vi "myRIO_BRig_RT_v0,60.vi"() -> ()   [LabVIEW 2014]
uses:
  myRIO_BRig_RT__Case_Exp_stateList.ctl
  myRIO_BRig_RT__Case_NonExp_stateList.ctl
  <vilib>/Platform/TimedLoop/XDataNode/timing_clust.ctl
  <vilib>/Platform/TimedLoop/XDataNode/nitl_modes.ctl
  <vilib>/Platform/TimedLoop/XDataNode/wakeup.ctl
  <vilib>/WebDAVClient/Advanced/SessionHandle.ctl
  <vilib>/myRIO/Common/Instrument Driver Framework/myRIO v1.0/UART/vis/myRIO v1.0 Close UART.vi
  <vilib>/FPGAPlugInAG/myRIO-1900/niLvFpga_Open_myRIO-1900.vi
  <vilib>/rvi/interface/common/dynamic/niFpgaDynamicAddResources.vi
  <vilib>/Utility/error.llb/Error Cluster From Error Code.vi
  <vilib>/rvi/errors/niLvFpgaAdjustHostInterfaceError.vi
  <vilib>/FPGAPlugInAG/Dynamic/niLvFpga_Close_Dynamic.vi
  <vilib>/myRIO/Common/Instrument Driver Framework/Utilities/vis/FPGA Ref Manager.vi
  <vilib>/myRIO/Common/Instrument Driver Framework/myRIO v1.0/myRIO v1.0 Reset FPGA.vi
  <vilib>/myRIO/Common/Instrument Driver Framework/myRIO v1.0/IRQ/vis/myRIO v1.0 IRQ Info FGV.vi
  <vilib>/myRIO/Common/Instrument Driver Framework/myRIO v1.0/IRQ/vis/myRIO v1.0 Timer IRQ Info FGV.vi
  <vilib>/myRIO/Common/Instrument Driver Framework/myRIO v1.0/IRQ/vis/myRIO v1.0 ISR Agent.vi
  <vilib>/rvi/interface/nirviOpenFPGA/nirviOpenFPGA.xnode
  myRIO_BRig_FPGA_v3,51__build.lvbitx
  myRIO_BRig_FPGA_v3,51.vi
  <vilib>/rvi/interface/nirviReadWriteControl/nirviReadWriteControl.xnode
  <vilib>/Platform/TimedLoop/XDataNode/XDataNode.xnode
  <vilib>/rvi/interface/nirviCloseFPGA/nirviCloseFPGA.xnode
  <vilib>/Platform/TimedLoop/XDataNode/XDNodeRunTimeDep.lvlib
  <vilib>/rvi/interface/Simulation/niFpgaSimulationCallBeginRW.vi
  <vilib>/myRIO/Instrument Drivers/Utilities/Utilities.lvlib
  <vilib>/WebDAVClient/NI_WebDAV.lvlib
  NiFpgaLv.dll
panel:
  out "SolenoidReward":bool
  in  "SolenoidProbability_L":u16=50 caption="Reward Time [ms]" min=1 max=1000 step=1
  in  "SolenoidProbability_R":u16=50 caption="Reward Time [ms]" min=1 max=1000 step=1
  out "output_PortA":dbl
  out "error out 4":errorcluster
  in  "laser_power_step":dbl
  in  "laser_power_max":dbl
  in  "Recording_p2":bool
  in  "Recording":bool
  out "error out 3":errorcluster
  out "error out 2":errorcluster
  in  "laser_power_min":dbl
  in  "f_millisec2count":dbl=159.0
  in  "laser_Tshutter":dbl=2.0
  in  "laser_Freq":dbl=10.0
  in  "laser_Tpeak":dbl=2.0
  in  "laser_duration":u16
  out "error out":errorcluster
  in  "LC_Cue1_All_Count":u16
  in  "LC_Cue1_First_Count":u16
  in  "LC_Cue1_All_delayOpt":bool
  in  "LC_ENL1_All_delayOpt":bool
  in  "LC_ENL1_All_Count":u16
  in  "LC_ENL1_First_Count":u16
  in  "LC_Cue1_First_delayOpt":bool
  in  "LC_ENL1_First_delayOpt":bool
  in  "Tcycle_Cue_max":u16=1000 caption="Max [ms]" min=5 max=5000 step=5
  in  "Tcycle_Cue_min":u16=1000 caption="Min [ms]" min=5 max=5000 step=5
  in  "SendData":bool
  out "cSpout":enum16{"Left", "Right"}(ring) caption="Left or Right Spout"
  out "A4":u32 caption="LickCounter_Right"
  out "A2":u32 caption="LickCounter_Left"
  in  "laserResponse_wrong_LED":bool
  out "error_initTrial":errorcluster
  out "error_Selection_pre":errorcluster
  out "error_Selection":errorcluster
  out "SelectWrong":bool
  out "SelectReward":bool
  in  "Left(F)_or_Right(T)":bool
  in  "ignoreWrong":bool
  in  "SelectionState":bool
  in  "laserResponse_wrong":bool
  in  "laserResponse_reward":bool
  in  "laserResponse_reward_LED":bool
  out "nRewards_Right":u16 caption="# Rewards Total (Right)"
  out "nRewards_Left":u16 caption="# Rewards Total (Left)"
  out "nRewards_cur":u16 caption="# Rewards in Current Block"
  out "TpB_target":u16 caption="Target Trials Per Block"
  out "cState_NonExp":T1 caption="NonExperimental State"
  out "iBlock":u16 caption="Current Block"
  out "cState":T2 caption="Experimental State"
  out "iTrial":u16 caption="Current Trial"
  in  "warmupType":u8(slide) max=2 step=1 scale=0.0..2.0
  in  "TestConnection":bool
  in  "warmup":bool caption="WarmUp"
  in  "Host Filename Prefix":string="Exp1_TM2"
  out "Connected To Host?":bool
  in  "Host Password":string="sabalab"
  in  "Host UserName":string="Test2"
  in  "sp_RightSpout":u16(slide)=2 max=2 step=1 scale=0.0..2.0
  in  "sp_LeftSpout":u16(slide)=2 max=2 step=1 scale=0.0..2.0
  in  "BUR_max":u16 caption="Count Reward Structure  (0 = off)"
  in  "LC_Wrong_Probability":u16
  in  "LC_Wrong_Trial":u16(slide) max=2 step=1 scale=0.0..2.0
  in  "LC_Wrong_Block":u16(slide) max=2 step=1 scale=0.0..2.0
  in  "LC_Wrong_OnOff":bool
  in  "LC_Reward_Probability":u16
  in  "LC_Reward_Trial":u16(slide) max=2 step=1 scale=0.0..2.0
  in  "LC_Reward_Block":u16(slide) max=2 step=1 scale=0.0..2.0
  in  "LC_Reward_OnOff":bool
  in  "LC_Cue1_All_Probability":u16
  in  "LC_Cue1_All_Block":u16(slide) max=2 step=1 scale=0.0..2.0
  in  "LC_Cue1_All_OnOff":bool
  in  "LC_Cue1_First_Probability":u16
  in  "LC_Cue1_First_Block":u16(slide) max=2 step=1 scale=0.0..2.0
  in  "LC_Cue1_First_OnOff":bool
  in  "LC_ENL1_All_Probability":u16 max=100 step=1
  in  "LC_ENL1_All_Block":u16(slide) max=2 step=1 scale=0.0..2.0
  in  "LC_ENL1_All_OnOff":bool
  in  "LC_ENL1_First_Probability":u16 max=100 step=1
  in  "LC_ENL1_First_Block":u16(slide) max=2 step=1 scale=0.0..2.0
  in  "Tcycle_Timeout":u16=1000 caption="Timeout Time [ms]" min=10 max=10000 step=1
  in  "Tcycle_Wrong":u16=1000 caption="Wrong Time [ms]" min=10 max=10000 step=1
  in  "Tcycle_Selection":u16=1000 caption="Answer Time [ms]" min=1 max=10000 step=1
  in  "Tcycle_RewardPost":u16=1000 caption="Consumption Time [ms]" min=250 max=10000 step=250
  in  "Tcycle_Reward_L":u16=500 caption="Reward Time [ms]" min=1 max=1000 step=1
  in  "Tcycle_Reward_R":u16=500 caption="Reward Time [ms]" min=1 max=1000 step=1
  in  "TpB_Max_R":u16=4 caption="Max TrialsPerBlock" min=1 max=12 step=1
  in  "TpB_Min_R":u16=4 caption="Min TrialsPerBlock" min=1 max=12 step=1
  in  "TpB_Max_L":u16=4 caption="Max TrialsPerBlock" min=1 max=12 step=1
  in  "TpB_Min_L":u16=4 caption="Min TrialsPerBlock" min=1 max=12 step=1
  in  "BUR_min":u16 caption="Count Reward Structure  (0 = off)"
  in  "TrialUntilReward":bool caption="Ignore Wrong \nSelection"
  in  "CueCycles":u16=1 caption="Cue Structure" min=1 max=1 step=1
  in  "MTrig_Laser_Tcycle":u16=10 caption="Time [ms]"
  in  "MTrig_Laser_trig":bool
  in  "MTrig_Audio_trig__R":bool caption="Trigger Audio"
  in  "MTrig_Audio_trig__L":bool caption="Trigger Audio"
  in  "RewCalib_Trig_R":bool caption="Calibrate_R"
  in  "RewCalib_Trig_L":bool caption="Calibrate_L"
  in  "MTrig_Solenoid_Tcycle__R":u16=300 caption="Time [ms]"
  in  "MTrig_Solenoid_Tcycle__L":u16=300 caption="Time [ms]"
  in  "MTrig_Solenoid_trig__R":bool caption="Solenoid"
  in  "MTrig_Solenoid_trig__L":bool caption="Solenoid"
  in  "STOP_abort":bool caption="Stop LabView\n(Stops myRio and FPGA)"
  in  "STOP_endBlock":bool caption="Stop Experiment\n@ End of Block"
  in  "STOP_endTrial":bool caption="Stop Experiment\n@ End of Trial"
  in  "START":bool caption="Start Experiment"
  in  "Tcycle_CuePenalty":u16=1000 caption="Penalty [ms]" min=1 max=10000 step=1
  in  "Audio_Amp__R":u16=100 caption="Amp"
  in  "Audio_Freq__R":u8=5 caption="Freq [kHz]" max=14 step=1
  in  "Audio_Amp__L":u16=100 caption="Amp"
  in  "Audio_Freq__L":u8=5 caption="Freq [kHz]" max=14 step=1
  in  "LC_Wrong_Tdelay":u16
  in  "LC_Cue1_All_Tdelay":u16
  in  "LC_ENL1_All_Tdelay":u16
  in  "LC_Reward_Tdelay":u16
  in  "LC_Cue1_First_Tdelay":u16
  in  "LC_ENL1_First_Tdelay":u16
  in  "LC_ENL1_First_OnOff":bool
  in  "Tcycle_ENLPenalty":u16=100 caption="Penalty [ms]" min=10 max=10000 step=10
  in  "Tcycle_ENL_max":u16=1000 caption="Max [ms]" min=250 max=10000 step=250
  in  "Tcycle_ENL_min":u16=1000 caption="Min [ms]" min=250 max=10000 step=250
  # "Manual Control"
  # "Task Structure"
  # "Task Timing"
  # "Laser Control\n\n                                                    On/Off      Block        Probability [%]   Delay [ms]                              Count"
  # "Manual Solenoid Trigger\nLeft              Right"
  # "Master Structure"
  # "Enforced NonLick"
  # "Enforced NonLick 1"
  # "from end"
  # "Time = Cue Min"
  # "Min\n \n  \nMax"
  # "Switch Trial"
  # "from start"
  # "(1) = Switching\n(2) = Two Choice"
  # "from end"
  # "NonSwitch Trials"
  # "Cue"
  # "from start"
  # "Cue 1"
  # "from end"
  # "Switch Trial"
  # "from start"
  # "Min"
  # "Max"
  # "from end"
  # "NonSwitch Trials"
  # "Trial Per Block Structure\n       Left                    Right"
  # "from start"
  # "Spout Selection Control"
  # "Manual Speaker Trigger\nLeft              Right"
  # "Selection Reward"
  # "Answer Time\n         [ms]\n\n  \nWrong Choice Penalty\n         [ms]\n \n \nChoice Timeout Penalty\n         [ms]"
  # "Selection Wrong"
  # "Cue Control"
  # "Left              Right"
  # "State"
  # "Manual Laser Trigger"
  # "Freq [kHz]\n \n \nAmp\n \n\n \n\nSpeaker\nSetting"
  # "Reward Control\n                 Left              Right"
  # "Min = 1\nMax = 32k"
  # "Reward Time\n         [ms]\n\nWater Prob"
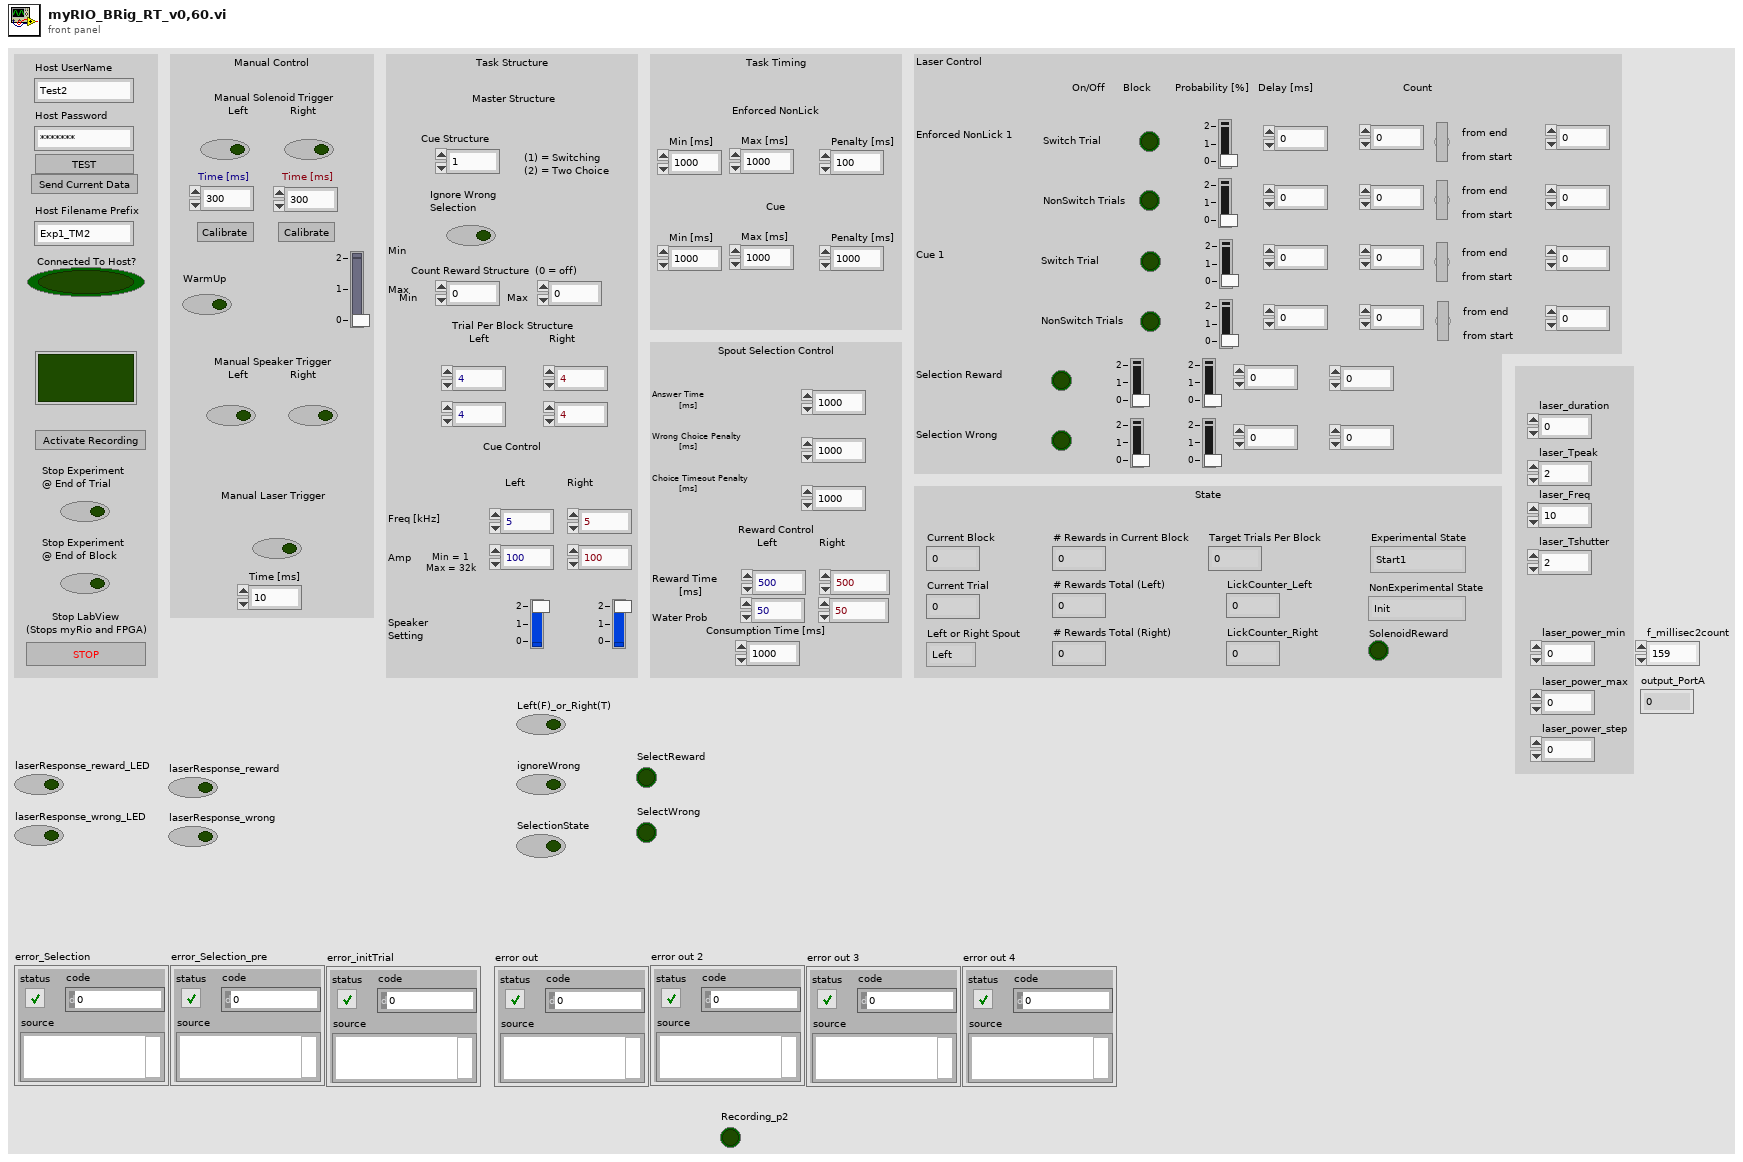
[diagram p1: front panel]
types:
  T1 = typedef "myRIO_BRig_RT__Case_NonExp_stateList.ctl" = enum16{"Init", "UploadSettings_pre", "UploadSettings_Read_dataExp", "UploadSettings_dataExp_1", "UploadSettings_Read_dataLC", "UploadSettings_dataLC_1", "UploadSettings_dataLC_2", "UploadSettings_Read_dataMTrig", "UploadSettings_dataMTrig_1", "UploadSettings_post", "Idle_pre", "IdleEmpty", "IdleEmpty2", "IdleEmpty3", "IdleEmpty4", "Idle", "Idle_2", "Idle_3", "Idle_4", "Idle_post", "Cue_pre__pre", "Cue_pre", "Cue", "Cue_post", "RewardCalibration_pre", "DispenseWater_pre__pre", "DispenseWater_pre", "DispenseWater", "DispenseWater_post", "TestConnection", "SendData", "End"}
  T2 = typedef "myRIO_BRig_RT__Case_Exp_stateList.ctl" = enum16{"Start1", "Start2", "Start3", "saveSettings1", "saveSettings2", "saveSettings3", "saveSettings4_LC_ENL", "saveSettings5_LC_Cue", "saveSettings6_LC_Other", "setSettings_Audio", "setSettings_Laser", "initBlock_pre", "initBlock", "initBlock2", "initBlock_post", "initTrial_pre", "initTrial", "initTrial2", "initTrial3", "initTrial4", "initTrial_LC_ENL1", "initTrial_LC_Cue1", "initTrial_post", "ENL1_pre", "ENL1", "ENL1_post", "ENL1Penalty_pre", "ENL1Penalty", "ENL2_pre", "ENL2", "ENL2Penalty_pre", "ENL2Penalty", "Cue1_pre", "Cue1", "Cue1_post", "Cue1Penalty_pre", "Cue1Penalty", "Cue2_pre", "Cue2", "Cue2Penalty_pre", "Cue2Penalty", "Selection_pre", "Selection", "Select_post", "SelectReward_pre", "SelectReward", "SelectRewardPost_pre", "SelectRewardPost", "SelectWrong_pre", "SelectWrong", "SelectWrong_post", "SelectTimeout_pre", "SelectTimeout", "SelectTimeout_post", "endTrial_pre", "endTrial1", "endTrial2", "endTrial3", "endTrial_post", "endBlock_pre", "endBlock", "endBlock_post", "endExp", "commConnect", "commUpload_pre", "commUpload_dataBlock", "commUpload_dataCurrent", "commUpload_dataExp", "commUpload_dataLC", "commUpload_dataTrial", "commUpload_post", "saveData_pre", "saveData_dataBlock", "saveData_dataCurrent", "saveData_dataExp", "saveData_dataLC", "saveData_dataTrial", "saveData_post", "empty_endBlock1", "empty_endBlock2", "empty_endTrial1", "empty_endTrial2", "empty_endTrial3", "empty_endTrial4", "empty_endTrial5"}
  T3 = typedef "XDNodeRunTimeDep.lvlib/timing_clust.ctl" = cluster{"Expected End [f-1]":u64, "Actual End [f-1]":u64, "Finished Late? [f-1]":bool, "Expected End [i-1]":u64, "Actual End [i-1]":u64, "Finished Late? [i-1]":bool, "Expected Start [i]":u64, "Actual Start [i]":u64, "Expected Start [f]":u64, "Actual Start [f]":u64, "Source Name":string, "Structure Name":string, "Period":i64, "Deadline":i64, "Offset":i64, "Start":i64, "Priority":i32, "Timeout":i32, "Mode":T4, "Wakeup Reason":T5, "Error":errorcluster, "Source Type":string, "Secondary Source Type":string, "Global End Time":u64, "Global Start Time":u64, "Frame Duration":u64, "Iteration Duration":u64, "Assigned CPU":i32, "I/O Scan Engine Mode":u32}
  T4 = typedef "XDNodeRunTimeDep.lvlib/nitl_modes.ctl" = enum32{"No Change", "Process missed periods, maintain original phase", "Discard missed periods, maintain original phase", "Process missed periods, ignore original phase", "Discard missed periods, ignore original phase"}
  T5 = typedef "XDNodeRunTimeDep.lvlib/wakeup.ctl" = enum32{"Normal", "Aborted", "Asynchronous wakeup", "Timing source error", "Timed loop error", "Timeout"}
  T6 = typedef "NI_WebDAV.lvlib/SessionHandle.ctl" = refnum<k1>
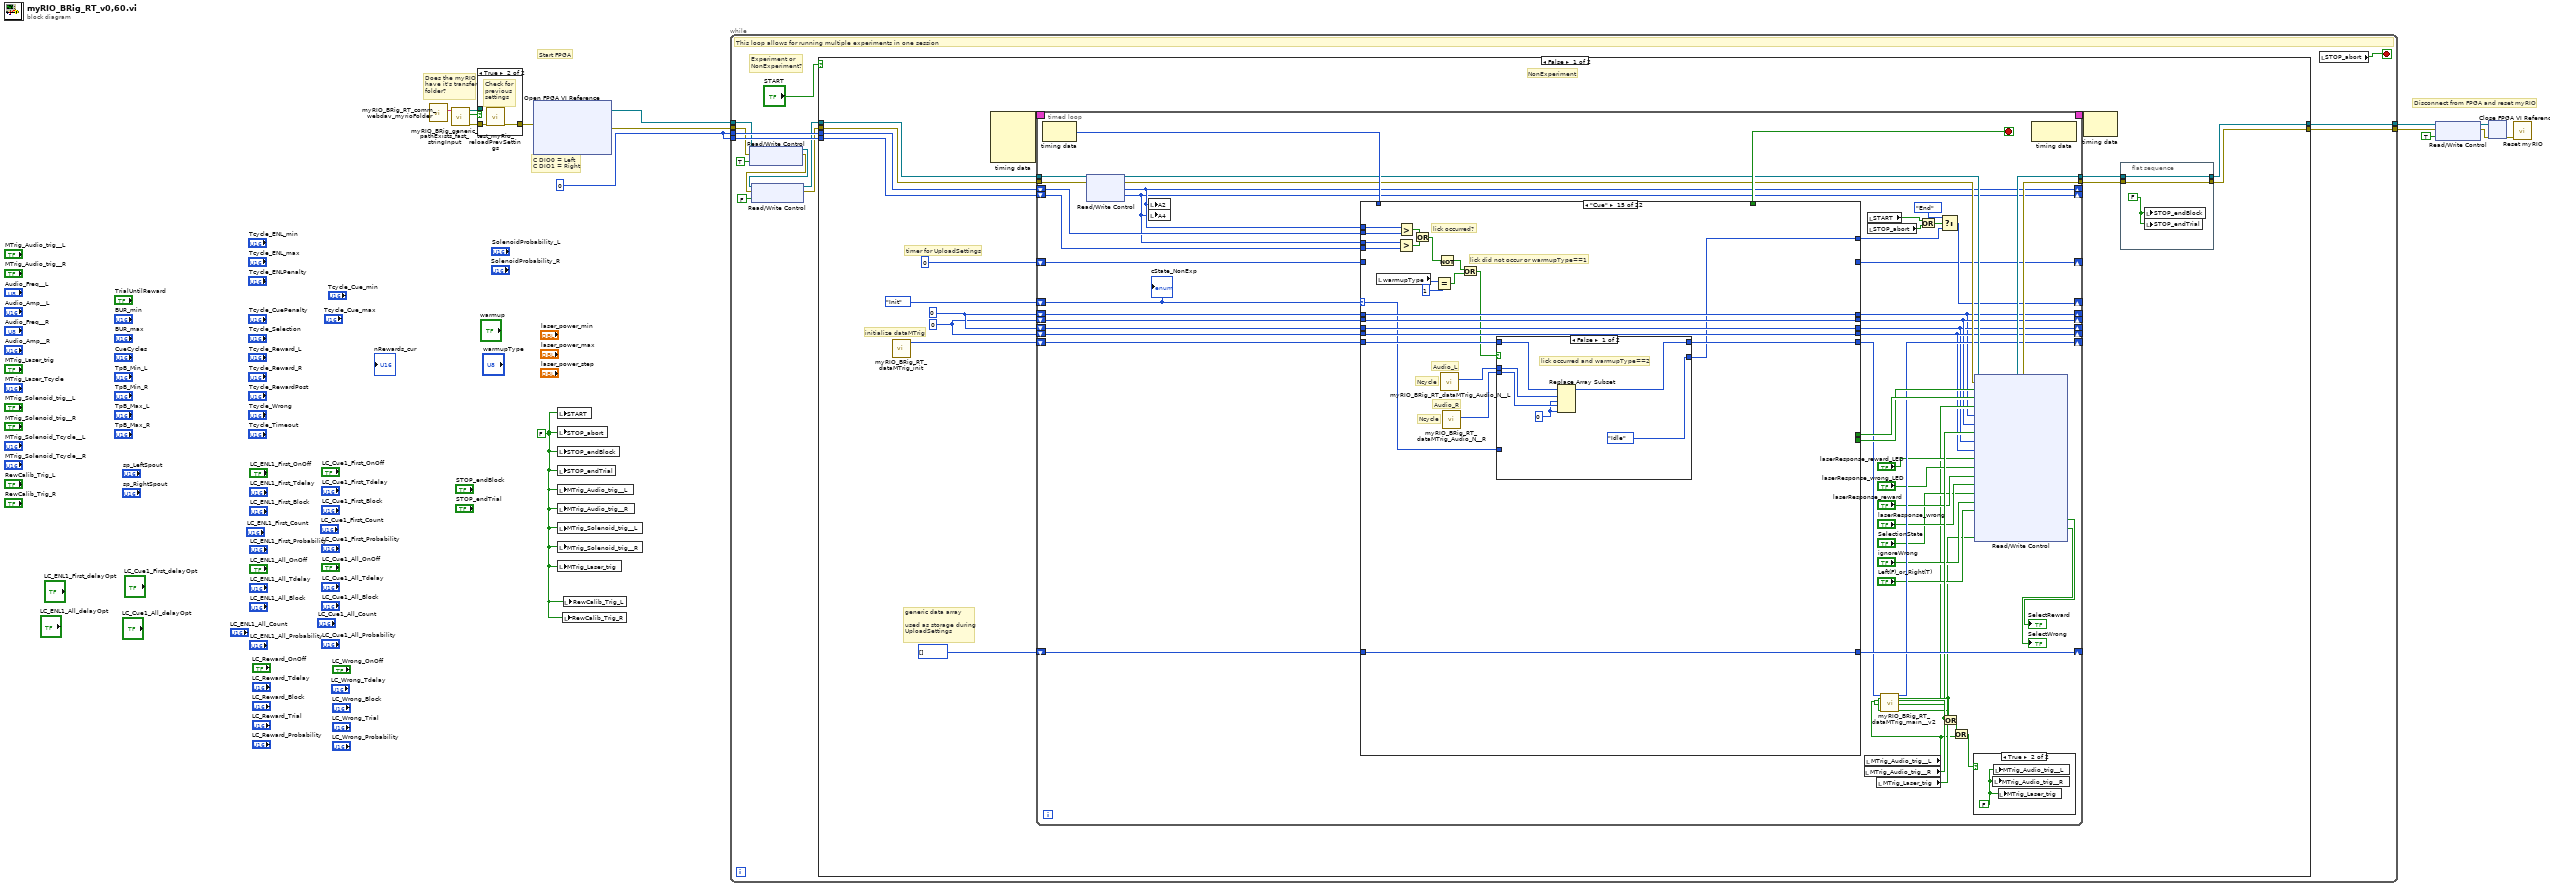
[diagram p0: block diagram]
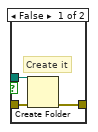
[diagram p2: hidden frame]
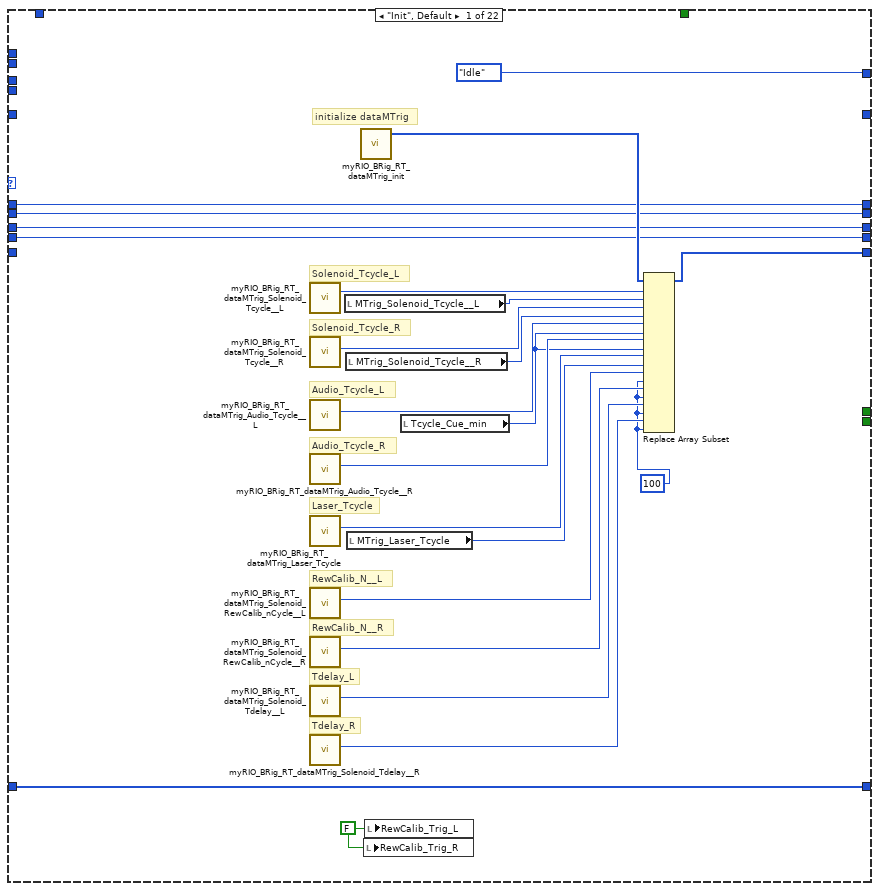
[diagram p4: hidden frame]
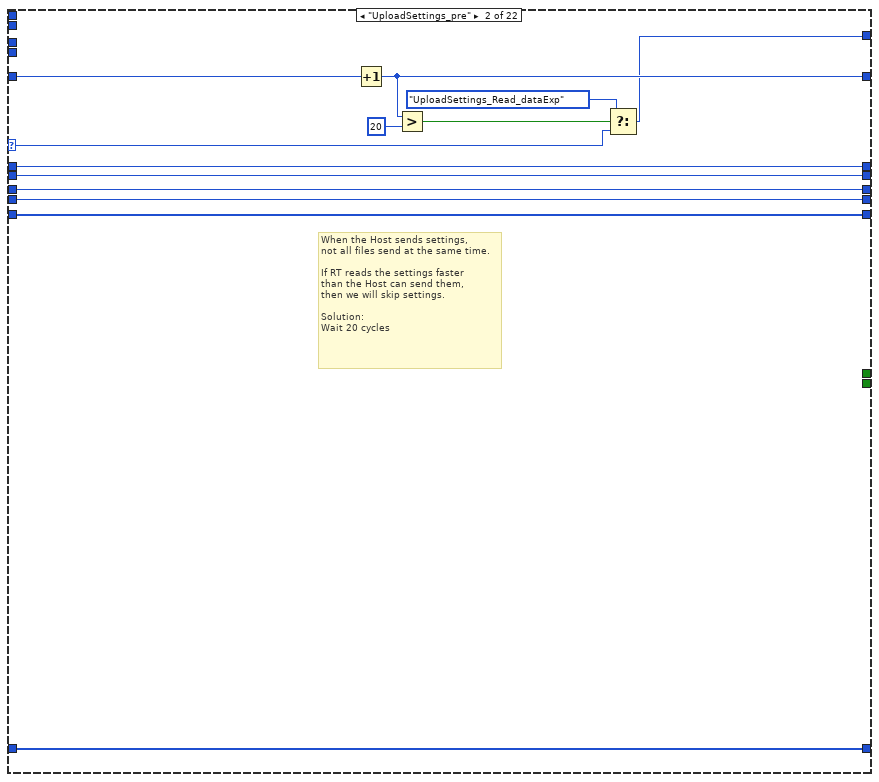
[diagram p5: hidden frame]
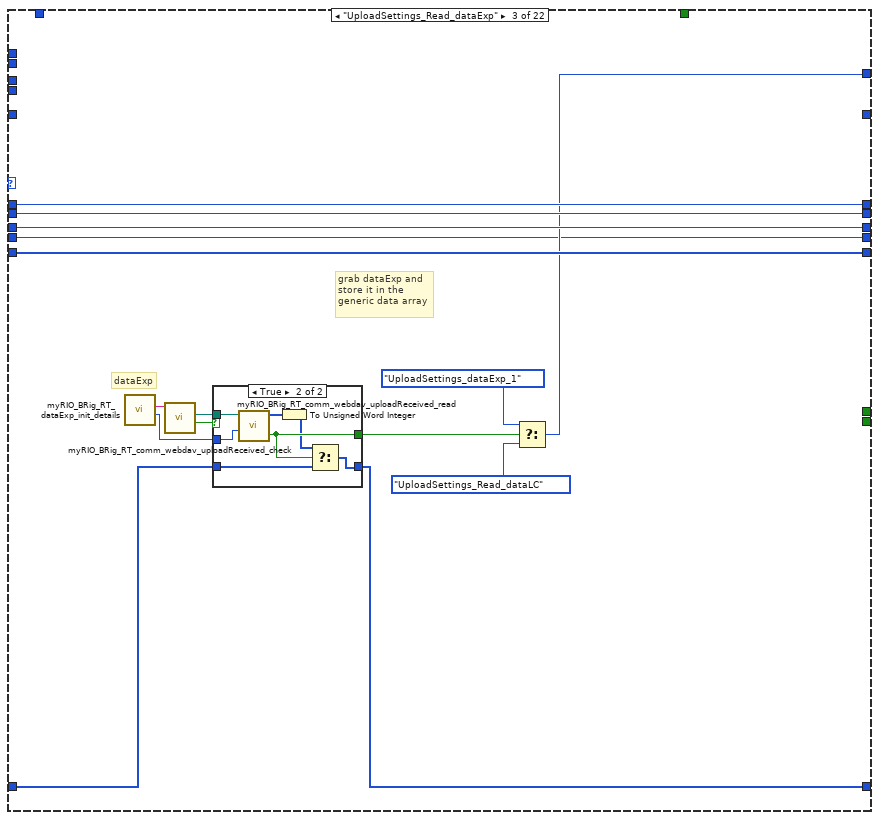
[diagram p6: hidden frame]
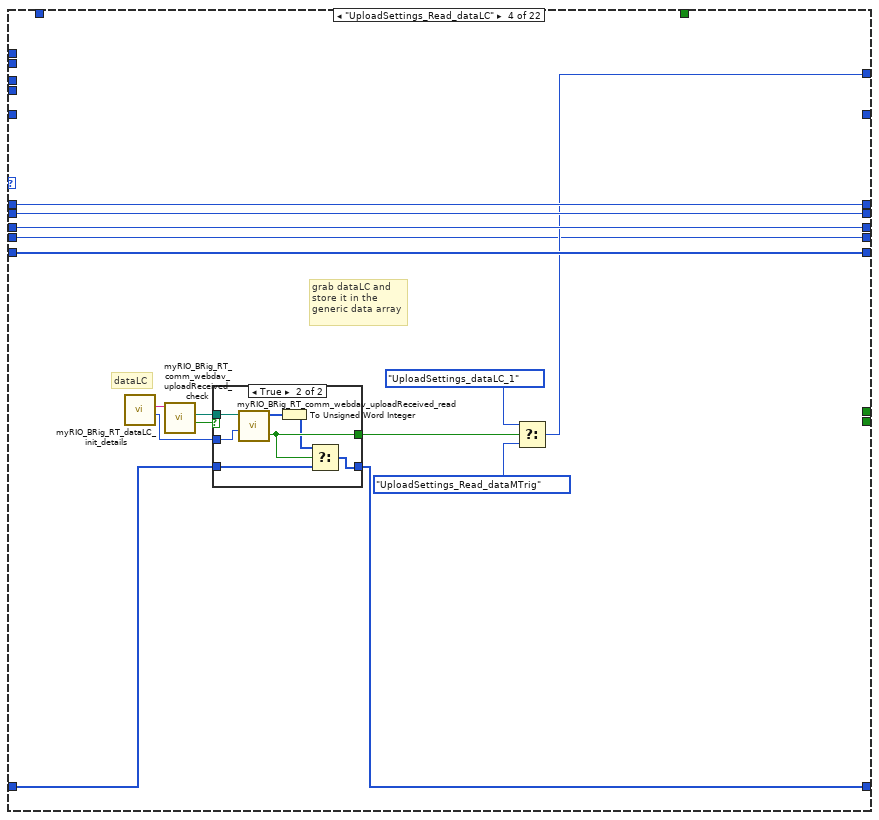
[diagram p8: hidden frame]
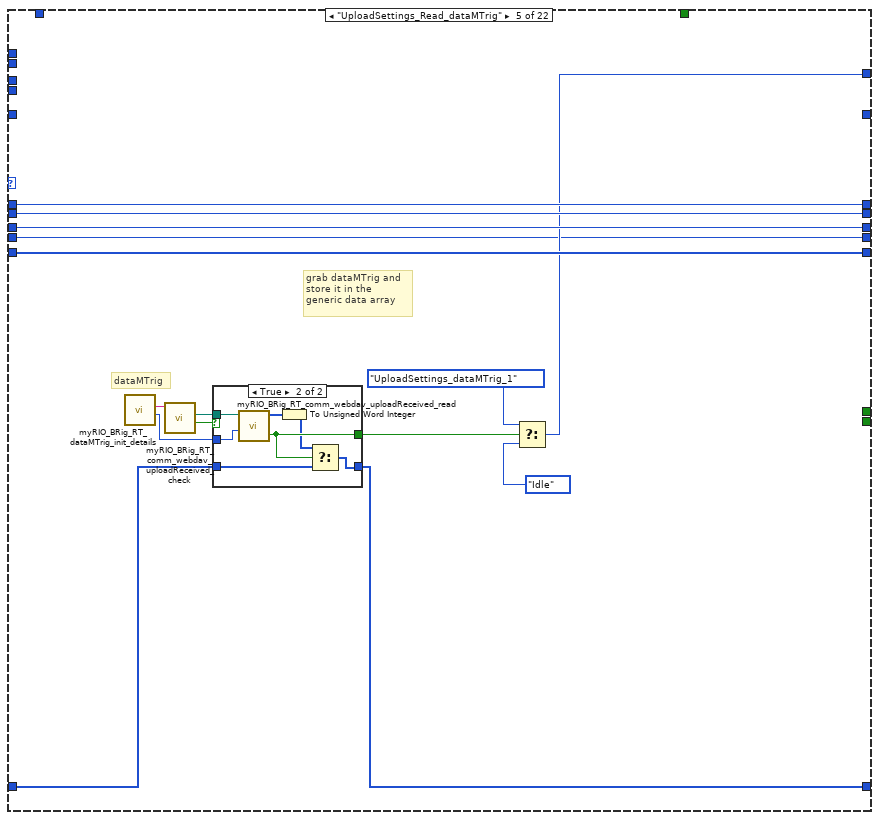
[diagram p10: hidden frame]
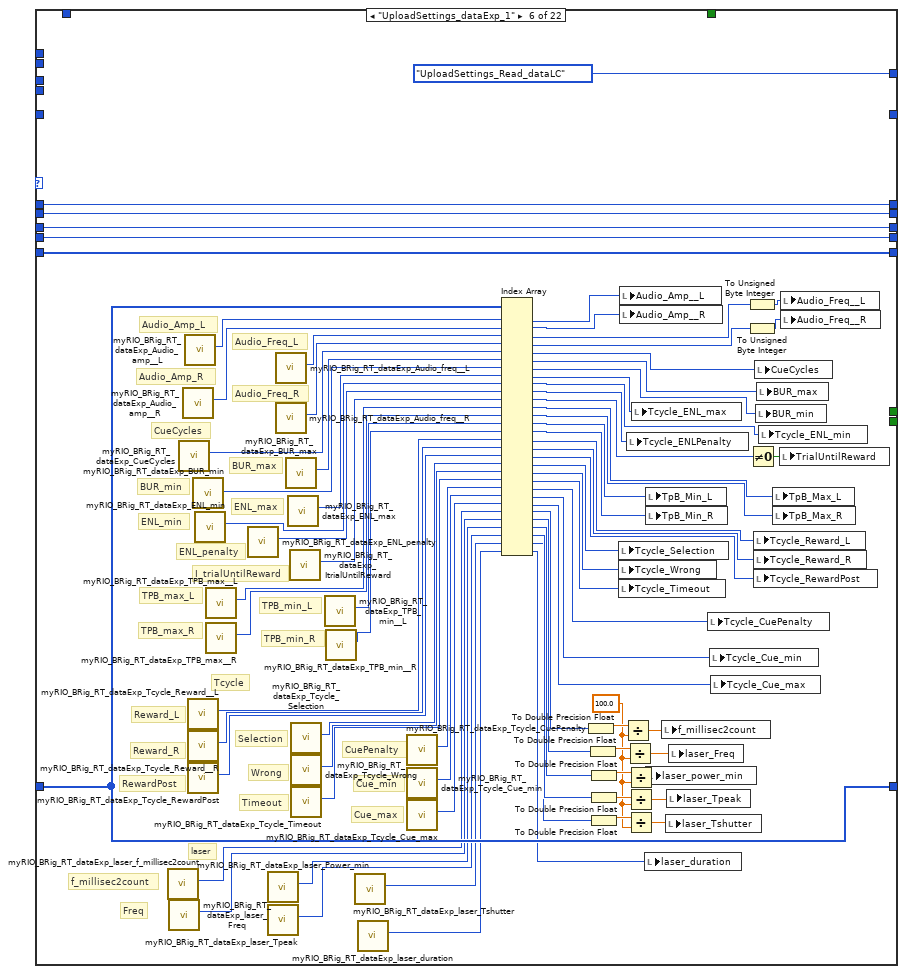
[diagram p12: hidden frame]
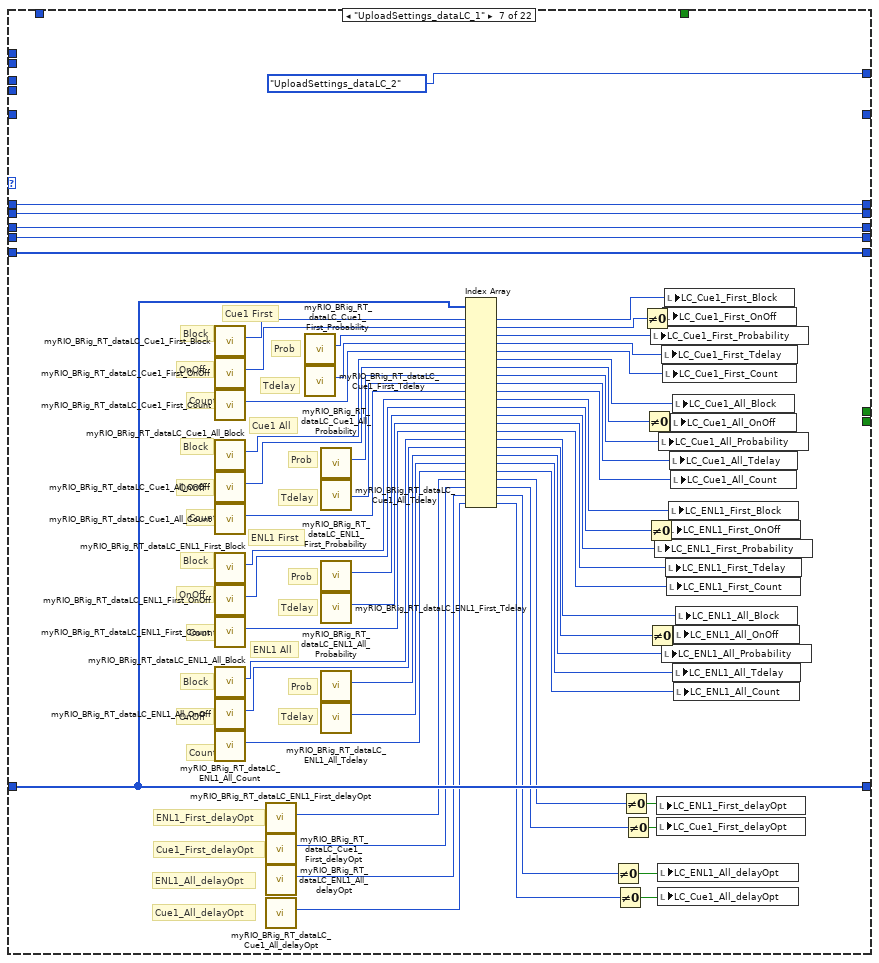
[diagram p13: hidden frame]
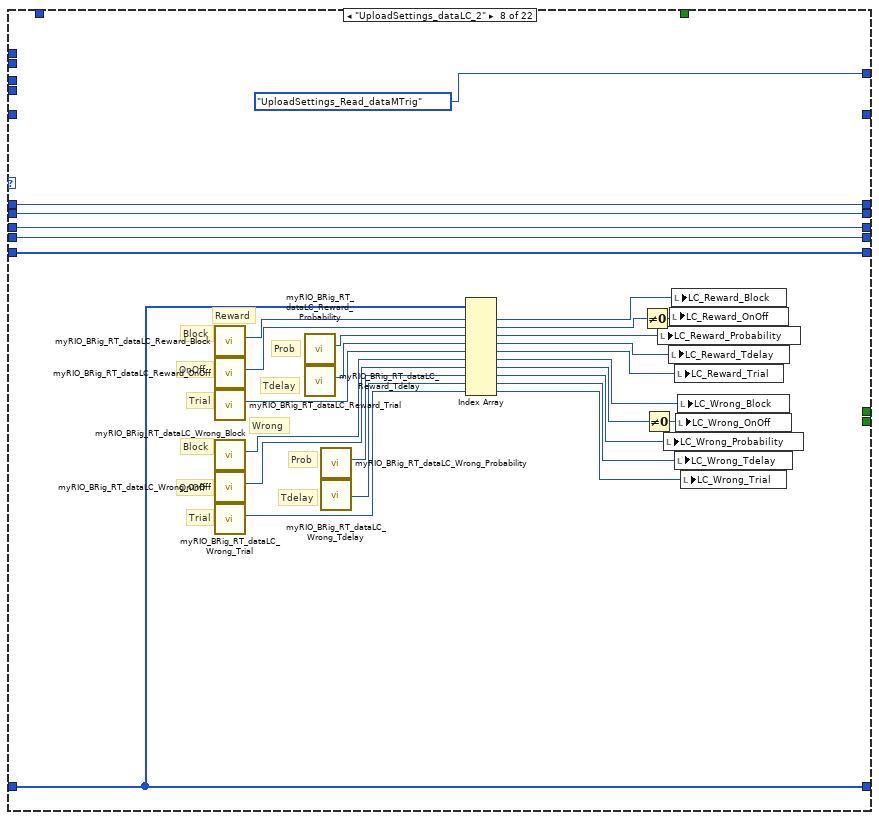
[diagram p14: hidden frame]
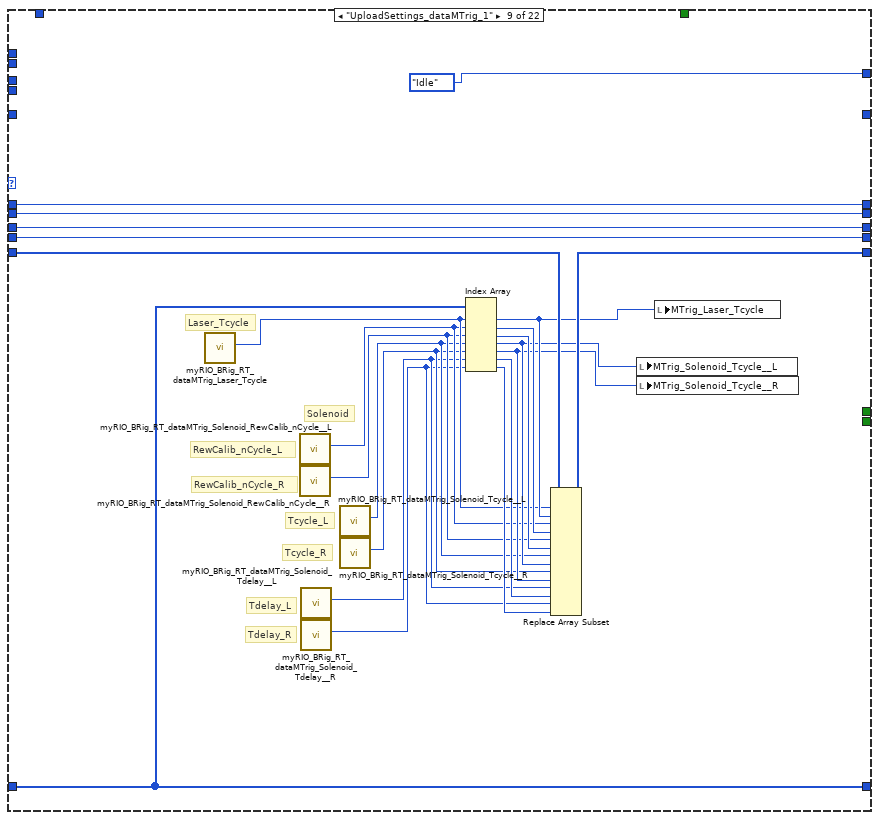
[diagram p15: hidden frame]
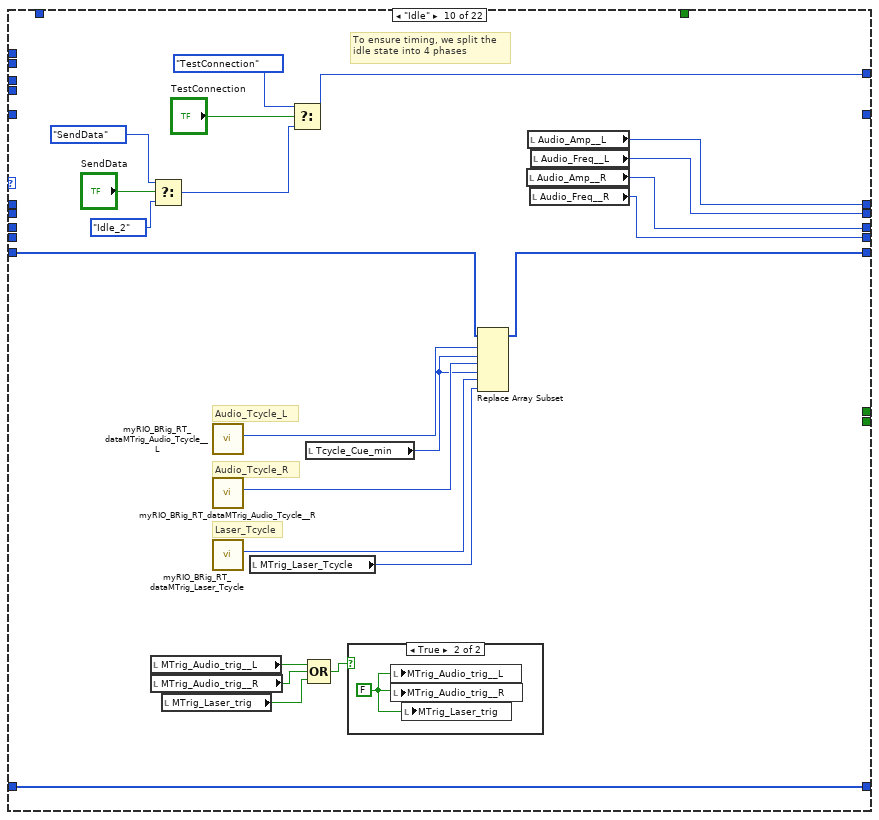
[diagram p16: hidden frame]
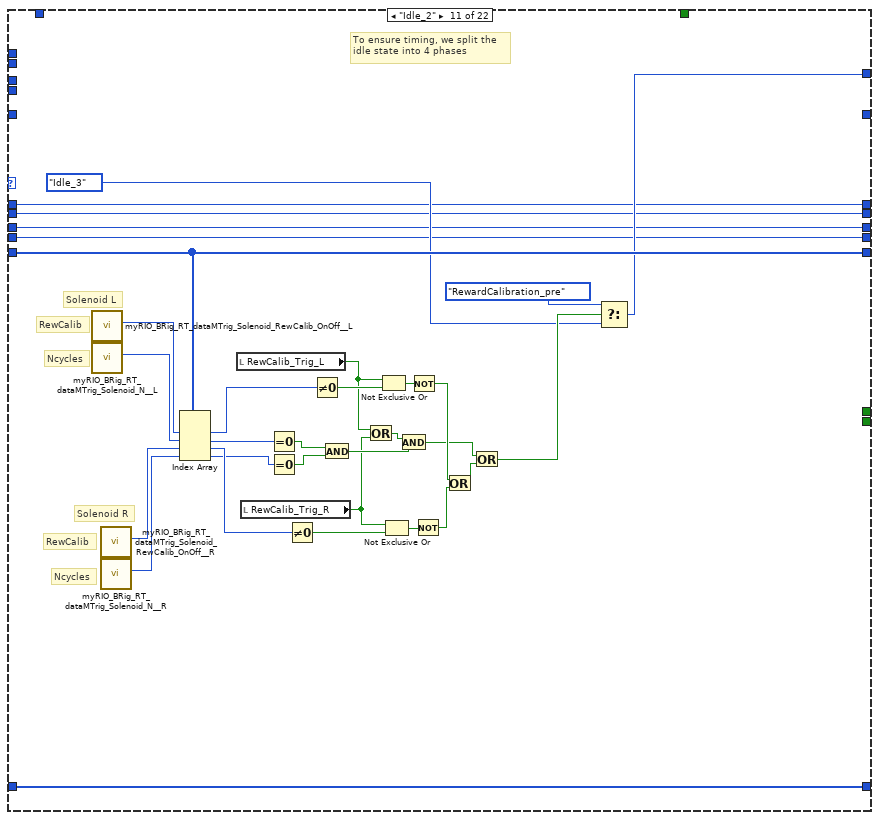
[diagram p18: hidden frame]
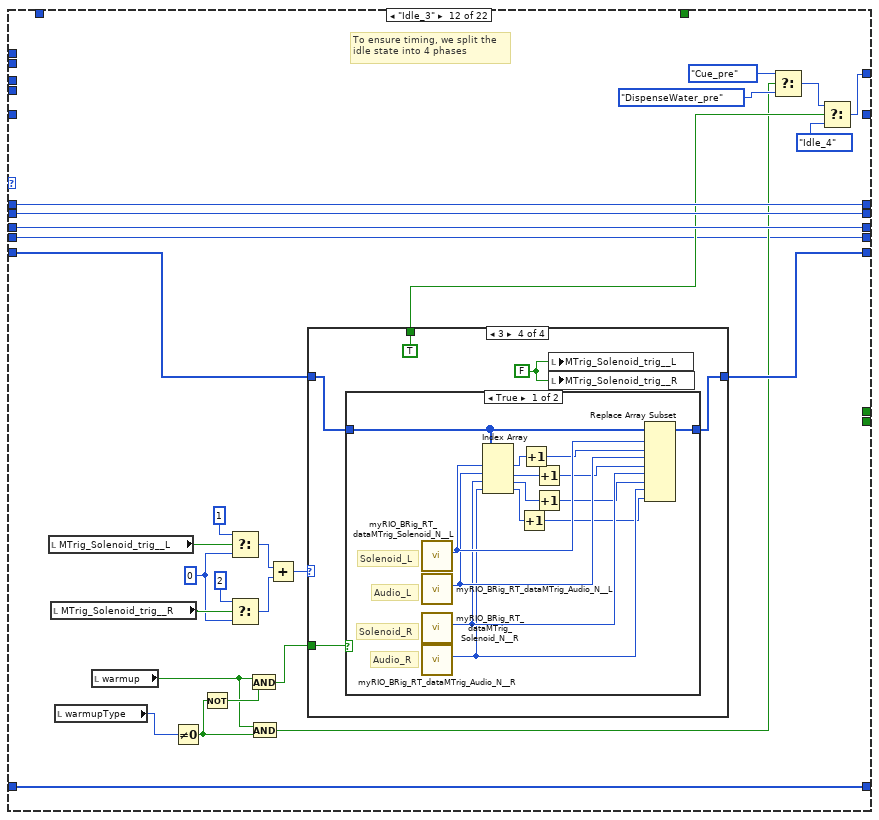
[diagram p19: hidden frame]
diagram:
  w9 = u32 0
  w6 = FALSE
  # "Does the myRIO\nhave it's transfer\nfolder?"
  # "C DIO0 = Left\nC DIO1 = Right"
  # "Start FPGA"
  # "Disconnect from FPGA and reset myRIO"
  n1 = call "myRIO_BRig_RT_comm_webdav_myrioFolder.vi"() -> ("output_myrioFolder"=w4:string)  [unwired: 11 in]
  n2 = call "myRIO_BRig_generic_pathExists_fast_stringInput.vi"("input_filePath"=w4) -> ("output_error"=w3:errorcluster, "output_Iexist"=w2:bool, "output_filePath"=w1:path)  [unwired: 8 in]
  n3 = case shown="True" w2 {
    tunnel: w1 -> [w18 _]
    tunnel: w3 -> [w17 w20]
    tunnel: [w16 w19] -> w5
    frame False {
      # "Create it"
      n4 = Create Folder(path (use dialog)=w18, error in=w17) -> (error out=w16:errorcluster)  [unwired: 1 in, 2 out]
    }
    frame True {
      # "Check for\nprevious\nsettings"
      n5 = call "test_myRio_reloadPrevSettings.vi"("input_error"=w20) -> ("output_error"=w19:errorcluster)  [unwired: 10 in]
    }
  }
  n6 = xnode "Open FPGA VI Reference"("error in"=w5) -> ("FPGA VI Reference Out"=w11:refnum<k20>, "error out"=w10:errorcluster)  [unwired: 1 in]
  n7 = local write "START"(w6) -> ()
  n8 = local write "STOP_abort"(w6) -> ()
  n9 = local write "STOP_endBlock"(w6) -> ()
  n10 = local write "STOP_endTrial"(w6) -> ()
  n11 = local write "MTrig_Audio_trig__L"(w6) -> ()
  n12 = local write "MTrig_Audio_trig__R"(w6) -> ()
  n13 = local write "MTrig_Solenoid_trig__L"(w6) -> ()
  n14 = local write "MTrig_Solenoid_trig__R"(w6) -> ()
  n15 = local write "MTrig_Laser_trig"(w6) -> ()
  n16 = local write "RewCalib_Trig_R"(w6) -> ()
  n17 = local write "RewCalib_Trig_L"(w6) -> ()
  n18 = while {
    tunnel: w11 -> [w24]
    tunnel: w10 -> [w29]
    tunnel: w9 -> [w32]
    tunnel: w9 -> [w31]
    tunnel: [w22] -> w8
    tunnel: [w21] -> w7
    stop <- w30 stop-if-true
    # "Experiment or\nNonExperiment?"
    # "This loop allows for running multiple experiments in one session"
    n19 = xnode "Read/Write Control"("FPGA VI Reference In"=w24, "error in"=w29, "Counts_Reset"=TRUE) -> ("FPGA VI Reference Out"=w26:refnum<k20>, "error out"=w27:errorcluster)
    n20 = xnode "Read/Write Control"("FPGA VI Reference In"=w26, "error in"=w27, "Counts_Reset"=FALSE) -> ("FPGA VI Reference Out"=w23:refnum<k20>, "error out"=w25:errorcluster)
    n21 = case shown="False" "START" {
      tunnel: w32 -> [w46 w958]
      tunnel: w31 -> [w45 w957]
      tunnel: w25 -> [w43 w908]
      tunnel: w23 -> [w44 w907]
      tunnel: [w41 w954] -> w22
      tunnel: [w39 w949] -> w21
      frame False {
        w35 = u8 0 ("Audio_Amp__L")
        w38 = u16 0 ("Audio_Amp__L")
        # "generic data array\n\nused as storage during\nUploadSettings"
        # "timer for UploadSettings"
        # "initialize dataMTrig"
        # "NonExperiment"
        n22 = call "myRIO_BRig_RT_dataMTrig_init.vi"() -> ("output_dataMTrig"=w47:u16[])  [unwired: 5 in]
        n23 = node-c288() -> (w50:T3)  [unwired: 4 in]
        n24 = timed-loop {
          timing: w50 -> [_]
          timing-out: [_] -> w49
          shift-right: [w88] -> _
          shift-left: w47 -> [w105]
          shift-right: [w77] -> _
          shift-left: myRIO_BRig_RT__Case_NonExp_stateList."Init" ("Enum") -> [w97]
          shift-right: [w56] -> _
          shift-left: w46 -> [w57]
          shift-right: [w54] -> _
          shift-left: w45 -> [w55]
          tunnel: [w100] -> w42
          tunnel: [w98] -> w40
          tunnel: w43 -> [w103]
          tunnel: w44 -> [w102]
          shift-right: [w96] -> _
          shift-left: u16[] [] ("output_data") -> [w95]
          shift-right: [w58] -> _
          shift-left: w38 -> [w94]
          shift-right: [w60] -> _
          shift-left: w35 -> [w93]
          shift-right: [w59] -> _
          shift-left: w38 -> [w92]
          shift-right: [w61] -> _
          shift-left: w35 -> [w62]
          shift-right: [w63] -> _
          shift-left: u16 0 ("Audio_Amp__L") -> [w64]
          stop <- w106 stop-if-true
          n25 = node-c288() -> (w104:i64)  [unwired: 1 in]
          n26 = xnode "Read/Write Control"("FPGA VI Reference In"=w102, "error in"=w103) -> ("FPGA VI Reference Out"=w101:refnum<k20>, "error out"=w99:errorcluster, "A2_LickL"=w56:u32, "A4_LickR"=w54:u32)
          n27 = local write "A2"(w56) -> ()
          n28 = local write "A4"(w54) -> ()
          n29 = case shown="\"Cue\"" w97 {
            selector: w97 -> [_ w139 _ _ _ _ _ _ _ _ _ _ _ _ w596 _ _ w802 _ _ _ w898]
            tunnel: [myRIO_BRig_RT__Case_NonExp_stateList."Idle" ("Enum") w137 w145 w168 w191 myRIO_BRig_RT__Case_NonExp_stateList."UploadSettings_Read_dataLC" ("Enum") myRIO_BRig_RT__Case_NonExp_stateList."UploadSettings_dataLC_2" ("Enum") myRIO_BRig_RT__Case_NonExp_stateList."UploadSettings_Read_dataMTrig" ("f") myRIO_BRig_RT__Case_NonExp_stateList."Idle" ("Enum") w421 w437 w473 w562 myRIO_BRig_RT__Case_NonExp_stateList."Cue" ("t") w589 myRIO_BRig_RT__Case_NonExp_stateList."DispenseWater_pre" ("Enum") w743 w800 w827 myRIO_BRig_RT__Case_NonExp_stateList."Idle" ("Enum") myRIO_BRig_RT__Case_NonExp_stateList."Idle" ("Enum") w898] -> w78
            tunnel: [w122 w133 w155 w178 w201 w293 w356 w385 w405 w427 w452 w482 w560 w579 w597 w652 w780 w807 w838 w880 w890 w896] -> w89
            tunnel: [_ _ _ _ _ _ _ _ _ _ _ _ _ _ _ _ _ _ _ _ _ TRUE] -> w106
            tunnel: w105 -> [_ w133 w155 w178 w201 w293 w356 w385 w406 w426 w452 w483 w560 w580 w598 w638 w776 w808 w839 w880 w890 w896]
            tunnel: w104 -> [_ _ _ _ _ _ _ _ _ _ _ _ _ _ _ _ _ w812 _ _ _ _]
            tunnel: [w112 w132 w146 w169 w192 w239 w309 w358 w387 w416 w433 w467 w556 w567 w606 w630 w728 w785 w820 w869 w885 w892] -> w96
            tunnel: w95 -> [w112 w132 w147 w170 w193 w239 w309 w358 w387 w416 w433 w467 w556 w567 w606 w630 w728 w785 w820 w869 w885 w892]
            tunnel: [w115 w135 w157 w180 w203 w290 w354 w360 w403 w409 w435 w477 w558 w586 w610 w632 w782 w817 w844 w871 w887 w894] -> w60
            tunnel: [w116 w136 w158 w181 w204 w291 w355 w361 w404 w423 w436 w476 w557 w588 w609 w633 w783 w818 w845 w872 w888 w895] -> w58
            tunnel: [w114 w134 w156 w179 w202 w289 w353 w359 w402 w422 w434 w478 w559 w585 w611 w631 w781 w816 w843 w870 w886 w893] -> w59
            tunnel: w94 -> [w116 w136 w158 w181 w204 w291 w355 w361 w404 _ w436 w476 w557 w588 w609 w633 w783 w818 w845 w872 w888 w895]
            tunnel: w93 -> [w115 w135 w157 w180 w203 w290 w354 w360 w403 _ w435 w477 w558 w586 w610 w632 w782 w817 w844 w871 w887 w894]
            tunnel: w92 -> [w114 w134 w156 w179 w202 w289 w353 w359 w402 _ w434 w478 w559 w585 w611 w631 w781 w816 w843 w870 w886 w893]
            tunnel: [_ _ _ _ _ _ _ _ _ _ _ _ _ _ _ _ _ w809 _ _ _ _] -> w91
            tunnel: [_ _ _ _ _ _ _ _ _ _ _ _ _ _ _ _ _ w791 _ _ _ _] -> w90
            tunnel: w64 -> [_ w143 _ _ _ _ _ _ _ _ _ _ _ _ _ _ _ _ _ _ _ _]
            tunnel: [_ w142 _ _ _ _ _ _ _ _ _ _ _ _ _ _ _ _ _ _ _ _] -> w63
            tunnel: w62 -> [w108 w131 w144 w167 w190 w213 w294 w357 w386 _ w432 w466 w555 w566 w605 w629 w727 w784 w819 w868 w881 w891]
            tunnel: [w108 w131 w144 w167 w190 w213 w294 w357 w386 w408 w432 w466 w555 w566 w605 w629 w727 w784 w819 w868 w881 w891] -> w61
            tunnel: w57 -> [_ _ _ _ _ _ _ _ _ _ _ _ _ _ w602 _ _ _ _ _ _ _]
            tunnel: w56 -> [_ _ _ _ _ _ _ _ _ _ _ _ _ _ w603 _ _ _ _ _ _ _]
            tunnel: w55 -> [_ _ _ _ _ _ _ _ _ _ _ _ _ _ w600 _ _ _ _ _ _ _]
            tunnel: w54 -> [_ _ _ _ _ _ _ _ _ _ _ _ _ _ w601 _ _ _ _ _ _ _]
            frame "Init", Default {
              w113 = FALSE ("RewCalib_Trig_L")
              w109 = u16 100 ("new element/subarray")
              # "Tdelay_R"
              # "Tdelay_L"
              # "RewCalib_N__R"
              # "RewCalib_N__L"
              # "Solenoid_Tcycle_R"
              # "Solenoid_Tcycle_L"
              # "Laser_Tcycle"
              # "Audio_Tcycle_R"
              # "Audio_Tcycle_L"
              # "initialize dataMTrig"
              n30 = call "myRIO_BRig_RT_dataMTrig_Solenoid_Tcycle__L.vi"() -> ("output_Solenoid_Tcycle__L"=w124:i32)  [unwired: 11 in]
              n31 = call "myRIO_BRig_RT_dataMTrig_Solenoid_Tcycle__R.vi"() -> ("output_Solenoid_Tcycle__R"=w125:i32)  [unwired: 11 in]
              n32 = call "myRIO_BRig_RT_dataMTrig_Audio_Tcycle__L.vi"() -> ("output_Audio_Tcycle__L"=w126:i32)  [unwired: 11 in]
              n33 = call "myRIO_BRig_RT_dataMTrig_Audio_Tcycle__R.vi"() -> ("output_Audio_Tcycle__R"=w127:i32)  [unwired: 11 in]
              n34 = call "myRIO_BRig_RT_dataMTrig_Laser_Tcycle.vi"() -> ("output_Laser_Tcycle"=w128:i32)  [unwired: 11 in]
              n35 = call "myRIO_BRig_RT_dataMTrig_Solenoid_RewCalib_nCycle__L.vi"() -> ("output_Solenoid_RewCalib_nCycle__L"=w120:i32)  [unwired: 11 in]
              n36 = call "myRIO_BRig_RT_dataMTrig_Solenoid_RewCalib_nCycle__R.vi"() -> ("output_Solenoid_RewCalib_nCycle__R"=w119:i32)  [unwired: 11 in]
              n37 = call "myRIO_BRig_RT_dataMTrig_Solenoid_Tdelay__L.vi"() -> ("output_Solenoid_Tdelay__L"=w118:i32)  [unwired: 11 in]
              n38 = call "myRIO_BRig_RT_dataMTrig_Solenoid_Tdelay__R.vi"() -> ("output_Solenoid_Tdelay__R"=w117:i32)  [unwired: 11 in]
              n39 = local read "MTrig_Solenoid_Tcycle__L"() -> (w129:u16)
              n40 = local read "MTrig_Solenoid_Tcycle__R"() -> (w130:u16)
              n41 = local read "MTrig_Laser_Tcycle"() -> (w110:u16)
              n42 = call "myRIO_BRig_RT_dataMTrig_init.vi"() -> ("output_dataMTrig"=w123:u16[])  [unwired: 5 in]
              n43 = local write "RewCalib_Trig_R"(w113) -> ()
              n44 = local write "RewCalib_Trig_L"(w113) -> ()
              n45 = local read "Tcycle_Cue_min"() -> (w111:u16)
              n46 = Replace Array Subset(array=w123, new element #1=w129, index #1=w124, new element #2=w130, index #2=w125, new element #3=w111, index #3=w126, new element #4=w111, index #4=w127, new element #5=w110, index #5=w128, new element #6=w109, index #6=w120, new element #7=w109, index #7=w119, new element #8=w109, index #8=w118, new element #9=w109, index #9=w117) -> (w122:u16[])
            }
            frame "UploadSettings_pre" {
              # "When the Host sends settings,\nnot all files send at the same time.\n\nIf RT reads the settings faster\nthan the Host can send them,\nthen we will skip settings.\n\nSolution:\nWait 20 cycles"
              n47 = Increment(x=w143) -> (x+1=w142:u16)
              n48 = Greater?(x=w142, y=u16 20) -> (0:w140:bool)
              n49 = Select(t=myRIO_BRig_RT__Case_NonExp_stateList."UploadSettings_Read_dataExp", s=w140, f=w139) -> (s? t:f=w137:T1)
            }
            frame "UploadSettings_Read_dataExp" {
              # "grab dataExp and\nstore it in the\ngeneric data array"
              # "dataExp"
              n50 = call "myRIO_BRig_RT_dataExp_init_details.vi"() -> ("output_dataSize"=w151:i32, "output_dataName"=w154:string)  [unwired: 10 in]
              n51 = call "myRIO_BRig_RT_comm_webdav_uploadReceived_check.vi"("input_dataName"=w154) -> ("output_Iexist"=w153:bool, "output_dataPath"=w152:path)  [unwired: 9 in]
              n52 = case shown="True" w153 {
                tunnel: w152 -> [_ w166]
                tunnel: w151 -> [_ w165]
                tunnel: [_ w164] -> w150
                tunnel: w147 -> [w159 w163]
                tunnel: [w159 w160] -> w146
                frame False {
                }
                frame True {
                  n53 = call "myRIO_BRig_RT_comm_webdav_uploadReceived_read.vi"("input_dataSize"=w165, "input_filePath"=w166) -> ("output_Ivalid"=w164:bool, "output_data"=w162:i64[])  [unwired: 8 in]
                  n54 = To Unsigned Word Integer(number=w162) -> (unsigned 16bit integer=w161:u16[])
                  n55 = Select(t=w161, s=w164, f=w163) -> (s? t:f=w160:u16[])
                }
              }
              n56 = Select(t=myRIO_BRig_RT__Case_NonExp_stateList."UploadSettings_dataExp_1", s=w150, f=myRIO_BRig_RT__Case_NonExp_stateList."UploadSettings_Read_dataLC" ("t")) -> (s? t:f=w145:T1)
            }
            frame "UploadSettings_Read_dataLC" {
              # "grab dataLC and\nstore it in the\ngeneric data array"
              # "dataLC"
              n57 = call "myRIO_BRig_RT_dataLC_init_details.vi"() -> ("output_dataSize"=w174:i32, "output_dataName"=w177:string)  [unwired: 10 in]
              n58 = call "myRIO_BRig_RT_comm_webdav_uploadReceived_check.vi"("input_dataName"=w177) -> ("output_Iexist"=w176:bool, "output_dataPath"=w175:path)  [unwired: 9 in]
              n59 = case shown="True" w176 {
                tunnel: w175 -> [_ w189]
                tunnel: w174 -> [_ w188]
                tunnel: [_ w187] -> w173
                tunnel: w170 -> [w182 w186]
                tunnel: [w182 w183] -> w169
                frame False {
                }
                frame True {
                  n60 = call "myRIO_BRig_RT_comm_webdav_uploadReceived_read.vi"("input_dataSize"=w188, "input_filePath"=w189) -> ("output_Ivalid"=w187:bool, "output_data"=w185:i64[])  [unwired: 8 in]
                  n61 = To Unsigned Word Integer(number=w185) -> (unsigned 16bit integer=w184:u16[])
                  n62 = Select(t=w184, s=w187, f=w186) -> (s? t:f=w183:u16[])
                }
              }
              n63 = Select(t=myRIO_BRig_RT__Case_NonExp_stateList."UploadSettings_dataLC_1", s=w173, f=myRIO_BRig_RT__Case_NonExp_stateList."UploadSettings_Read_dataMTrig" ("t")) -> (s? t:f=w168:T1)
            }
            frame "UploadSettings_Read_dataMTrig" {
              # "grab dataMTrig and\nstore it in the\ngeneric data array"
              # "dataMTrig"
              n64 = call "myRIO_BRig_RT_dataMTrig_init_details.vi"() -> ("output_dataSize"=w197:i32, "output_dataName"=w200:string)  [unwired: 10 in]
              n65 = call "myRIO_BRig_RT_comm_webdav_uploadReceived_check.vi"("input_dataName"=w200) -> ("output_Iexist"=w199:bool, "output_dataPath"=w198:path)  [unwired: 9 in]
              n66 = case shown="True" w199 {
                tunnel: w198 -> [_ w212]
                tunnel: w197 -> [_ w211]
                tunnel: [_ w210] -> w196
                tunnel: w193 -> [w205 w209]
                tunnel: [w205 w206] -> w192
                frame False {
                }
                frame True {
                  n67 = call "myRIO_BRig_RT_comm_webdav_uploadReceived_read.vi"("input_dataSize"=w211, "input_filePath"=w212) -> ("output_Ivalid"=w210:bool, "output_data"=w208:i64[])  [unwired: 8 in]
                  n68 = To Unsigned Word Integer(number=w208) -> (unsigned 16bit integer=w207:u16[])
                  n69 = Select(t=w207, s=w210, f=w209) -> (s? t:f=w206:u16[])
                }
              }
              n70 = Select(t=myRIO_BRig_RT__Case_NonExp_stateList."UploadSettings_dataMTrig_1", s=w196, f=myRIO_BRig_RT__Case_NonExp_stateList."Idle" ("t")) -> (s? t:f=w191:T1)
            }
            frame "UploadSettings_dataExp_1" {
              w222 = 100.0 ("y")
              # "Freq"
              # "f_millisec2count"
              # "laser"
              # "Cue_max"
              # "Cue_min"
              # "CuePenalty"
              # "Timeout"
              # "Wrong"
              # "Selection"
              # "RewardPost"
              # "Reward_R"
              # "Reward_L"
              # "Tcycle"
              # "TPB_min_R"
              # "TPB_min_L"
              # "TPB_max_R"
              # "TPB_max_L"
              # "I_trialUntilReward"
              # "ENL_penalty"
              # "ENL_min"
              # "ENL_max"
              # "BUR_max"
              # "BUR_min"
              # "CueCycles"
              # "Audio_Freq_R"
              # "Audio_Freq_L"
              # "Audio_Amp_R"
              # "Audio_Amp_L"
              n71 = call "myRIO_BRig_RT_dataExp_laser_f_millisec2count.vi"() -> ("output_laser_f_millisec2count"=w236:i32)  [unwired: 11 in]
              n72 = call "myRIO_BRig_RT_dataExp_laser_Freq.vi"() -> ("output_laser_Freq"=w235:i32)  [unwired: 11 in]
              n73 = call "myRIO_BRig_RT_dataExp_CueCycles.vi"() -> ("output_CueCycles"=w282:i32)  [unwired: 11 in]
              n74 = call "myRIO_BRig_RT_dataExp_Audio_amp__R.vi"() -> ("output_Audio_amp__R"=w286:i32)  [unwired: 11 in]
              n75 = call "myRIO_BRig_RT_dataExp_Audio_amp__L.vi"() -> ("output_Audio_amp__L"=w288:i32)  [unwired: 11 in]
              n76 = call "myRIO_BRig_RT_dataExp_Tcycle_Reward__L.vi"() -> ("output_Tcycle_Reward__L"=w259:i32)  [unwired: 11 in]
              n77 = call "myRIO_BRig_RT_dataExp_Tcycle_Reward__R.vi"() -> ("output_Tcycle_Reward__R"=w258:i32)  [unwired: 11 in]
              n78 = call "myRIO_BRig_RT_dataExp_Tcycle_RewardPost.vi"() -> ("output_Tcycle_RewardPost"=w257:i32)  [unwired: 11 in]
              n79 = call "myRIO_BRig_RT_dataExp_BUR_min.vi"() -> ("output_BUR_min"=w279:i32)  [unwired: 11 in]
              n80 = call "myRIO_BRig_RT_dataExp_ENL_min.vi"() -> ("output_ENL_min"=w275:i32)  [unwired: 11 in]
              n81 = call "myRIO_BRig_RT_dataExp_TPB_max__L.vi"() -> ("output_TPB_max__L"=w267:i32)  [unwired: 11 in]
              n82 = call "myRIO_BRig_RT_dataExp_TPB_max__R.vi"() -> ("output_TPB_max__R"=w266:i32)  [unwired: 11 in]
              n83 = call "myRIO_BRig_RT_dataExp_ENL_penalty.vi"() -> ("output_ENL_penalty"=w274:i32)  [unwired: 11 in]
              n84 = call "myRIO_BRig_RT_dataExp_laser_Power_min.vi"() -> ("output_laser_Power_min"=w234:i32)  [unwired: 11 in]
              n85 = call "myRIO_BRig_RT_dataExp_laser_Tpeak.vi"() -> ("output_laser_Tpeak"=w233:i32)  [unwired: 11 in]
              n86 = call "myRIO_BRig_RT_dataExp_Audio_freq__L.vi"() -> ("output_Audio_freq__L"=w284:i32)  [unwired: 11 in]
              n87 = call "myRIO_BRig_RT_dataExp_Audio_freq__R.vi"() -> ("output_Audio_freq__R"=w283:i32)  [unwired: 11 in]
              n88 = call "myRIO_BRig_RT_dataExp_BUR_max.vi"() -> ("output_BUR_max"=w280:i32)  [unwired: 11 in]
              n89 = call "myRIO_BRig_RT_dataExp_ENL_max.vi"() -> ("output_ENL_max"=w276:i32)  [unwired: 11 in]
              n90 = call "myRIO_BRig_RT_dataExp_ItrialUntilReward.vi"() -> ("output_I_trialUntilReward"=w270:i32)  [unwired: 11 in]
              n91 = call "myRIO_BRig_RT_dataExp_Tcycle_Selection.vi"() -> ("output_Tcycle_Selection"=w256:i32)  [unwired: 11 in]
              n92 = call "myRIO_BRig_RT_dataExp_Tcycle_Wrong.vi"() -> ("output_Tcycle_Wrong"=w255:i32)  [unwired: 11 in]
              n93 = call "myRIO_BRig_RT_dataExp_Tcycle_Timeout.vi"() -> ("output_Tcycle_Timeout"=w254:i32)  [unwired: 11 in]
              n94 = call "myRIO_BRig_RT_dataExp_TPB_min__L.vi"() -> ("output_TPB_min__L"=w265:i32)  [unwired: 11 in]
              n95 = call "myRIO_BRig_RT_dataExp_TPB_min__R.vi"() -> ("output_TPB_min__R"=w264:i32)  [unwired: 11 in]
              n96 = call "myRIO_BRig_RT_dataExp_laser_Tshutter.vi"() -> ("output_laser_Tshutter"=w232:i32)  [unwired: 11 in]
              n97 = call "myRIO_BRig_RT_dataExp_laser_duration.vi"() -> ("output_laser_duration"=w231:i32)  [unwired: 11 in]
              n98 = call "myRIO_BRig_RT_dataExp_Tcycle_CuePenalty.vi"() -> ("output_Tcycle_CuePenalty"=w247:i32)  [unwired: 11 in]
              n99 = call "myRIO_BRig_RT_dataExp_Tcycle_Cue_min.vi"() -> ("output_Tcycle_Cue_min"=w246:i32)  [unwired: 11 in]
              n100 = call "myRIO_BRig_RT_dataExp_Tcycle_Cue_max.vi"() -> ("output_Tcycle_Cue_max"=w245:i32)  [unwired: 11 in]
              n101 = Index Array(array=w239, index #1=w288, index #2=w286, index #3=w284, index #4=w283, index #5=w282, index #6=w280, index #7=w279, index #8=w276, index #9=w275, index #10=w274, index #11=w270, index #12=w267, index #13=w266, index #14=w265, index #15=w264, index #16=w259, index #17=w258, index #18=w257, index #19=w256, index #20=w255, index #21=w254, index #22=w247, index #23=w246, index #24=w245, index #25=w236, index #26=w235, index #27=w234, index #28=w233, index #29=w232, index #30=w231) -> (element #1=w287:u16, element #2=w285:u16, element #3=w242:u16, element #4=w241:u16, element #5=w281:u16, element #6=w278:u16, element #7=w277:u16, element #8=w273:u16, element #9=w272:u16, element #10=w271:u16, element #11=w268:u16, element #12=w263:u16, element #13=w262:u16, element #14=w261:u16, element #15=w260:u16, element #16=w253:u16, element #17=w252:u16, element #18=w251:u16, element #19=w250:u16, element #20=w249:u16, element #21=w248:u16, element #22=w244:u16, element #23=w238:u16, element #24=w237:u16, element #25=w230:u16, element #26=w221:u16, element #27=w220:u16, element #28=w219:u16, element #29=w218:u16, element #30=w214:u16)
              n102 = To Double Precision Float(number=w230) -> (double precision float=w229:dbl)
              n103 = To Double Precision Float(number=w221) -> (double precision float=w227:dbl)
              n104 = To Double Precision Float(number=w220) -> (double precision float=w225:dbl)
              n105 = To Double Precision Float(number=w219) -> (double precision float=w224:dbl)
              n106 = To Double Precision Float(number=w218) -> (double precision float=w223:dbl)
              n107 = local write "Tcycle_Selection"(w250) -> ()
              n108 = local write "Tcycle_Wrong"(w249) -> ()
              n109 = local write "Tcycle_Timeout"(w248) -> ()
              n110 = local write "Audio_Amp__L"(w287) -> ()
              n111 = local write "Audio_Amp__R"(w285) -> ()
              n112 = Divide(x=w229, y=w222) -> (x/y=w228:dbl)
              n113 = Divide(x=w227, y=w222) -> (x/y=w226:dbl)
              n114 = Divide(x=w225, y=w222) -> (x/y=w217:dbl)
              n115 = Divide(x=w224, y=w222) -> (x/y=w216:dbl)
              n116 = Divide(x=w223, y=w222) -> (x/y=w215:dbl)
              n117 = local write "Tcycle_ENLPenalty"(w271) -> ()
              n118 = local write "Tcycle_ENL_max"(w273) -> ()
              n119 = local write "laser_duration"(w214) -> ()
              n120 = local write "TpB_Min_L"(w261) -> ()
              n121 = local write "TpB_Min_R"(w260) -> ()
              n122 = local write "laser_power_min"(w217) -> ()
              n123 = local write "f_millisec2count"(w228) -> ()
              n124 = local write "laser_Tshutter"(w215) -> ()
              n125 = local write "laser_Tpeak"(w216) -> ()
              n126 = local write "laser_Freq"(w226) -> ()
              n127 = local write "Tcycle_CuePenalty"(w244) -> ()
              n128 = local write "Tcycle_Cue_min"(w238) -> ()
              n129 = local write "Tcycle_Cue_max"(w237) -> ()
              n130 = To Unsigned Byte Integer(number=w242) -> (unsigned 8bit integer=w243:u8)
              n131 = To Unsigned Byte Integer(number=w241) -> (unsigned 8bit integer=w240:u8)
              n132 = Not Equal To 0?(x=w268) -> (x != 0?=w269:bool)
              n133 = local write "Tcycle_Reward_L"(w253) -> ()
              n134 = local write "Tcycle_Reward_R"(w252) -> ()
              n135 = local write "Tcycle_RewardPost"(w251) -> ()
              n136 = local write "CueCycles"(w281) -> ()
              n137 = local write "BUR_min"(w277) -> ()
              n138 = local write "BUR_max"(w278) -> ()
              n139 = local write "Tcycle_ENL_min"(w272) -> ()
              n140 = local write "TpB_Max_L"(w263) -> ()
              n141 = local write "TpB_Max_R"(w262) -> ()
              n142 = local write "TrialUntilReward"(w269) -> ()
              n143 = local write "Audio_Freq__L"(w243) -> ()
              n144 = local write "Audio_Freq__R"(w240) -> ()
            }
            frame "UploadSettings_dataLC_1" {
              # "Cue1_All_delayOpt"
              # "ENL1_All_delayOpt"
              # "Cue1_First_delayOpt"
              # "ENL1_First_delayOpt"
              # "ENL1 First"
              # "Cue1 All"
              # "Cue1 First"
              # "Count"
              # "Tdelay"
              # "Prob"
              # "OnOff"
              # "Block"
              # "ENL1 All"
              # "Count"
              # "Tdelay"
              # "Prob"
              # "OnOff"
              # "Block"
              # "Count"
              # "Tdelay"
              # "Prob"
              # "Block"
              # "OnOff"
              # "Count"
              # "Tdelay"
              # "Prob"
              # "OnOff"
              # "Block"
              n145 = call "myRIO_BRig_RT_dataLC_Cue1_First_Block.vi"() -> ("output_Cue1_First_Block"=w351:i32)  [unwired: 11 in]
              n146 = call "myRIO_BRig_RT_dataLC_Cue1_First_OnOff.vi"() -> ("output_Cue1_First_OnOff"=w349:i32)  [unwired: 11 in]
              n147 = call "myRIO_BRig_RT_dataLC_Cue1_First_Count.vi"() -> ("output_Cue1_First_Count"=w346:i32)  [unwired: 11 in]
              n148 = call "myRIO_BRig_RT_dataLC_Cue1_All_Block.vi"() -> ("output_Cue1_All_Block"=w333:i32)  [unwired: 11 in]
              n149 = call "myRIO_BRig_RT_dataLC_Cue1_All_OnOff.vi"() -> ("output_Cue1_All_OnOff"=w332:i32)  [unwired: 11 in]
              n150 = call "myRIO_BRig_RT_dataLC_Cue1_All_Count.vi"() -> ("output_Cue1_All_Count"=w343:i32)  [unwired: 11 in]
              n151 = call "myRIO_BRig_RT_dataLC_ENL1_First_Block.vi"() -> ("output_ENL1_First_Block"=w331:i32)  [unwired: 11 in]
              n152 = call "myRIO_BRig_RT_dataLC_ENL1_First_OnOff.vi"() -> ("output_ENL1_First_OnOff"=w342:i32)  [unwired: 11 in]
              n153 = call "myRIO_BRig_RT_dataLC_ENL1_First_Count.vi"() -> ("output_ENL1_First_Count"=w339:i32)  [unwired: 11 in]
              n154 = call "myRIO_BRig_RT_dataLC_ENL1_All_Block.vi"() -> ("output_ENL1_All_Block"=w338:i32)  [unwired: 11 in]
              n155 = call "myRIO_BRig_RT_dataLC_ENL1_All_OnOff.vi"() -> ("output_ENL1_All_OnOff"=w337:i32)  [unwired: 11 in]
              n156 = call "myRIO_BRig_RT_dataLC_ENL1_All_Count.vi"() -> ("output_ENL1_All_Count"=w334:i32)  [unwired: 11 in]
              n157 = call "myRIO_BRig_RT_dataLC_ENL1_First_delayOpt.vi"() -> ("output_ENL1_First_delayOpt"=w308:i32)  [unwired: 11 in]
              n158 = call "myRIO_BRig_RT_dataLC_Cue1_First_delayOpt.vi"() -> ("output_Cue1_First_delayOpt"=w307:i32)  [unwired: 11 in]
              n159 = call "myRIO_BRig_RT_dataLC_ENL1_All_delayOpt.vi"() -> ("output_ENL1_All_delayOpt"=w300:i32)  [unwired: 11 in]
              n160 = call "myRIO_BRig_RT_dataLC_Cue1_All_delayOpt.vi"() -> ("output_Cue1_All_delayOpt"=w299:i32)  [unwired: 11 in]
              n161 = call "myRIO_BRig_RT_dataLC_Cue1_First_Probability.vi"() -> ("output_Cue1_First_Probability"=w348:i32)  [unwired: 11 in]
              n162 = call "myRIO_BRig_RT_dataLC_Cue1_First_Tdelay.vi"() -> ("output_Cue1_First_Tdelay"=w347:i32)  [unwired: 11 in]
              n163 = call "myRIO_BRig_RT_dataLC_Cue1_All_Probability.vi"() -> ("output_Cue1_All_Probability"=w345:i32)  [unwired: 11 in]
              n164 = call "myRIO_BRig_RT_dataLC_Cue1_All_Tdelay.vi"() -> ("output_Cue1_All_Tdelay"=w344:i32)  [unwired: 11 in]
              n165 = call "myRIO_BRig_RT_dataLC_ENL1_First_Probability.vi"() -> ("output_ENL1_First_Probability"=w341:i32)  [unwired: 11 in]
              n166 = call "myRIO_BRig_RT_dataLC_ENL1_First_Tdelay.vi"() -> ("output_ENL1_First_Tdelay"=w340:i32)  [unwired: 11 in]
              n167 = call "myRIO_BRig_RT_dataLC_ENL1_All_Probability.vi"() -> ("output_ENL1_All_Probability"=w336:i32)  [unwired: 11 in]
              n168 = call "myRIO_BRig_RT_dataLC_ENL1_All_Tdelay.vi"() -> ("output_ENL1_All_Tdelay"=w335:i32)  [unwired: 11 in]
              n169 = Index Array(array=w309, index #1=w351, index #2=w349, index #3=w348, index #4=w347, index #5=w346, index #6=w333, index #7=w332, index #8=w345, index #9=w344, index #10=w343, index #11=w331, index #12=w342, index #13=w341, index #14=w340, index #15=w339, index #16=w338, index #17=w337, index #18=w336, index #19=w335, index #20=w334, index #21=w308, index #22=w307, index #23=w300, index #24=w299) -> (element #1=w350:u16, element #2=w329:u16, element #3=w328:u16, element #4=w327:u16, element #5=w326:u16, element #6=w322:u16, element #7=w321:u16, element #8=w320:u16, element #9=w319:u16, element #10=w318:u16, element #11=w317:u16, element #12=w316:u16, element #13=w315:u16, element #14=w314:u16, element #15=w301:u16, element #16=w313:u16, element #17=w312:u16, element #18=w311:u16, element #19=w310:u16, element #20=w302:u16, element #21=w305:u16, element #22=w303:u16, element #23=w296:u16, element #24=w295:u16)
              n170 = Not Equal To 0?(x=w296) -> (x != 0?=w298:bool)
              n171 = Not Equal To 0?(x=w295) -> (x != 0?=w297:bool)
              n172 = Not Equal To 0?(x=w305) -> (x != 0?=w306:bool)
              n173 = Not Equal To 0?(x=w303) -> (x != 0?=w304:bool)
              n174 = Not Equal To 0?(x=w329) -> (x != 0?=w330:bool)
              n175 = Not Equal To 0?(x=w321) -> (x != 0?=w325:bool)
              n176 = Not Equal To 0?(x=w316) -> (x != 0?=w324:bool)
              n177 = Not Equal To 0?(x=w312) -> (x != 0?=w323:bool)
              n178 = local write "LC_Cue1_First_Probability"(w328) -> ()
              n179 = local write "LC_ENL1_First_Probability"(w315) -> ()
              n180 = local write "LC_ENL1_First_delayOpt"(w306) -> ()
              n181 = local write "LC_Cue1_First_delayOpt"(w304) -> ()
              n182 = local write "LC_ENL1_All_delayOpt"(w298) -> ()
              n183 = local write "LC_Cue1_All_delayOpt"(w297) -> ()
              n184 = local write "LC_Cue1_All_Probability"(w320) -> ()
              n185 = local write "LC_Cue1_First_Tdelay"(w327) -> ()
              n186 = local write "LC_ENL1_All_Probability"(w311) -> ()
              n187 = local write "LC_Cue1_First_OnOff"(w330) -> ()
              n188 = local write "LC_Cue1_First_Count"(w326) -> ()
              n189 = local write "LC_Cue1_First_Block"(w350) -> ()
              n190 = local write "LC_ENL1_First_Tdelay"(w314) -> ()
              n191 = local write "LC_ENL1_First_OnOff"(w324) -> ()
              n192 = local write "LC_ENL1_First_Count"(w301) -> ()
              n193 = local write "LC_ENL1_First_Block"(w317) -> ()
              n194 = local write "LC_Cue1_All_Tdelay"(w319) -> ()
              n195 = local write "LC_Cue1_All_OnOff"(w325) -> ()
              n196 = local write "LC_Cue1_All_Count"(w318) -> ()
              n197 = local write "LC_Cue1_All_Block"(w322) -> ()
              n198 = local write "LC_ENL1_All_Tdelay"(w310) -> ()
              n199 = local write "LC_ENL1_All_OnOff"(w323) -> ()
              n200 = local write "LC_ENL1_All_Count"(w302) -> ()
              n201 = local write "LC_ENL1_All_Block"(w313) -> ()
            }
            frame "UploadSettings_dataLC_2" {
              # "Wrong"
              # "Reward"
              # "Trial"
              # "Tdelay"
              # "Prob"
              # "Block"
              # "OnOff"
              # "Trial"
              # "Tdelay"
              # "Prob"
              # "OnOff"
              # "Block"
              n202 = call "myRIO_BRig_RT_dataLC_Reward_Block.vi"() -> ("output_Reward_Block"=w383:i32)  [unwired: 11 in]
              n203 = call "myRIO_BRig_RT_dataLC_Reward_OnOff.vi"() -> ("output_Reward_OnOff"=w381:i32)  [unwired: 11 in]
              n204 = call "myRIO_BRig_RT_dataLC_Reward_Trial.vi"() -> ("output_Reward_Trial"=w378:i32)  [unwired: 11 in]
              n205 = call "myRIO_BRig_RT_dataLC_Wrong_Block.vi"() -> ("output_Wrong_Block"=w374:i32)  [unwired: 11 in]
              n206 = call "myRIO_BRig_RT_dataLC_Wrong_OnOff.vi"() -> ("output_Wrong_OnOff"=w373:i32)  [unwired: 11 in]
              n207 = call "myRIO_BRig_RT_dataLC_Wrong_Trial.vi"() -> ("output_Wrong_Trial"=w375:i32)  [unwired: 11 in]
              n208 = call "myRIO_BRig_RT_dataLC_Reward_Probability.vi"() -> ("output_Reward_Probability"=w380:i32)  [unwired: 11 in]
              n209 = call "myRIO_BRig_RT_dataLC_Reward_Tdelay.vi"() -> ("output_Reward_Tdelay"=w379:i32)  [unwired: 11 in]
              n210 = call "myRIO_BRig_RT_dataLC_Wrong_Probability.vi"() -> ("output_Wrong_Probability"=w377:i32)  [unwired: 11 in]
              n211 = call "myRIO_BRig_RT_dataLC_Wrong_Tdelay.vi"() -> ("output_Wrong_Tdelay"=w376:i32)  [unwired: 11 in]
              n212 = Index Array(array=w358, index #1=w383, index #2=w381, index #3=w380, index #4=w379, index #5=w378, index #6=w374, index #7=w373, index #8=w377, index #9=w376, index #10=w375) -> (element #1=w382:u16, element #2=w371:u16, element #3=w370:u16, element #4=w369:u16, element #5=w368:u16, element #6=w366:u16, element #7=w365:u16, element #8=w364:u16, element #9=w363:u16, element #10=w362:u16)
              n213 = Not Equal To 0?(x=w371) -> (x != 0?=w372:bool)
              n214 = Not Equal To 0?(x=w365) -> (x != 0?=w367:bool)
              n215 = local write "LC_Reward_Probability"(w370) -> ()
              n216 = local write "LC_Wrong_Probability"(w364) -> ()
              n217 = local write "LC_Reward_Tdelay"(w369) -> ()
              n218 = local write "LC_Reward_OnOff"(w372) -> ()
              n219 = local write "LC_Reward_Block"(w382) -> ()
              n220 = local write "LC_Reward_Trial"(w368) -> ()
              n221 = local write "LC_Wrong_Tdelay"(w363) -> ()
              n222 = local write "LC_Wrong_OnOff"(w367) -> ()
              n223 = local write "LC_Wrong_Block"(w366) -> ()
              n224 = local write "LC_Wrong_Trial"(w362) -> ()
            }
            frame "UploadSettings_dataMTrig_1" {
              # "Tdelay_R"
              # "Tdelay_L"
              # "Tcycle_R"
              # "Tcycle_L"
              # "RewCalib_nCycle_R"
              # "RewCalib_nCycle_L"
              # "Solenoid"
              # "Laser_Tcycle"
              n225 = call "myRIO_BRig_RT_dataMTrig_Laser_Tcycle.vi"() -> ("output_Laser_Tcycle"=w394:i32)  [unwired: 11 in]
              n226 = call "myRIO_BRig_RT_dataMTrig_Solenoid_RewCalib_nCycle__L.vi"() -> ("output_Solenoid_RewCalib_nCycle__L"=w393:i32)  [unwired: 11 in]
              n227 = call "myRIO_BRig_RT_dataMTrig_Solenoid_RewCalib_nCycle__R.vi"() -> ("output_Solenoid_RewCalib_nCycle__R"=w392:i32)  [unwired: 11 in]
              n228 = call "myRIO_BRig_RT_dataMTrig_Solenoid_Tdelay__L.vi"() -> ("output_Solenoid_Tdelay__L"=w389:i32)  [unwired: 11 in]
              n229 = call "myRIO_BRig_RT_dataMTrig_Solenoid_Tdelay__R.vi"() -> ("output_Solenoid_Tdelay__R"=w388:i32)  [unwired: 11 in]
              n230 = call "myRIO_BRig_RT_dataMTrig_Solenoid_Tcycle__L.vi"() -> ("output_Solenoid_Tcycle__L"=w391:i32)  [unwired: 11 in]
              n231 = call "myRIO_BRig_RT_dataMTrig_Solenoid_Tcycle__R.vi"() -> ("output_Solenoid_Tcycle__R"=w390:i32)  [unwired: 11 in]
              n232 = Index Array(array=w387, index #1=w394, index #2=w393, index #3=w392, index #4=w391, index #5=w390, index #6=w389, index #7=w388) -> (element #1=w401:u16, element #2=w400:u16, element #3=w399:u16, element #4=w398:u16, element #5=w397:u16, element #6=w396:u16, element #7=w395:u16)
              n233 = Replace Array Subset(array=w406, new element #1=w401, index #1=w394, new element #2=w400, index #2=w393, new element #3=w399, index #3=w392, new element #4=w398, index #4=w391, new element #5=w397, index #5=w390, new element #6=w396, index #6=w389, new element #7=w395, index #7=w388) -> (w405:u16[])
              n234 = local write "MTrig_Solenoid_Tcycle__L"(w398) -> ()
              n235 = local write "MTrig_Solenoid_Tcycle__R"(w397) -> ()
              n236 = local write "MTrig_Laser_Tcycle"(w401) -> ()
            }
            frame "Idle" {
              # "To ensure timing, we split the\nidle state into 4 phases"
              # "Laser_Tcycle"
              # "Audio_Tcycle_R"
              # "Audio_Tcycle_L"
              n237 = local read "MTrig_Audio_trig__L"() -> (w417:bool)
              n238 = local read "MTrig_Audio_trig__R"() -> (w419:bool)
              n239 = Select(t=myRIO_BRig_RT__Case_NonExp_stateList."SendData" ("Enum"), s="SendData", f=myRIO_BRig_RT__Case_NonExp_stateList."Idle_2" ("Enum")) -> (s? t:f=w412:T1)
              n240 = local read "MTrig_Laser_trig"() -> (w418:bool)
              n241 = call "myRIO_BRig_RT_dataMTrig_Audio_Tcycle__L.vi"() -> ("output_Audio_Tcycle__L"=w430:i32)  [unwired: 11 in]
              n242 = call "myRIO_BRig_RT_dataMTrig_Audio_Tcycle__R.vi"() -> ("output_Audio_Tcycle__R"=w429:i32)  [unwired: 11 in]
              n243 = call "myRIO_BRig_RT_dataMTrig_Laser_Tcycle.vi"() -> ("output_Laser_Tcycle"=w428:i32)  [unwired: 11 in]
              n244 = local read "MTrig_Laser_Tcycle"() -> (w410:u16)
              n245 = Select(t=myRIO_BRig_RT__Case_NonExp_stateList."TestConnection" ("Enum"), s="TestConnection", f=w412) -> (s? t:f=w421:T1)
              n246 = local read "Tcycle_Cue_min"() -> (w411:u16)
              n247 = Compound Arithmetic op=OR(w417, w419, w418) -> (w420:bool)
              n248 = case shown="True" w420 {
                frame False {
                }
                frame True {
                  w431 = FALSE
                  n249 = local write "MTrig_Audio_trig__L"(w431) -> ()
                  n250 = local write "MTrig_Audio_trig__R"(w431) -> ()
                  n251 = local write "MTrig_Laser_trig"(w431) -> ()
                }
              }
              n252 = Replace Array Subset(array=w426, new element #1=w411, index #1=w430, new element #2=w411, index #2=w429, new element #3=w410, index #3=w428) -> (w427:u16[])
              n253 = local read "Audio_Amp__R"() -> (w422:u16)
              n254 = local read "Audio_Amp__L"() -> (w423:u16)
              n255 = local read "Audio_Freq__R"() -> (w408:u8)
              n256 = local read "Audio_Freq__L"() -> (w409:u8)
            }
            frame "Idle_2" {
              # "To ensure timing, we split the\nidle state into 4 phases"
              # "Ncycles"
              # "Ncycles"
              # "RewCalib"
              # "RewCalib"
              # "Solenoid R"
              # "Solenoid L"
              n257 = call "myRIO_BRig_RT_dataMTrig_Solenoid_RewCalib_OnOff__L.vi"() -> ("output_Solenoid_RewCalib_OnOff__L"=w461:i32)  [unwired: 11 in]
              n258 = call "myRIO_BRig_RT_dataMTrig_Solenoid_N__L.vi"() -> ("output_Solenoid_N__L"=w449:i32)  [unwired: 11 in]
              n259 = call "myRIO_BRig_RT_dataMTrig_Solenoid_RewCalib_OnOff__R.vi"() -> ("output_Solenoid_RewCalib_OnOff__R"=w446:i32)  [unwired: 11 in]
              n260 = call "myRIO_BRig_RT_dataMTrig_Solenoid_N__R.vi"() -> ("output_Solenoid_N__R"=w445:i32)  [unwired: 11 in]
              n261 = Index Array(array=w452, index #1=w461, index #2=w449, index #3=w446, index #4=w445) -> (element #1=w448:u16, element #2=w443:u16, element #3=w444:u16, element #4=w442:u16)
              n262 = local read "RewCalib_Trig_L"() -> (w441:bool)
              n263 = local read "RewCalib_Trig_R"() -> (w440:bool)
              n264 = Equal To 0?(x=w443) -> (x = 0?=w451:bool)
              n265 = Equal To 0?(x=w442) -> (x = 0?=w450:bool)
              n266 = Not Equal To 0?(x=w444) -> (x != 0?=w462:bool)
              n267 = Not Equal To 0?(x=w448) -> (x != 0?=w463:bool)
              n268 = And(x=w451, y=w450) -> (x .and. y?=w455:bool)
              n269 = Or(x=w441, y=w440) -> (x .or. y?=w456:bool)
              n270 = Not Exclusive Or(1:w463, 2:w441) -> (0:w458:bool)
              n271 = Not Exclusive Or(1:w462, 2:w440) -> (0:w460:bool)
              n272 = And(x=w456, y=w455) -> (x .and. y?=w438:bool)
              n273 = Not(x=w458) -> (.not. x?=w457:bool)
              n274 = Not(x=w460) -> (.not. x?=w459:bool)
              n275 = Or(x=w457, y=w459) -> (x .or. y?=w439:bool)
              n276 = Or(x=w438, y=w439) -> (x .or. y?=w454:bool)
              n277 = Select(t=myRIO_BRig_RT__Case_NonExp_stateList."RewardCalibration_pre" ("Enum"), s=w454, f=myRIO_BRig_RT__Case_NonExp_stateList."Idle_3" ("Enum")) -> (s? t:f=w437:T1)
            }
            frame "Idle_3" {
              w487 = u8 0 ("f")
              # "To ensure timing, we split the\nidle state into 4 phases"
              n278 = local read "MTrig_Solenoid_trig__L"() -> (w475:bool)
              n279 = local read "MTrig_Solenoid_trig__R"() -> (w488:bool)
              n280 = local read "warmupType"() -> (w465:u8)
              n281 = local read "warmup"() -> (w480:bool)
              n282 = Not Equal To 0?(x=w465) -> (x != 0?=w464:bool)
              n283 = Not(x=w464) -> (.not. x?=w481:bool)
              n284 = Select(t=u8 1, s=w475, f=w487) -> (s? t:f=w486:u8)
              n285 = Select(t=u8 2, s=w488, f=w487) -> (s? t:f=w485:u8)
              n286 = And(x=w480, y=w481) -> (x .and. y?=w479:bool)
              n287 = And(x=w480, y=w464) -> (x .and. y?=w470:bool)
              n288 = Add(x=w486, y=w485) -> (x+y=w484:u8)
              n289 = case shown="3" w484 {
                tunnel: w483 -> [w491 w495 w513 w531]
                tunnel: [w491 w494 w512 w530] -> w482
                tunnel: w479 -> [_ w493 w511 w529]
                tunnel: [_ TRUE TRUE TRUE] -> w472
                frame 0, Default {
                }
                frame 1 {
                  n290 = case shown="True" w493 {
                    tunnel: w495 -> [w504 w509]
                    tunnel: [w503 w508] -> w494
                    frame True {
                      # "Audio_L"
                      # "Solenoid_L"
                      n291 = call "myRIO_BRig_RT_dataMTrig_Solenoid_N__L.vi"() -> ("output_Solenoid_N__L"=w500:i32)  [unwired: 11 in]
                      n292 = call "myRIO_BRig_RT_dataMTrig_Audio_N__L.vi"() -> ("output_Audio_N__L"=w498:i32)  [unwired: 11 in]
                      n293 = Index Array(array=w504, index #1=w500, index #2=w498) -> (element #1=w502:u16, element #2=w501:u16)
                      n294 = Increment(x=w502) -> (x+1=w499:u16)
                      n295 = Increment(x=w501) -> (x+1=w497:u16)
                      n296 = Replace Array Subset(array=w504, new element #1=w499, index #1=w500, new element #2=w497, index #2=w498) -> (w503:u16[])
                    }
                    frame False {
                      # "Solenoid_L"
                      n297 = call "myRIO_BRig_RT_dataMTrig_Solenoid_N__L.vi"() -> ("output_Solenoid_N__L"=w506:i32)  [unwired: 11 in]
                      n298 = Index Array(array=w509, index=w506) -> (element=w507:u16)
                      n299 = Increment(x=w507) -> (x+1=w505:u16)
                      n300 = Replace Array Subset(array=w509, new element=w505, index=w506) -> (w508:u16[])
                    }
                  }
                  n301 = local write "MTrig_Solenoid_trig__L"(FALSE) -> ()
                }
                frame 2 {
                  n302 = case shown="True" w511 {
                    tunnel: w513 -> [w522 w527]
                    tunnel: [w521 w526] -> w512
                    frame True {
                      # "Audio_R"
                      # "Solenoid_R"
                      n303 = call "myRIO_BRig_RT_dataMTrig_Solenoid_N__R.vi"() -> ("output_Solenoid_N__R"=w518:i32)  [unwired: 11 in]
                      n304 = call "myRIO_BRig_RT_dataMTrig_Audio_N__R.vi"() -> ("output_Audio_N__R"=w517:i32)  [unwired: 11 in]
                      n305 = Index Array(array=w522, index #1=w518, index #2=w517) -> (element #1=w520:u16, element #2=w519:u16)
                      n306 = Increment(x=w519) -> (x+1=w515:u16)
                      n307 = Increment(x=w520) -> (x+1=w516:u16)
                      n308 = Replace Array Subset(array=w522, new element #1=w516, index #1=w518, new element #2=w515, index #2=w517) -> (w521:u16[])
                    }
                    frame False {
                      # "Solenoid_R"
                      n309 = call "myRIO_BRig_RT_dataMTrig_Solenoid_N__R.vi"() -> ("output_Solenoid_N__R"=w523:i32)  [unwired: 11 in]
                      n310 = Index Array(array=w527, index=w523) -> (element=w525:u16)
                      n311 = Increment(x=w525) -> (x+1=w524:u16)
                      n312 = Replace Array Subset(array=w527, new element=w524, index=w523) -> (w526:u16[])
                    }
                  }
                  n313 = local write "MTrig_Solenoid_trig__R"(FALSE) -> ()
                }
                frame 3 {
                  w532 = FALSE
                  n314 = case shown="True" w529 {
                    tunnel: w531 -> [w546 w554]
                    tunnel: [w545 w553] -> w530
                    frame True {
                      # "Audio_R"
                      # "Solenoid_R"
                      # "Audio_L"
                      # "Solenoid_L"
                      n315 = call "myRIO_BRig_RT_dataMTrig_Solenoid_N__L.vi"() -> ("output_Solenoid_N__L"=w540:i32)  [unwired: 11 in]
                      n316 = call "myRIO_BRig_RT_dataMTrig_Audio_N__L.vi"() -> ("output_Audio_N__L"=w538:i32)  [unwired: 11 in]
                      n317 = call "myRIO_BRig_RT_dataMTrig_Solenoid_N__R.vi"() -> ("output_Solenoid_N__R"=w536:i32)  [unwired: 11 in]
                      n318 = call "myRIO_BRig_RT_dataMTrig_Audio_N__R.vi"() -> ("output_Audio_N__R"=w535:i32)  [unwired: 11 in]
                      n319 = Index Array(array=w546, index #1=w540, index #2=w538, index #3=w536, index #4=w535) -> (element #1=w544:u16, element #2=w543:u16, element #3=w542:u16, element #4=w541:u16)
                      n320 = Increment(x=w541) -> (x+1=w533:u16)
                      n321 = Increment(x=w544) -> (x+1=w539:u16)
                      n322 = Increment(x=w543) -> (x+1=w537:u16)
                      n323 = Increment(x=w542) -> (x+1=w534:u16)
                      n324 = Replace Array Subset(array=w546, new element #1=w539, index #1=w540, new element #2=w537, index #2=w538, new element #3=w534, index #3=w536, new element #4=w533, index #4=w535) -> (w545:u16[])
                    }
                    frame False {
                      # "Solenoid_R"
                      # "Solenoid_L"
                      n325 = call "myRIO_BRig_RT_dataMTrig_Solenoid_N__L.vi"() -> ("output_Solenoid_N__L"=w550:i32)  [unwired: 11 in]
                      n326 = call "myRIO_BRig_RT_dataMTrig_Solenoid_N__R.vi"() -> ("output_Solenoid_N__R"=w547:i32)  [unwired: 11 in]
                      n327 = Index Array(array=w554, index #1=w550, index #2=w547) -> (element #1=w552:u16, element #2=w551:u16)
                      n328 = Increment(x=w552) -> (x+1=w549:u16)
                      n329 = Increment(x=w551) -> (x+1=w548:u16)
                      n330 = Replace Array Subset(array=w554, new element #1=w549, index #1=w550, new element #2=w548, index #2=w547) -> (w553:u16[])
                    }
                  }
                  n331 = local write "MTrig_Solenoid_trig__L"(w532) -> ()
                  n332 = local write "MTrig_Solenoid_trig__R"(w532) -> ()
                }
              }
              n333 = Select(t=myRIO_BRig_RT__Case_NonExp_stateList."Cue_pre", s=w470, f=myRIO_BRig_RT__Case_NonExp_stateList."DispenseWater_pre" ("Enum")) -> (s? t:f=w468:T1)
              n334 = Select(t=w468, s=w472, f=myRIO_BRig_RT__Case_NonExp_stateList."Idle_4" ("Enum")) -> (s? t:f=w473:T1)
            }
            frame "Idle_4" {
              # "use dataMTrig as it is one of the last to transfer"
              # "To ensure timing, we split the\nidle state into 4 phases"
              n335 = call "myRIO_BRig_RT_comm_webdav_uploadReceived_check_v2,0.vi"("input_dataName"="dataMTrig") -> ("output_Iexist"=w564:bool)  [unwired: 9 in, 1 out]
              n336 = Select(t=myRIO_BRig_RT__Case_NonExp_stateList."UploadSettings_pre" ("Enum"), s=w564, f=myRIO_BRig_RT__Case_NonExp_stateList."Idle") -> (s? t:f=w562:T1)
            }
            frame "Cue_pre" {
              w573 = u16 1 ("t")
              w572 = u16 0 ("new element/subarray")
              w569 = u16 0 ("new element/subarray")
              # "Ncycle"
              # "count"
              # "Audio_R"
              # "Solenoid_R"
              # "Solenoid_L"
              # "Ncycle"
              # "count"
              # "Audio_L"
              n337 = call "myRIO_BRig_RT_dataMTrig_Solenoid_N__L.vi"() -> ("output_Solenoid_N__L"=w584:i32)  [unwired: 11 in]
              n338 = call "myRIO_BRig_RT_dataMTrig_Solenoid_N__R.vi"() -> ("output_Solenoid_N__R"=w583:i32)  [unwired: 11 in]
              n339 = Index Array(array=w580, index #1=w584, index #2=w583) -> (element #1=w582:u16, element #2=w581:u16)
              n340 = Not Equal To 0?(x=w581) -> (x != 0?=w574:bool)
              n341 = Not Equal To 0?(x=w582) -> (x != 0?=w576:bool)
              n342 = Select(t=w573, s=w576, f=w572) -> (s? t:f=w575:u16)
              n343 = Select(t=w573, s=w574, f=w572) -> (s? t:f=w568:u16)
              n344 = call "myRIO_BRig_RT_dataMTrig_Audio_c__L.vi"() -> ("output_Audio_c__L"=w578:i32)  [unwired: 11 in]
              n345 = call "myRIO_BRig_RT_dataMTrig_Audio_N__L.vi"() -> ("output_Audio_N__L"=w577:i32)  [unwired: 11 in]
              n346 = call "myRIO_BRig_RT_dataMTrig_Audio_c__R.vi"() -> ("output_Audio_c__R"=w571:i32)  [unwired: 11 in]
              n347 = call "myRIO_BRig_RT_dataMTrig_Audio_N__R.vi"() -> ("output_Audio_N__R"=w570:i32)  [unwired: 11 in]
              n348 = Replace Array Subset(array=w580, new element #1=w569, index #1=w578, new element #2=w575, index #2=w577, new element #3=w569, index #3=w571, new element #4=w568, index #4=w570) -> (w579:u16[])
            }
            frame "Cue" {
              # "lick did not occur or warmupType==1"
              # "lick occurred?"
              # "Ncycle"
              # "Audio_R"
              # "Ncycle"
              # "Audio_L"
              n349 = local read "warmupType"() -> (w595:u8)
              n350 = Greater?(x=w601, y=w600) -> (0:w604:bool)
              n351 = Greater?(x=w603, y=w602) -> (0:w599:bool)
              n352 = Or(x=w599, y=w604) -> (x .or. y?=w593:bool)
              n353 = Equal?(x=w595, y=u8 1) -> (x = y?=w592:bool)
              n354 = Not(x=w593) -> (.not. x?=w591:bool)
              n355 = call "myRIO_BRig_RT_dataMTrig_Audio_N__L.vi"() -> ("output_Audio_N__L"=w608:i32)  [unwired: 11 in]
              n356 = call "myRIO_BRig_RT_dataMTrig_Audio_N__R.vi"() -> ("output_Audio_N__R"=w607:i32)  [unwired: 11 in]
              n357 = Or(x=w591, y=w592) -> (x .or. y?=w590:bool)
              n358 = case shown="False" w590 {
                tunnel: w608 -> [w615 w628]
                tunnel: w607 -> [w614 w627]
                tunnel: w598 -> [w617 w622]
                tunnel: [w616 w622] -> w597
                tunnel: w596 -> [_ w619]
                tunnel: [myRIO_BRig_RT__Case_NonExp_stateList."Idle" ("t") w618] -> w589
                frame False {
                  w613 = u16 0 ("new element/subarray")
                  # "lick occurred and warmupType==2"
                  n359 = Replace Array Subset(array=w617, new element #1=w613, index #1=w615, new element #2=w613, index #2=w614) -> (w616:u16[])
                }
                frame True {
                  n360 = Index Array(array=w622, index #1=w628, index #2=w627) -> (element #1=w626:u16, element #2=w625:u16)
                  n361 = Equal To 0?(x=w626) -> (x = 0?=w624:bool)
                  n362 = Equal To 0?(x=w625) -> (x = 0?=w623:bool)
                  n363 = And(x=w624, y=w623) -> (x .and. y?=w620:bool)
                  n364 = Select(t=myRIO_BRig_RT__Case_NonExp_stateList."DispenseWater_pre", s=w620, f=w619) -> (s? t:f=w618:T1)
                }
              }
            }
            frame "RewardCalibration_pre" {
              (unwired) FALSE
              w634 = FALSE
              w645 = u8 0
              w661 = u8 0
              # "Are we starting a RewardCalibration?\nOr are we stopping a RewardCalibration?\nOr is a RewardCalibration over?"
              # "RewCalib\nOnOff"
              # "N"
              # "Solenoid R"
              # "RewCalib\nOnOff"
              # "N"
              # "Solenoid L"
              n365 = local read "RewCalib_Trig_L"() -> (w668:bool)
              n366 = local read "RewCalib_Trig_R"() -> (w637:bool)
              n367 = call "myRIO_BRig_RT_dataMTrig_Solenoid_N__R.vi"() -> ("output_Solenoid_N__R"=w639:i32)  [unwired: 11 in]
              n368 = call "myRIO_BRig_RT_dataMTrig_Solenoid_RewCalib_OnOff__R.vi"() -> ("output_Solenoid_RewCalib_OnOff__R"=w636:i32)  [unwired: 11 in]
              n369 = call "myRIO_BRig_RT_dataMTrig_Solenoid_N__L.vi"() -> ("output_Solenoid_N__L"=w654:i32)  [unwired: 11 in]
              n370 = call "myRIO_BRig_RT_dataMTrig_Solenoid_RewCalib_OnOff__L.vi"() -> ("output_Solenoid_RewCalib_OnOff__L"=w655:i32)  [unwired: 11 in]
              n371 = Index Array(array=w638, index #1=w639, index #2=w636) -> (element #1=w649:u16, element #2=w644:u16)
              n372 = Index Array(array=w638, index #1=w654, index #2=w655) -> (element #1=w665:u16, element #2=w660:u16)
              n373 = Equal To 0?(x=w649) -> (x = 0?=w650:bool)
              n374 = Not Equal To 0?(x=w644) -> (x != 0?=w647:bool)
              n375 = Equal To 0?(x=w665) -> (x = 0?=w666:bool)
              n376 = Not Equal To 0?(x=w660) -> (x != 0?=w663:bool)
              n377 = local write "MTrig_Solenoid_trig__L"(w634) -> ()
              n378 = local write "MTrig_Solenoid_trig__R"(w634) -> ()
              n379 = Select(t=u8 1, s=w637, f=w645) -> (s? t:f=w641:u8)
              n380 = Select(t=u8 1, s=w668, f=w661) -> (s? t:f=w657:u8)
              n381 = Select(t=u8 2, s=w650, f=w645) -> (s? t:f=w642:u8)
              n382 = Select(t=u8 4, s=w647, f=w645) -> (s? t:f=w643:u8)
              n383 = Select(t=u8 2, s=w666, f=w661) -> (s? t:f=w658:u8)
              n384 = Select(t=u8 4, s=w663, f=w661) -> (s? t:f=w659:u8)
              n385 = Compound Arithmetic op=ADD(w641, w642, w643) -> (w640:u8)
              n386 = Compound Arithmetic op=ADD(w657, w658, w659) -> (w656:u8)
              n387 = case shown="7" w656 {
                tunnel: w638 -> [w698 w703 w705 w710 w715 w717 w720 w725]
                tunnel: [w698 w704 w705 w711 w716 w717 w721 w726] -> w653
                tunnel: w655 -> [_ w701 _ w708 w713 _ w719 w724]
                tunnel: w654 -> [_ w702 _ w709 w714 _ _ _]
                frame 0, Default {
                }
                frame 1 {
                  n388 = Replace Array Subset(array=w703, new element #1=u16 100 ("new element/subarray"), index #1=w702, new element #2=u16 1 ("new element/subarray"), index #2=w701) -> (w704:u16[])
                }
                frame 2 {
                }
                frame 3 {
                  n389 = Replace Array Subset(array=w710, new element #1=u16 100 ("new element/subarray"), index #1=w709, new element #2=u16 1 ("new element/subarray"), index #2=w708) -> (w711:u16[])
                }
                frame 4 {
                  w712 = u16 0 ("new element/subarray")
                  n390 = Replace Array Subset(array=w715, new element #1=w712, index #1=w714, new element #2=w712, index #2=w713) -> (w716:u16[])
                }
                frame 5 {
                }
                frame 6 {
                  n391 = Replace Array Subset(array=w720, new element=u16 0 ("new element/subarray"), index=w719) -> (w721:u16[])
                }
                frame 7 {
                  n392 = local write "RewCalib_Trig_L"(FALSE ("RewCalib_Trig_L")) -> ()
                  n393 = Replace Array Subset(array=w725, new element=u16 0 ("new element/subarray"), index=w724) -> (w726:u16[])
                }
              }
              n394 = case shown="7" w640 {
                tunnel: w653 -> [w669 w674 w676 w681 w686 w688 w691 w696]
                tunnel: [w669 w675 w676 w682 w687 w688 w692 w697] -> w652
                tunnel: w636 -> [_ w672 _ w679 w684 _ w690 w695]
                tunnel: w639 -> [_ w673 _ w680 w685 _ _ _]
                frame 0, Default {
                }
                frame 1 {
                  n395 = Replace Array Subset(array=w674, new element #1=u16 100 ("new element/subarray"), index #1=w673, new element #2=u16 1 ("new element/subarray"), index #2=w672) -> (w675:u16[])
                }
                frame 2 {
                }
                frame 3 {
                  n396 = Replace Array Subset(array=w681, new element #1=u16 100 ("new element/subarray"), index #1=w680, new element #2=u16 1 ("new element/subarray"), index #2=w679) -> (w682:u16[])
                }
                frame 4 {
                  w683 = u16 0 ("new element/subarray")
                  n397 = Replace Array Subset(array=w686, new element #1=w683, index #1=w685, new element #2=w683, index #2=w684) -> (w687:u16[])
                }
                frame 5 {
                }
                frame 6 {
                  n398 = Replace Array Subset(array=w691, new element=u16 0 ("new element/subarray"), index=w690) -> (w692:u16[])
                }
                frame 7 {
                  n399 = local write "RewCalib_Trig_R"(FALSE ("RewCalib_Trig_L")) -> ()
                  n400 = Replace Array Subset(array=w696, new element=u16 0 ("new element/subarray"), index=w695) -> (w697:u16[])
                }
              }
            }
            frame "DispenseWater_pre" {
              w734 = u16 0 ("t")
              w777 = u16 0 ("new element/subarray")
              # "just trust me on this one"
              # "RewCalib\nOnOff"
              # "RewCalib\nOnOff"
              # "nCycle"
              # "Solenoid__R"
              # "Tdelay"
              # "delay"
              # "nCycle"
              # "Solenoid__L"
              # "Tdelay"
              # "delay"
              # "Solenoid__R"
              # "count"
              # "Solenoid_Tcycle_R"
              # "Solenoid_Tcycle_L"
              # "Solenoid__L"
              # "count"
              n401 = call "myRIO_BRig_RT_dataMTrig_Solenoid_RewCalib_OnOff__L.vi"() -> ("output_Solenoid_RewCalib_OnOff__L"=w741:i32)  [unwired: 11 in]
              n402 = call "myRIO_BRig_RT_dataMTrig_Solenoid_N__L.vi"() -> ("output_Solenoid_N__L"=w732:i32)  [unwired: 11 in]
              n403 = call "myRIO_BRig_RT_dataMTrig_Solenoid_delay__L.vi"() -> ("output_Solenoid_delay__L"=w775:i32)  [unwired: 11 in]
              n404 = call "myRIO_BRig_RT_dataMTrig_Solenoid_Tdelay__L.vi"() -> ("output_Solenoid_Tdelay__L"=w774:i32)  [unwired: 11 in]
              n405 = call "myRIO_BRig_RT_dataMTrig_Solenoid_N__R.vi"() -> ("output_Solenoid_N__R"=w730:i32)  [unwired: 11 in]
              n406 = call "myRIO_BRig_RT_dataMTrig_Solenoid_delay__R.vi"() -> ("output_Solenoid_delay__R"=w764:i32)  [unwired: 11 in]
              n407 = call "myRIO_BRig_RT_dataMTrig_Solenoid_Tdelay__R.vi"() -> ("output_Solenoid_Tdelay__R"=w763:i32)  [unwired: 11 in]
              n408 = call "myRIO_BRig_RT_dataMTrig_Solenoid_RewCalib_OnOff__R.vi"() -> ("output_Solenoid_RewCalib_OnOff__R"=w737:i32)  [unwired: 11 in]
              n409 = Index Array(array=w776, index #1=w732, index #2=w775, index #3=w774, index #4=w730, index #5=w764, index #6=w763, index #7=w741, index #8=w737) -> (element #1=w733:u16, element #2=w773:u16, element #3=w768:u16, element #4=w736:u16, element #5=w758:u16, element #6=w757:u16, element #7=w742:u16, element #8=w739:u16)
              n410 = Equal To 0?(x=w773) -> (x = 0?=w772:bool)
              n411 = Equal To 0?(x=w758) -> (x = 0?=w762:bool)
              n412 = local read "RewCalib_Trig_L"() -> (w753:bool)
              n413 = local read "RewCalib_Trig_R"() -> (w748:bool)
              n414 = Not Equal To 0?(x=w733) -> (x != 0?=w771:bool)
              n415 = Not Equal To 0?(x=w736) -> (x != 0?=w761:bool)
              n416 = local read "MTrig_Solenoid_Tcycle__L"() -> (w770:u16)
              n417 = local read "MTrig_Solenoid_Tcycle__R"() -> (w756:u16)
              n418 = Not Equal To 0?(x=w742) -> (x != 0?=w752:bool)
              n419 = Not Equal To 0?(x=w739) -> (x != 0?=w750:bool)
              n420 = Not(x=w753) -> (.not. x?=w751:bool)
              n421 = Not(x=w748) -> (.not. x?=w749:bool)
              n422 = And(x=w752, y=w751) -> (x .and. y?=w747:bool)
              n423 = And(x=w750, y=w749) -> (x .and. y?=w746:bool)
              n424 = call "myRIO_BRig_RT_dataMTrig_Solenoid_c__L.vi"() -> ("output_Solenoid_c__L"=w779:i32)  [unwired: 11 in]
              n425 = call "myRIO_BRig_RT_dataMTrig_Solenoid_c__R.vi"() -> ("output_Solenoid_c__R"=w778:i32)  [unwired: 11 in]
              n426 = Select(t=w770, s=w771, f=u16 0) -> (s? t:f=w767:u16)
              n427 = Or(x=w747, y=w746) -> (x .or. y?=w735:bool)
              n428 = Select(t=w756, s=w761, f=u16 0) -> (s? t:f=w759:u16)
              n429 = Select(t=w767, s=w772, f=w768) -> (s? t:f=w765:u16)
              n430 = Select(t=w759, s=w762, f=w757) -> (s? t:f=w754:u16)
              n431 = call "myRIO_BRig_RT_dataMTrig_Solenoid_Tcycle__L.vi"() -> ("output_Solenoid_Tcycle__L"=w766:i32)  [unwired: 11 in]
              n432 = call "myRIO_BRig_RT_dataMTrig_Solenoid_Tcycle__R.vi"() -> ("output_Solenoid_Tcycle__R"=w755:i32)  [unwired: 11 in]
              n433 = Select(t=w734, s=w735, f=w733) -> (s? t:f=w731:u16)
              n434 = Select(t=w734, s=w735, f=w736) -> (s? t:f=w729:u16)
              n435 = Select(t=myRIO_BRig_RT__Case_NonExp_stateList."Idle" ("Enum"), s=w735, f=myRIO_BRig_RT__Case_NonExp_stateList."DispenseWater" ("Enum")) -> (s? t:f=w743:T1)
              n436 = Select(t=w734, s=w735, f=w742) -> (s? t:f=w740:u16)
              n437 = Select(t=w734, s=w735, f=w739) -> (s? t:f=w738:u16)
              n438 = Replace Array Subset(array=w776, new element #1=w777, index #1=w779, new element #2=w777, index #2=w778, new element #3=w765, index #3=w766, new element #4=w754, index #4=w755, new element #5=w740, index #5=w741, new element #6=w738, index #6=w737, new element #7=w731, index #7=w732, new element #8=w729, index #8=w730) -> (w780:u16[])
            }
            frame "DispenseWater" {
              # "D"
              # "C"
              # "B"
              # "A"
              # "(A) Add COUNT and INCREMENT\n(B) Is (A) smaller than Tcycle?\n(C) Are we dispensing water or in the delay phase?\n(D) If (A) is smaller than Tcycle   AND   if we are dispensing water\n      then send TRUE to solenoid"
              # "delay"
              # "Tcycle"
              # "Solenoid__R"
              # "count"
              # "delay"
              # "Tcycle"
              # "Solenoid__L"
              # "count"
              n439 = To Unsigned Word Integer(number=w812) -> (unsigned 16bit integer=w794:u16)
              n440 = call "myRIO_BRig_RT_dataMTrig_Solenoid_delay__R.vi"() -> ("output_Solenoid_delay__R"=w798:i32)  [unwired: 11 in]
              n441 = call "myRIO_BRig_RT_dataMTrig_Solenoid_c__R.vi"() -> ("output_Solenoid_c__R"=w797:i32)  [unwired: 11 in]
              n442 = call "myRIO_BRig_RT_dataMTrig_Solenoid_Tcycle__R.vi"() -> ("output_Solenoid_Tcycle__R"=w799:i32)  [unwired: 11 in]
              n443 = call "myRIO_BRig_RT_dataMTrig_Solenoid_delay__L.vi"() -> ("output_Solenoid_delay__L"=w814:i32)  [unwired: 11 in]
              n444 = call "myRIO_BRig_RT_dataMTrig_Solenoid_c__L.vi"() -> ("output_Solenoid_c__L"=w806:i32)  [unwired: 11 in]
              n445 = call "myRIO_BRig_RT_dataMTrig_Solenoid_Tcycle__L.vi"() -> ("output_Solenoid_Tcycle__L"=w815:i32)  [unwired: 11 in]
              n446 = Index Array(array=w808, index #1=w806, index #2=w815, index #3=w814, index #4=w797, index #5=w799, index #6=w798) -> (element #1=w813:u16, element #2=w803:u16, element #3=w811:u16, element #4=w793:u16, element #5=w790:u16, element #6=w789:u16)
              n447 = Add(x=w813, y=w794) -> (x+y=w804:u16)
              n448 = Add(x=w793, y=w794) -> (x+y=w795:u16)
              n449 = Less?(x=w804, y=w803) -> (x < y?=w787:bool)
              n450 = Equal To 0?(x=w811) -> (x = 0?=w810:bool)
              n451 = Less?(x=w795, y=w790) -> (x < y?=w788:bool)
              n452 = Equal To 0?(x=w789) -> (x = 0?=w796:bool)
              n453 = And(x=w787, y=w810) -> (x .and. y?=w809:bool)
              n454 = Or(x=w787, y=w788) -> (x .or. y?=w786:bool)
              n455 = And(x=w788, y=w796) -> (x .and. y?=w791:bool)
              n456 = Select(t=w804, s=w787, f=w803) -> (s? t:f=w805:u16)
              n457 = Select(t=w795, s=w788, f=w790) -> (s? t:f=w792:u16)
              n458 = Replace Array Subset(array=w808, new element #1=w805, index #1=w806, new element #2=w792, index #2=w797) -> (w807:u16[])
              n459 = Select(t=w802, s=w786, f=myRIO_BRig_RT__Case_NonExp_stateList."DispenseWater_post" ("Enum")) -> (s? t:f=w800:T1)
            }
            frame "DispenseWater_post" {
              # "nCycle"
              # "delay"
              # "Solenoid__R"
              # "nCycle"
              # "delay"
              # "Solenoid__L"
              n460 = call "myRIO_BRig_RT_dataMTrig_Solenoid_N__L.vi"() -> ("output_Solenoid_N__L"=w837:i32)  [unwired: 11 in]
              n461 = call "myRIO_BRig_RT_dataMTrig_Solenoid_delay__L.vi"() -> ("output_Solenoid_delay__L"=w836:i32)  [unwired: 11 in]
              n462 = call "myRIO_BRig_RT_dataMTrig_Solenoid_N__R.vi"() -> ("output_Solenoid_N__R"=w833:i32)  [unwired: 11 in]
              n463 = call "myRIO_BRig_RT_dataMTrig_Solenoid_delay__R.vi"() -> ("output_Solenoid_delay__R"=w832:i32)  [unwired: 11 in]
              n464 = Index Array(array=w839, index #1=w837, index #2=w836, index #3=w833, index #4=w832) -> (element #1=w841:u16, element #2=w840:u16, element #3=w824:u16, element #4=w826:u16)
              n465 = Not Equal To 0?(x=w841) -> (x != 0?=w842:bool)
              n466 = Not Equal To 0?(x=w824) -> (x != 0?=w825:bool)
              n467 = case shown="True" w825 {
                selector: w825 -> [_ w849]
                tunnel: w824 -> [w847 w855]
                tunnel: w826 -> [_ w856]
                tunnel: [w847 w853] -> w823
                tunnel: [u16 0 w852] -> w822
                tunnel: [_ w849] -> w821
                frame False {
                }
                frame True {
                  n468 = Equal To 0?(x=w856) -> (x = 0?=w848:bool)
                  n469 = Decrement(x=w855) -> (x-1=w854:u16)
                  n470 = Select(t=w854, s=w848, f=w855) -> (s? t:f=w853:u16)
                  n471 = Select(t=u16 1, s=w848, f=u16 0) -> (s? t:f=w852:u16)
                }
              }
              n472 = case shown="True" w842 {
                selector: w842 -> [_ w860]
                tunnel: w841 -> [w858 w866]
                tunnel: w840 -> [_ w867]
                tunnel: [w858 w864] -> w835
                tunnel: [u16 0 w863] -> w834
                tunnel: [_ w860] -> w831
                frame False {
                }
                frame True {
                  n473 = Equal To 0?(x=w867) -> (x = 0?=w859:bool)
                  n474 = Decrement(x=w866) -> (x-1=w865:u16)
                  n475 = Select(t=w865, s=w859, f=w866) -> (s? t:f=w864:u16)
                  n476 = Select(t=u16 1, s=w859, f=u16 0) -> (s? t:f=w863:u16)
                }
              }
              n477 = Or(x=w831, y=w821) -> (x .or. y?=w830:bool)
              n478 = Replace Array Subset(array=w839, new element #1=w835, index #1=w837, new element #2=w834, index #2=w836, new element #3=w823, index #3=w833, new element #4=w822, index #4=w832) -> (w838:u16[])
              n479 = Select(t=myRIO_BRig_RT__Case_NonExp_stateList."DispenseWater_pre" ("Enum"), s=w830, f=myRIO_BRig_RT__Case_NonExp_stateList."Idle" ("Enum")) -> (s? t:f=w827:T1)
            }
            frame "TestConnection" {
              n480 = local read "Host Password"() -> (w878:string)
              n481 = local read "Host UserName"() -> (w879:string)
              n482 = call "myRIO_BRig_RT_comm_webdav_testConnect.vi"("input_password"=w878, "input_username"=w879) -> ("output_Iconnected"=w876:bool)  [unwired: 9 in]
              n483 = Select(t="Connection accepted!" ("message"), s=w876, f="Error!") -> (s? t:f=w874:string)
              n484 = One Button Dialog(message=w874) -> ()  [unwired: 1 in, 1 out]
            }
            frame "SendData" {
              n485 = local read "Host Filename Prefix"() -> (w882:string)
              n486 = local read "Host Password"() -> (w883:string)
              n487 = local read "Host UserName"() -> (w884:string)
              n488 = call "myRIO_BRig_RT_comm_webdav_sendData_all.vi"("Host Filename Prefix"=w882, "Host Password"=w883, "Host UserName"=w884) -> ()  [unwired: 9 in]
            }
            frame "End" {
            }
          }
          n489 = local read "MTrig_Audio_trig__R"() -> (w86:bool)
          n490 = local read "MTrig_Audio_trig__L"() -> (w85:bool)
          n491 = local read "START"() -> (w81:bool)
          n492 = local read "STOP_abort"() -> (w80:bool)
          n493 = local read "MTrig_Laser_trig"() -> (w87:bool)
          n494 = call "myRIO_BRig_RT_dataMTrig_main__v2.vi"("input_dataMTrig"=w89, "input_Audio_trig_L"=w85, "input_Audio_trig_R"=w86, "input_Laser_trig"=w87) -> ("output_dataMTrig"=w88:u16[], "output_Audio_L"=w65:bool, "output_Audio_R"=w76:bool, "output_Laser"=w68:bool)  [unwired: 12 in]
          n495 = Or(x=w81, y=w80) -> (x .or. y?=w79:bool)
          n496 = Select(t=myRIO_BRig_RT__Case_NonExp_stateList."End" ("Enum"), s=w79, f=w78) -> (s? t:f=w77:T1)
          n497 = Or(x=w86, y=w87) -> (x .or. y?=w84:bool)
          n498 = Or(x=w84, y=w85) -> (x .or. y?=w83:bool)
          n499 = case shown="True" w83 {
            frame False {
            }
            frame True {
              w107 = FALSE
              n500 = local write "MTrig_Audio_trig__R"(w107) -> ()
              n501 = local write "MTrig_Audio_trig__L"(w107) -> ()
              n502 = local write "MTrig_Laser_trig"(w107) -> ()
            }
          }
          n503 = xnode "Read/Write Control"("FPGA VI Reference In"=w101, "error in"=w99, "A1_SR"=w90, "A3_SL"=w91, "audioTrigger_L"=w65, "audioAmp_L"=w58, "audioFreq_L_kHz"=w60, "audioTrigger_R"=w76, "audioAmp_R"=w59, "audioFreq_R_kHz"=w61, "laserResponse_reward_LED"="laserResponse_reward_LED", "laserResponse_wrong_LED"="laserResponse_wrong_LED", "laserResponse_reward"="laserResponse_reward", "laserResponse_wrong"="laserResponse_wrong", "SelectionState"="SelectionState", "ignoreWrong"="ignoreWrong", "Left(F)_or_Right(T)"="Left(F)_or_Right(T)", "laserMTrig"=w68) -> ("FPGA VI Reference Out"=w100:refnum<k20>, "error out"=w98:errorcluster, "SelectReward"=→"SelectReward":bool, "SelectWrong"=→"SelectWrong":bool)
          n504 = node-c288() -> ()  [unwired: 1 in, 1 out]
          "cState_NonExp" <- w97
        }
        n505 = node-c288(w49) -> ()  [unwired: 1 out]
        n506 = flat-sequence {
          tunnel: w42 -> [w53]
          tunnel: [w53] -> w41
          tunnel: w40 -> [w52]
          tunnel: [w52] -> w39
          frame #0 {
            w51 = FALSE
            n507 = local write "STOP_endBlock"(w51) -> ()
            n508 = local write "STOP_endTrial"(w51) -> ()
          }
        }
      }
      frame True {
        w904 = u8 0
        w906 = FALSE ("SelectionState")
        w911 = u16 0 ("idxDataBlock")
        w913 = u16 100 ("new element/subarray")
        w914 = u16 100 ("new element/subarray")
        w934 = T6 refnum items=["Session NI_WebDAV"] ("output_hSession")
        w943 = FALSE
        w944 = u16 0
        w905 = FALSE
        # "audio__L\naudio__R"
        # "Audio params"
        # "nRewards"
        # "idxDataBlock"
        # "Solenoid_Tdelay_R"
        # "Solenoid_Tdelay_L"
        # "RewCalib_N__R"
        # "RewCalib_N__L"
        # "Save dataLick to file\nSend file to Host\nSave dataMTrig\nSend file to Host\nDisconnect"
        # "dataTrial"
        # "dataTrial"
        # "Solenoid_Tcycle_R"
        # "Solenoid_Tcycle_L"
        # "Laser_Tcycle"
        # "Audio_Tcycle_R"
        # "Audio_Tcycle_L"
        # "dataLick"
        # "dataLC"
        # "dataLC"
        # "dataBlock"
        # "dataBlock"
        # "dataMTrig"
        # "dataMTrig"
        # "dataExp"
        # "dataCurrent"
        # "dataExp"
        # "dataCurrent"
        # "spout"
        # "state"
        n509 = call "myRIO_BRig_RT_dataMTrig_Solenoid_Tcycle__L.vi"() -> ("output_Solenoid_Tcycle__L"=w940:i32)  [unwired: 11 in]
        n510 = call "myRIO_BRig_RT_dataMTrig_Solenoid_Tcycle__R.vi"() -> ("output_Solenoid_Tcycle__R"=w939:i32)  [unwired: 11 in]
        n511 = call "myRIO_BRig_RT_dataMTrig_Audio_Tcycle__L.vi"() -> ("output_Audio_Tcycle__L"=w938:i32)  [unwired: 11 in]
        n512 = call "myRIO_BRig_RT_dataMTrig_Audio_Tcycle__R.vi"() -> ("output_Audio_Tcycle__R"=w937:i32)  [unwired: 11 in]
        n513 = call "myRIO_BRig_RT_dataMTrig_Laser_Tcycle.vi"() -> ("output_Laser_Tcycle"=w936:i32)  [unwired: 11 in]
        n514 = local read "MTrig_Solenoid_Tcycle__L"() -> (w919:u16)
        n515 = local read "MTrig_Solenoid_Tcycle__R"() -> (w918:u16)
        n516 = local read "Tcycle_Reward_L"() -> (w915:u16)
        n517 = local read "Tcycle_Reward_R"() -> (w916:u16)
        n518 = local read "MTrig_Laser_Tcycle"() -> (w917:u16)
        n519 = call "myRIO_BRig_RT_dataMTrig_Solenoid_RewCalib_nCycle__L.vi"() -> ("output_Solenoid_RewCalib_nCycle__L"=w922:i32)  [unwired: 11 in]
        n520 = call "myRIO_BRig_RT_dataMTrig_Solenoid_Tdelay__L.vi"() -> ("output_Solenoid_Tdelay__L"=w924:i32)  [unwired: 11 in]
        n521 = call "myRIO_BRig_RT_dataMTrig_Solenoid_RewCalib_nCycle__R.vi"() -> ("output_Solenoid_RewCalib_nCycle__R"=w923:i32)  [unwired: 11 in]
        n522 = call "myRIO_BRig_RT_dataMTrig_Solenoid_Tdelay__R.vi"() -> ("output_Solenoid_Tdelay__R"=w925:i32)  [unwired: 11 in]
        n523 = call "myRIO_BRig_RT_dataLick_init.vi"() -> ("output_dataLick"=w946:u16[][])  [unwired: 11 in]
        n524 = call "myRIO_BRig_RT_dataCurrent_init.vi"() -> ("output_dataCurrent"=w953:u16[])  [unwired: 11 in]
        n525 = call "myRIO_BRig_RT_dataExp_init.vi"() -> ("output_dataExp"=w952:u16[])  [unwired: 11 in]
        n526 = call "myRIO_BRig_RT_dataMTrig_init.vi"() -> ("output_dataMTrig"=w942:u16[])  [unwired: 5 in]
        n527 = call "myRIO_BRig_RT_dataLC_init.vi"() -> ("output_dataLC"=w950:u16[])  [unwired: 11 in]
        n528 = call "myRIO_BRig_RT_dataBlock_init.vi"() -> ("output_dataBlock"=w951:u16[][])  [unwired: 11 in]
        n529 = call "myRIO_BRig_RT_dataTrial_init.vi"() -> ("output_dataTrial"=w935:u16[][])  [unwired: 11 in]
        n530 = xnode "Read/Write Control"("FPGA VI Reference In"=w907, "error in"=w908, "SelectionState"=w906, "laserResponse_reward"=w906, "laserResponse_wrong"=w906, "laserResponse_reward_LED"=w906, "laserResponse_wrong_LED"=w906, "Left(F)_or_Right(T)"=w906, "ignoreWrong"=w906, "SelectionState"=w906) -> ("FPGA VI Reference Out"=w909:refnum<k20>, "error out"=w910:errorcluster)
        n531 = Replace Array Subset(array=w942, new element #1=w914, index #1=w922, new element #2=w914, index #2=w923, new element #3=w913, index #3=w924, new element #4=w913, index #4=w925, new element #5=w919, index #5=w940, new element #6=w918, index #6=w939, new element #7=w915, index #7=w938, new element #8=w916, index #8=w937, new element #9=w917, index #9=w936) -> (w941:u16[])
        n532 = Get Date/Time In Seconds() -> (seconds since 1Jan1904=w921:timestamp)
        n533 = To Double Precision Float(number=w921) -> (double precision float=w920:dbl)
        n534 = node-c288() -> (w961:T3)  [unwired: 4 in]
        n535 = timed-loop {
          timing: w961 -> [_]
          timing-out: [_] -> w960
          shift-right: [w1040] -> _
          shift-left: myRIO_BRig_RT__Case_Exp_stateList."Start1" ("Enum") -> [w1071]
          shift-right: [w1092] -> _
          shift-left: enum16{"Left", "Right"}."Left" -> [w1094]
          tunnel: w909 -> [w1091]
          tunnel: w910 -> [w1090]
          shift-right: [w1085] -> _
          shift-left: w958 -> [w1089]
          shift-right: [w1084] -> _
          shift-left: w957 -> [w1088]
          tunnel: [w1065] -> w955
          tunnel: [w1066] -> w956
          shift-right: [w1067] -> w926
          shift-left: w953 -> [w1032]
          shift-right: [w1083] -> _
          shift-left: w952 -> [w1027]
          shift-right: [w1054] -> w930
          shift-left: w941 -> [w1055]
          shift-right: [w1081] -> _
          shift-left: w951 -> [w1082]
          shift-right: [w1079] -> _
          shift-left: w950 -> [w1080]
          shift-right: [w1013] -> _
          shift-left: w905 -> [w1078]
          shift-right: [w1069] -> w932
          shift-left: w946 -> [w1070]
          shift-right: [w1056] -> _
          shift-left: w944 -> [w1064]
          shift-right: [w1024] -> _
          shift-left: w904 -> [w1063]
          shift-right: [w1057] -> _
          shift-left: w944 -> [w1062]
          shift-right: [w1058] -> _
          shift-left: w904 -> [w1061]
          shift-right: [w1025] -> _
          shift-left: w943 -> [w1059]
          shift-right: [w1026] -> _
          shift-left: w943 -> [w1060]
          shift-right: [w1038] -> _
          shift-left: w935 -> [w1039]
          shift-right: [w1037] -> w928
          shift-left: w934 -> [w1035]
          shift-right: [w1036] -> w929
          shift-left: FALSE ("output_Iconnected") -> [w1034]
          tunnel: "Host Filename Prefix" -> [w1033]
          tunnel: [w1033] -> w927
          shift-right: [w1008] -> _
          shift-left: w905 -> [w1031]
          tunnel: w920 -> [w1028]
          shift-right: [w1022] -> _
          shift-left: 0 ("idxDataBlock") -> [w1023]
          shift-right: [w1019] -> _
          shift-left: w911 -> [w1021]
          shift-right: [w1018] -> _
          shift-left: w911 -> [w1020]
          shift-right: [w1007] -> _
          shift-left: w905 -> [w1014]
          shift-right: [w1010] -> _
          shift-left: w905 -> [w1012]
          shift-right: [w1009] -> _
          shift-left: w905 -> [w1011]
          shift-right: [w1000] -> _
          shift-left: w905 -> [w1001]
          stop <- w1077 stop-if-true
          # "Laser"
          # "Audio R"
          # "Audio L"
          # "Solenoid R"
          # "Solenoid L"
          # "manual triggering"
          # "dataTrial"
          # "dataBlock"
          # "nRewards"
          # "laserOccurred"
          # "dataExp"
          # "dataCurrent"
          # "audio__L\naudio__R"
          # "time stamp"
          # "Audio params"
          # "nRewards"
          # "idxDataBlock"
          # "idxDataBlock"
          # "activate"
          # "audio__L\naudio__R"
          # "amp__R\nfreq__R"
          # "amp__L\nfreq__L"
          # "dataLC"
          # "solenoid__R"
          # "solenoid__L"
          # "Did a lick occur?"
          # "Update lick counter"
          # "spout"
          # "spout"
          # "state"
          # "state"
          n536 = node-c288() -> ()  [unwired: 1 in, 1 out]
          n537 = local read "MTrig_Solenoid_trig__L"() -> (w1052:bool)
          n538 = local read "MTrig_Solenoid_trig__R"() -> (w1051:bool)
          n539 = local read "MTrig_Audio_trig__L"() -> (w1050:bool)
          n540 = local read "MTrig_Audio_trig__R"() -> (w1049:bool)
          n541 = xnode "Read/Write Control"("FPGA VI Reference In"=w1091, "error in"=w1090) -> ("FPGA VI Reference Out"=w1017:refnum<k20>, "error out"=w1016:errorcluster, "A2_LickL"=w1085:u32, "A4_LickR"=w1084:u32)
          "A2" <- w1085
          "A4" <- w1084
          n542 = local read "MTrig_Laser_trig"() -> (w1048:bool)
          n543 = Greater?(x=w1085, y=w1089) -> (0:w1087:bool)
          n544 = Greater?(x=w1084, y=w1088) -> (0:w1086:bool)
          n545 = Or(x=w1087, y=w1086) -> (x .or. y?=w1093:bool)
          n546 = call "myRIO_BRig_RT_dataMTrig_main.vi"("input_dataMTrig"=w1055, "input_Solenoid_trig_L"=w1052, "input_Solenoid_trig_R"=w1051, "input_Audio_trig_L"=w1050, "input_Audio_trig_R"=w1049, "input_Laser_trig"=w1048) -> ("output_Laser"=w1005:bool, "output_dataMTrig"=w1054:u16[], "output_Solenoid_L"=w1042:bool, "output_Solenoid_R"=w1044:bool, "output_Audio_L"=w1046:bool, "output_Audio_R"=w1047:bool)  [unwired: 8 in]
          n547 = Compound Arithmetic op=OR(w1052, w1051, w1050, w1049, w1048) -> (w1053:bool)
          n548 = case shown="True" w1053 {
            frame False {
            }
            frame True {
              w1095 = FALSE
              n549 = local write "MTrig_Solenoid_trig__L"(w1095) -> ()
              n550 = local write "MTrig_Solenoid_trig__R"(w1095) -> ()
              n551 = local write "MTrig_Audio_trig__L"(w1095) -> ()
              n552 = local write "MTrig_Audio_trig__R"(w1095) -> ()
              n553 = local write "MTrig_Laser_trig"(w1095) -> ()
            }
          }
          n554 = case shown="\"SelectReward\"" w1071 {
            selector: w1071 -> [_ _ _ _ _ _ _ _ _ _ _ _ _ _ _ _ _ _ _ _ w1832 _ w1897 _ _ _ _ _ w2039 _ w2114 _ _ _ _ _ w2243 _ w2319 _ w2383 _ w2427 _ _ w2497 _ _ _ _ _ w2669 _ _ _ _ _ _ _ _ _ _ _ _ _ _ _ _ _ _ _]
            tunnel: [myRIO_BRig_RT__Case_Exp_stateList."Start2" ("Enum") myRIO_BRig_RT__Case_Exp_stateList."Start3" ("Enum") myRIO_BRig_RT__Case_Exp_stateList."saveSettings1" ("Enum") myRIO_BRig_RT__Case_Exp_stateList."saveSettings2" ("Enum") myRIO_BRig_RT__Case_Exp_stateList."saveSettings3" ("Enum") myRIO_BRig_RT__Case_Exp_stateList."saveSettings4_LC_ENL" ("Enum") myRIO_BRig_RT__Case_Exp_stateList."saveSettings5_LC_Cue" ("Enum") myRIO_BRig_RT__Case_Exp_stateList."saveSettings6_LC_Other" ("Enum") myRIO_BRig_RT__Case_Exp_stateList."setSettings_Audio" ("Enum") myRIO_BRig_RT__Case_Exp_stateList."setSettings_Laser" ("Enum") myRIO_BRig_RT__Case_Exp_stateList."commConnect" ("Enum") w1593 myRIO_BRig_RT__Case_Exp_stateList."initTrial" ("Enum") w1637 myRIO_BRig_RT__Case_Exp_stateList."initTrial3" ("Enum") myRIO_BRig_RT__Case_Exp_stateList."initTrial_LC_ENL1" ("Enum") myRIO_BRig_RT__Case_Exp_stateList."ENL1_pre" ("Enum") myRIO_BRig_RT__Case_Exp_stateList."initTrial_LC_Cue1" ("Enum") myRIO_BRig_RT__Case_Exp_stateList."initTrial4" ("Enum") w1791 w1829 myRIO_BRig_RT__Case_Exp_stateList."ENL1Penalty" ("Enum") w1898 myRIO_BRig_RT__Case_Exp_stateList."endExp" ("Enum") myRIO_BRig_RT__Case_Exp_stateList."endExp" ("Enum") myRIO_BRig_RT__Case_Exp_stateList."endExp" ("Enum") myRIO_BRig_RT__Case_Exp_stateList."endExp" ("Enum") w1993 w2038 myRIO_BRig_RT__Case_Exp_stateList."Cue1Penalty" ("Enum") w2112 myRIO_BRig_RT__Case_Exp_stateList."endExp" ("Enum") myRIO_BRig_RT__Case_Exp_stateList."endExp" ("Enum") myRIO_BRig_RT__Case_Exp_stateList."endExp" ("Enum") myRIO_BRig_RT__Case_Exp_stateList."endExp" ("Enum") w2200 w2251 myRIO_BRig_RT__Case_Exp_stateList."SelectReward" ("Enum") w2320 myRIO_BRig_RT__Case_Exp_stateList."SelectRewardPost" ("Enum") w2384 myRIO_BRig_RT__Case_Exp_stateList."SelectWrong" ("Enum") w2423 myRIO_BRig_RT__Case_Exp_stateList."endTrial1" ("Enum") myRIO_BRig_RT__Case_Exp_stateList."SelectTimeout" ("Enum") w2499 myRIO_BRig_RT__Case_Exp_stateList."endTrial1" ("Enum") myRIO_BRig_RT__Case_Exp_stateList."endTrial2" ("Enum") myRIO_BRig_RT__Case_Exp_stateList."saveData_dataBlock" ("Enum") w2582 w2652 w2669 myRIO_BRig_RT__Case_Exp_stateList."initBlock" ("Enum") w2696 myRIO_BRig_RT__Case_Exp_stateList."commUpload_dataCurrent" ("Enum") myRIO_BRig_RT__Case_Exp_stateList."commUpload_dataExp" ("Enum") myRIO_BRig_RT__Case_Exp_stateList."commUpload_dataLC" ("Enum") myRIO_BRig_RT__Case_Exp_stateList."commUpload_dataTrial" ("Enum") myRIO_BRig_RT__Case_Exp_stateList."endTrial3" ("Enum") myRIO_BRig_RT__Case_Exp_stateList."saveData_dataCurrent" ("Enum") myRIO_BRig_RT__Case_Exp_stateList."saveData_dataExp" ("Enum") myRIO_BRig_RT__Case_Exp_stateList."saveData_dataLC" ("Enum") myRIO_BRig_RT__Case_Exp_stateList."saveData_dataTrial" ("Enum") myRIO_BRig_RT__Case_Exp_stateList."commUpload_pre" ("Enum") myRIO_BRig_RT__Case_Exp_stateList."empty_endBlock2" ("Enum") myRIO_BRig_RT__Case_Exp_stateList."initBlock" ("Enum") myRIO_BRig_RT__Case_Exp_stateList."empty_endTrial2" ("Enum") myRIO_BRig_RT__Case_Exp_stateList."empty_endTrial3" ("Enum") myRIO_BRig_RT__Case_Exp_stateList."empty_endTrial4" ("Enum") myRIO_BRig_RT__Case_Exp_stateList."empty_endTrial5" ("Enum") myRIO_BRig_RT__Case_Exp_stateList."initTrial" ("Enum")] -> w1040
            tunnel: [w1121 w1140 w1162 w1217 w1265 w1332 w1384 w1436 w1480 w1506 w1565 w1569 w1601 w1618 w1653 w1683 w1716 w1740 w1766 w1807 w1845 w1875 w1902 w1918 w1940 w1959 w1978 w2012 w2060 w2085 w2111 w2132 w2153 w2172 w2191 w2211 w2269 w2294 w2317 w2331 w2381 w2405 w2437 w2458 w2478 w2510 w2533 w2545 w2564 w2606 w2625 w2668 w2685 w2699 w2733 w2754 w2775 w2796 w2817 w2845 w2865 w2892 w2912 w2937 w2956 w2975 w2994 w3013 w3032 w3051 w3070] -> w1092
            tunnel: w1094 -> [w1121 w1140 w1162 w1217 w1265 w1332 w1384 w1436 w1480 w1506 w1565 w1592 w1601 w1618 w1653 w1683 w1716 w1740 w1766 w1807 w1845 w1875 w1902 w1918 w1940 w1959 w1978 w2012 w2060 w2085 w2111 w2132 w2153 w2172 w2191 w2211 w2269 w2294 w2317 w2331 w2381 w2405 w2437 w2458 w2478 w2510 w2533 w2545 w2564 w2606 w2625 w2668 w2685 w2699 w2733 w2754 w2775 w2796 w2817 w2845 w2865 w2892 w2912 w2937 w2956 w2975 w2994 w3013 w3032 w3051 w3070]
            tunnel: w1093 -> [w1124 w1143 w1159 w1220 w1268 w1335 w1387 w1439 w1483 w1509 w1568 w1586 w1612 w1638 w1671 w1699 w1730 w1753 w1779 w1794 w1826 w1878 w1905 w1924 w1943 w1962 w1981 w1992 w2037 w2093 w2118 w2137 w2156 w2175 w2194 w2209 w2267 w2304 w2327 w2362 w2389 w2416 w2440 w2457 w2490 w2515 w2530 w2553 w2563 w2617 w2651 w2672 w2682 w2708 w2736 w2757 w2778 w2799 w2820 w2848 w2868 w2895 w2915 w2940 w2959 w2978 w2997 w3016 w3035 w3054 w3073]
            tunnel: w1087 -> [w1123 w1142 w1160 w1219 w1267 w1334 w1386 w1438 w1482 w1508 w1567 w1585 w1611 w1639 w1670 w1700 w1731 w1754 w1780 w1817 w1847 w1877 w1904 w1923 w1942 w1961 w1980 w2026 w2061 w2092 w2117 w2136 w2155 w2174 w2193 w2210 w2266 w2303 w2326 w2361 w2388 w2415 w2439 w2456 w2489 w2514 w2531 w2554 w2562 w2616 w2650 w2671 w2683 w2709 w2735 w2756 w2777 w2798 w2819 w2847 w2867 w2894 w2914 w2939 w2958 w2977 w2996 w3015 w3034 w3053 w3072]
            tunnel: w1086 -> [w1122 w1141 w1161 w1218 w1266 w1333 w1385 w1437 w1481 w1507 w1566 w1584 w1610 w1640 w1669 w1701 w1732 w1755 w1781 w1816 w1846 w1876 w1903 w1922 w1941 w1960 w1979 w2025 w2062 w2091 w2116 w2135 w2154 w2173 w2192 w2229 w2270 w2302 w2325 w2360 w2387 w2414 w2438 w2455 w2488 w2513 w2532 w2555 w2561 w2615 w2649 w2670 w2684 w2710 w2734 w2755 w2776 w2797 w2818 w2846 w2866 w2893 w2913 w2938 w2957 w2976 w2995 w3014 w3033 w3052 w3071]
            tunnel: [w1124 w1143 w1159 w1220 w1268 w1335 w1387 w1439 w1483 w1509 w1568 w1586 w1612 w1638 w1671 w1699 w1730 w1753 w1779 w1794 w1826 w1878 w1905 w1924 w1943 w1962 w1981 w1992 w2037 w2093 w2118 w2137 w2156 w2175 w2194 w2209 w2267 w2304 w2327 w2362 w2389 w2416 w2440 w2457 w2490 w2515 w2530 w2553 w2563 w2617 w2651 w2672 w2682 w2708 w2736 w2757 w2778 w2799 w2820 w2848 w2868 w2895 w2915 w2940 w2959 w2978 w2997 w3016 w3035 w3054 w3073] -> w1074
            tunnel: [w1123 w1142 w1160 w1219 w1267 w1334 w1386 w1438 w1482 w1508 w1567 w1585 w1611 w1639 w1670 w1700 w1731 w1754 w1780 w1817 w1847 w1877 w1904 w1923 w1942 w1961 w1980 w2026 w2061 w2092 w2117 w2136 w2155 w2174 w2193 w2210 w2266 w2303 w2326 w2361 w2388 w2415 w2439 w2456 w2489 w2514 w2531 w2554 w2562 w2616 w2650 w2671 w2683 w2709 w2735 w2756 w2777 w2798 w2819 w2847 w2867 w2894 w2914 w2939 w2958 w2977 w2996 w3015 w3034 w3053 w3072] -> w1073
            tunnel: [w1122 w1141 w1161 w1218 w1266 w1333 w1385 w1437 w1481 w1507 w1566 w1584 w1610 w1640 w1669 w1701 w1732 w1755 w1781 w1816 w1846 w1876 w1903 w1922 w1941 w1960 w1979 w2025 w2062 w2091 w2116 w2135 w2154 w2173 w2192 w2229 w2270 w2302 w2325 w2360 w2387 w2414 w2438 w2455 w2488 w2513 w2532 w2555 w2561 w2615 w2649 w2670 w2684 w2710 w2734 w2755 w2776 w2797 w2818 w2846 w2866 w2893 w2913 w2938 w2957 w2976 w2995 w3014 w3033 w3052 w3071] -> w1072
            tunnel: w1032 -> [w1120 w1139 w1158 w1184 w1241 w1309 w1383 w1435 w1479 w1504 w1525 w1591 w1600 w1636 w1642 w1684 w1711 w1737 w1765 w1806 w1831 w1869 w1901 w1919 w1939 w1958 w1977 w1996 w2057 w2084 w2115 w2133 w2152 w2171 w2190 w2220 w2247 w2286 w2322 w2333 w2386 w2406 w2436 w2454 w2479 w2512 w2529 w2542 w2566 w2586 w2623 w2667 w2686 w2711 w2730 w2751 w2772 w2793 w2804 w2834 w2853 w2877 w2909 w2926 w2946 w2965 w2984 w3003 w3022 w3041 w3060]
            tunnel: w1027 -> [w1119 w1138 w1157 w1215 w1263 w1329 w1381 w1433 w1477 w1497 w1561 w1590 w1609 w1635 w1650 w1682 w1718 w1743 w1769 w1809 w1844 w1868 w1899 w1921 w1938 w1957 w1976 w2014 w2059 w2082 w2110 w2134 w2151 w2170 w2189 w2222 w2268 w2300 w2324 w2354 w2382 w2407 w2434 w2453 w2481 w2509 w2528 w2552 w2569 w2585 w2642 w2666 w2687 w2712 w2729 w2750 w2771 w2792 w2805 w2842 w2862 w2873 w2908 w2934 w2953 w2972 w2991 w3010 w3029 w3048 w3067]
            tunnel: [w1120 w1139 w1158 w1184 w1241 w1308 w1383 w1435 w1479 w1504 w1547 w1575 w1600 w1624 w1642 w1684 w1711 w1736 w1764 w1810 w1830 w1870 w1900 w1919 w1939 w1958 w1977 w2021 w2056 w2083 w2113 w2133 w2152 w2171 w2190 w2223 w2242 w2301 w2321 w2355 w2385 w2408 w2435 w2454 w2482 w2511 w2529 w2541 w2565 w2586 w2621 w2667 w2686 w2711 w2730 w2751 w2772 w2793 w2804 w2834 w2853 w2877 w2909 w2926 w2946 w2965 w2984 w3003 w3022 w3041 w3060] -> w1068
            tunnel: [w1119 w1138 w1157 w1214 w1262 w1324 w1381 w1433 w1477 w1497 w1561 w1589 w1609 w1634 w1650 w1682 w1718 w1743 w1769 w1809 w1844 w1868 w1899 w1921 w1938 w1957 w1976 w2014 w2059 w2082 w2110 w2134 w2151 w2170 w2189 w2222 w2268 w2300 w2324 w2354 w2382 w2407 w2434 w2453 w2481 w2509 w2528 w2552 w2569 w2585 w2642 w2666 w2687 w2712 w2729 w2750 w2771 w2792 w2805 w2842 w2862 w2876 w2908 w2934 w2953 w2972 w2991 w3010 w3029 w3048 w3067] -> w1083
            tunnel: [_ _ _ _ _ _ _ _ _ _ _ _ _ _ _ _ _ _ _ _ _ _ _ _ _ _ _ _ _ _ _ _ _ _ _ _ _ _ w2315 _ _ _ _ _ _ _ _ _ _ _ _ _ _ _ _ _ _ _ _ _ _ _ _ _ _ _ _ _ _ _ _] -> w1043
            tunnel: [_ _ _ _ _ _ _ _ _ _ _ _ _ _ _ _ _ _ _ _ _ _ _ _ _ _ _ _ _ _ _ _ _ _ _ _ _ _ w2316 _ _ _ _ _ _ _ _ _ _ _ _ _ _ _ _ _ _ _ _ _ _ _ _ _ _ _ _ _ _ _ _] -> w1045
            tunnel: w1082 -> [w1117 w1136 w1155 w1186 w1243 w1330 w1382 w1434 w1478 w1502 w1562 w1587 w1602 w1632 w1662 w1697 w1728 w1733 w1761 w1808 w1843 w1865 w1895 w1920 w1936 w1955 w1974 w2020 w2058 w2081 w2108 w2130 w2149 w2168 w2187 w2221 w2264 w2292 w2323 w2335 w2379 w2404 w2432 w2451 w2480 w2508 w2526 w2544 w2571 w2613 w2634 w2664 w2689 w2714 w2727 w2748 w2769 w2790 w2814 w2828 w2855 w2883 w2902 w2928 w2947 w2966 w2985 w3004 w3023 w3042 w3061]
            tunnel: [w1117 w1136 w1155 w1186 w1243 w1330 w1382 w1434 w1478 w1502 w1562 w1587 w1599 w1632 w1662 w1697 w1728 w1733 w1761 w1808 w1843 w1865 w1895 w1920 w1936 w1955 w1974 w2020 w2058 w2081 w2108 w2130 w2149 w2168 w2187 w2221 w2264 w2292 w2323 w2334 w2379 w2404 w2432 w2451 w2480 w2508 w2526 w2543 w2571 w2613 w2634 w2664 w2689 w2714 w2727 w2748 w2769 w2790 w2814 w2828 w2855 w2883 w2902 w2928 w2947 w2966 w2985 w3004 w3023 w3042 w3061] -> w1081
            tunnel: w1080 -> [w1118 w1137 w1156 w1185 w1242 w1331 w1379 w1431 w1475 w1503 w1563 w1588 w1608 w1633 w1641 w1698 w1729 w1741 w1767 w1805 w1825 w1866 w1896 w1917 w1937 w1956 w1975 w2019 w2036 w2080 w2109 w2131 w2150 w2169 w2188 w2219 w2265 w2293 w2318 w2352 w2380 w2403 w2433 w2452 w2477 w2506 w2527 w2551 w2570 w2614 w2641 w2665 w2688 w2713 w2728 w2749 w2770 w2791 w2815 w2841 w2861 w2889 w2900 w2933 w2952 w2971 w2990 w3009 w3028 w3047 w3066]
            tunnel: [w1118 w1137 w1156 w1185 w1242 w1331 w1380 w1432 w1476 w1503 w1563 w1588 w1608 w1633 w1641 w1698 w1729 w1741 w1767 w1805 w1825 w1866 w1896 w1917 w1937 w1956 w1975 w2019 w2036 w2080 w2109 w2131 w2150 w2169 w2188 w2219 w2265 w2293 w2318 w2352 w2380 w2403 w2433 w2452 w2477 w2506 w2527 w2551 w2570 w2614 w2641 w2665 w2688 w2713 w2728 w2749 w2770 w2791 w2815 w2841 w2861 w2889 w2900 w2933 w2952 w2971 w2990 w3009 w3028 w3047 w3066] -> w1079
            tunnel: w1078 -> [_ _ _ _ _ _ _ _ _ _ _ _ _ _ _ _ _ _ _ w1790 w1818 w1851 w1884 _ _ _ _ _ w2030 w2067 _ _ _ _ _ _ _ _ _ _ _ _ _ _ _ w2507 _ _ _ _ _ _ _ _ _ _ _ _ _ _ _ _ _ _ _ _ _ _ _ _ _]
            tunnel: [_ _ _ _ _ _ _ _ _ _ _ _ _ _ _ _ _ _ _ _ _ _ _ _ _ _ _ _ _ _ _ _ _ _ _ _ _ _ _ _ _ _ _ _ _ _ _ _ _ _ _ TRUE _ _ _ _ _ _ _ _ _ _ _ _ _ _ _ _ _ _ _] -> w1075
            tunnel: w1064 -> [w1115 w1134 w1153 w1176 w1236 w1319 w1366 w1418 w1447 _ w1553 w1583 w1607 w1631 w1661 w1696 w1727 w1752 w1778 w1804 w1842 w1863 w1894 w1915 w1934 w1953 w1972 w2018 w2053 w2078 w2107 w2128 w2147 w2166 w2185 w2218 w2263 w2282 w2314 w2350 w2378 w2401 w2431 w2450 w2475 w2505 w2525 w2549 w2575 w2612 w2638 w2662 w2680 w2707 w2725 w2746 w2767 w2788 w2812 w2839 w2859 w2887 w2906 w2932 w2951 w2970 w2989 w3008 w3027 w3046 w3065]
            tunnel: w1063 -> [w1114 w1133 w1152 w1175 w1235 w1318 w1365 w1417 w1448 _ w1552 w1582 w1606 w1630 w1660 w1695 w1726 w1751 w1777 w1803 w1841 w1862 w1893 w1914 w1933 w1952 w1971 w2017 w2052 w2077 w2106 w2127 w2146 w2165 w2184 w2217 w2262 w2281 w2313 w2349 w2377 w2400 w2430 w2449 w2474 w2504 w2524 w2548 w2574 w2611 w2637 w2661 w2679 w2706 w2724 w2745 w2766 w2787 w2811 w2838 w2858 w2886 w2905 w2931 w2950 w2969 w2988 w3007 w3026 w3045 w3064]
            tunnel: w1062 -> [w1113 w1132 w1151 w1174 w1234 w1317 w1364 w1416 w1449 _ w1551 w1581 w1605 w1629 w1659 w1694 w1725 w1750 w1776 w1802 w1840 w1861 w1892 w1913 w1932 w1951 w1970 w2016 w2051 w2076 w2105 w2126 w2145 w2164 w2183 w2216 w2261 w2280 w2312 w2348 w2376 w2399 w2429 w2448 w2473 w2503 w2523 w2547 w2573 w2610 w2636 w2660 w2678 w2705 w2723 w2744 w2765 w2786 w2810 w2837 w2857 w2885 w2904 w2930 w2949 w2968 w2987 w3006 w3025 w3044 w3063]
            tunnel: w1061 -> [w1112 w1131 w1150 w1173 w1233 w1316 w1363 w1415 w1450 _ w1550 w1580 w1604 w1628 w1658 w1693 w1724 w1749 w1775 w1801 w1839 w1860 w1891 w1912 w1931 w1950 w1969 w2015 w2050 w2075 w2104 w2125 w2144 w2163 w2182 w2215 w2260 w2279 w2311 w2347 w2375 w2398 w2428 w2447 w2472 w2502 w2522 w2546 w2572 w2609 w2635 w2659 w2677 w2704 w2722 w2743 w2764 w2785 w2809 w2836 w2856 w2884 w2903 w2929 w2948 w2967 w2986 w3005 w3024 w3043 w3062]
            tunnel: w1060 -> [_ _ _ _ _ _ _ _ _ _ _ _ _ _ _ _ _ _ _ _ _ _ _ _ _ _ _ _ w2055 _ _ _ _ _ _ _ _ _ _ _ _ _ _ _ _ _ _ _ _ _ _ _ _ _ _ _ _ _ _ _ _ _ _ _ _ _ _ _ _ _ _]
            tunnel: w1059 -> [_ _ _ _ _ _ _ _ _ _ _ _ _ _ _ _ _ _ _ _ _ _ _ _ _ _ _ _ w2054 _ _ _ _ _ _ _ _ _ _ _ _ _ _ _ _ _ _ _ _ _ _ _ _ _ _ _ _ _ _ _ _ _ _ _ _ _ _ _ _ _ _]
            tunnel: [w1115 w1134 w1153 w1176 w1236 w1319 w1366 w1418 w1447 w1496 w1553 w1583 w1607 w1631 w1661 w1696 w1727 w1752 w1778 w1804 w1842 w1863 w1894 w1915 w1934 w1953 w1972 w2018 w2053 w2078 w2107 w2128 w2147 w2166 w2185 w2218 w2263 w2282 w2314 w2350 w2378 w2401 w2431 w2450 w2475 w2505 w2525 w2549 w2575 w2612 w2638 w2662 w2680 w2707 w2725 w2746 w2767 w2788 w2812 w2839 w2859 w2887 w2906 w2932 w2951 w2970 w2989 w3008 w3027 w3046 w3065] -> w1056
            tunnel: [w1114 w1133 w1152 w1175 w1235 w1318 w1365 w1417 w1448 w1487 w1552 w1582 w1606 w1630 w1660 w1695 w1726 w1751 w1777 w1803 w1841 w1862 w1893 w1914 w1933 w1952 w1971 w2017 w2052 w2077 w2106 w2127 w2146 w2165 w2184 w2217 w2262 w2281 w2313 w2349 w2377 w2400 w2430 w2449 w2474 w2504 w2524 w2548 w2574 w2611 w2637 w2661 w2679 w2706 w2724 w2745 w2766 w2787 w2811 w2838 w2858 w2886 w2905 w2931 w2950 w2969 w2988 w3007 w3026 w3045 w3064] -> w1024
            tunnel: [w1113 w1132 w1151 w1174 w1234 w1317 w1364 w1416 w1449 w1495 w1551 w1581 w1605 w1629 w1659 w1694 w1725 w1750 w1776 w1802 w1840 w1861 w1892 w1913 w1932 w1951 w1970 w2016 w2051 w2076 w2105 w2126 w2145 w2164 w2183 w2216 w2261 w2280 w2312 w2348 w2376 w2399 w2429 w2448 w2473 w2503 w2523 w2547 w2573 w2610 w2636 w2660 w2678 w2705 w2723 w2744 w2765 w2786 w2810 w2837 w2857 w2885 w2904 w2930 w2949 w2968 w2987 w3006 w3025 w3044 w3063] -> w1057
            tunnel: [w1112 w1131 w1150 w1173 w1233 w1316 w1363 w1415 w1450 w1485 w1550 w1580 w1604 w1628 w1658 w1693 w1724 w1749 w1775 w1801 w1839 w1860 w1891 w1912 w1931 w1950 w1969 w2015 w2050 w2075 w2104 w2125 w2144 w2163 w2182 w2215 w2260 w2279 w2311 w2347 w2375 w2398 w2428 w2447 w2472 w2502 w2522 w2546 w2572 w2609 w2635 w2659 w2677 w2704 w2722 w2743 w2764 w2785 w2809 w2836 w2856 w2884 w2903 w2929 w2948 w2967 w2986 w3005 w3024 w3043 w3062] -> w1058
            tunnel: [_ _ _ _ _ _ _ _ _ _ _ _ _ _ _ _ _ _ _ _ _ _ _ _ _ _ _ w2005 w2055 _ _ _ _ _ _ _ _ _ _ _ _ _ _ _ _ _ _ _ _ _ _ _ _ _ _ _ _ _ _ _ _ _ _ _ _ _ _ _ _ _ _] -> w1026
            tunnel: [_ _ _ _ _ _ _ _ _ _ _ _ _ _ _ _ _ _ _ _ _ _ _ _ _ _ _ w2004 w2054 _ _ _ _ _ _ _ _ _ _ _ _ _ _ _ _ _ _ _ _ _ _ _ _ _ _ _ _ _ _ _ _ _ _ _ _ _ _ _ _ _ _] -> w1025
            tunnel: w1039 -> [w1111 w1130 w1149 w1172 w1232 w1315 w1362 w1414 w1446 w1494 w1560 w1579 w1603 w1627 w1644 w1686 w1710 w1735 w1763 w1800 w1838 w1859 w1890 w1911 w1930 w1949 w1968 w2003 w2049 w2074 w2103 w2124 w2143 w2162 w2181 w2214 w2259 w2276 w2310 w2346 w2374 w2395 w2422 w2446 w2469 w2496 w2521 w2540 w2568 w2602 w2633 w2658 w2690 w2715 w2726 w2747 w2768 w2789 w2813 w2840 w2860 w2888 w2907 w2923 w2945 w2964 w2983 w3002 w3021 w3040 w3059]
            tunnel: [w1111 w1130 w1149 w1172 w1232 w1315 w1362 w1414 w1446 w1494 w1560 w1579 w1603 w1627 w1643 w1685 w1703 w1734 w1762 w1800 w1838 w1859 w1890 w1911 w1930 w1949 w1968 w2003 w2049 w2074 w2103 w2124 w2143 w2162 w2181 w2214 w2259 w2276 w2310 w2346 w2374 w2395 w2422 w2446 w2469 w2496 w2521 w2540 w2567 w2602 w2633 w2658 w2690 w2715 w2726 w2747 w2768 w2789 w2813 w2840 w2860 w2888 w2907 w2923 w2945 w2964 w2983 w3002 w3021 w3040 w3059] -> w1038
            tunnel: [w1110 w1129 w1148 w1171 w1231 w1314 w1361 w1413 w1445 w1493 w1559 w1578 w1614 w1626 w1664 w1692 w1723 w1748 w1774 w1799 w1837 w1858 w1889 w1910 w1929 w1948 w1967 w2002 w2048 w2073 w2102 w2123 w2142 w2161 w2180 w2213 w2258 w2275 w2309 w2345 w2373 w2394 w2421 w2445 w2468 w2495 w2520 w2539 w2560 w2608 w2632 w2656 w2691 w2701 w2721 w2742 w2763 w2784 w2808 w2844 w2864 w2891 w2911 w2936 w2955 w2974 w2993 w3012 w3031 w3050 w3069] -> w1037
            tunnel: [w1109 w1128 w1147 w1170 w1230 w1313 w1360 w1412 w1444 w1492 w1558 w1577 w1613 w1625 w1663 w1691 w1722 w1747 w1773 w1798 w1836 w1857 w1888 w1909 w1928 w1947 w1966 w2001 w2047 w2072 w2101 w2122 w2141 w2160 w2179 w2212 w2257 w2274 w2308 w2344 w2372 w2393 w2420 w2444 w2467 w2494 w2519 w2538 w2559 w2607 w2631 w2657 w2673 w2698 w2731 w2752 w2773 w2794 w2816 w2843 w2863 w2890 w2910 w2935 w2954 w2973 w2992 w3011 w3030 w3049 w3068] -> w1036
            tunnel: w1035 -> [w1110 w1129 w1148 w1171 w1231 w1314 w1361 w1413 w1445 w1493 w1559 w1578 w1614 w1626 w1664 w1692 w1723 w1748 w1774 w1799 w1837 w1858 w1889 w1910 w1929 w1948 w1967 w2002 w2048 w2073 w2102 w2123 w2142 w2161 w2180 w2213 w2258 w2275 w2309 w2345 w2373 w2394 w2421 w2445 w2468 w2495 w2520 w2539 w2560 w2608 w2632 w2656 _ w2701 w2721 w2742 w2763 w2784 w2808 w2844 w2864 w2891 w2911 w2936 w2955 w2974 w2993 w3012 w3031 w3050 w3069]
            tunnel: w1034 -> [w1109 w1128 w1147 w1170 w1230 w1313 w1360 w1412 w1444 w1492 w1558 w1577 w1613 w1625 w1663 w1691 w1722 w1747 w1773 w1798 w1836 w1857 w1888 w1909 w1928 w1947 w1966 w2001 w2047 w2072 w2101 w2122 w2141 w2160 w2179 w2212 w2257 w2274 w2308 w2344 w2372 w2393 w2420 w2444 w2467 w2494 w2519 w2538 w2559 w2607 w2631 w2657 _ w2698 w2731 w2752 w2773 w2794 w2816 w2843 w2863 w2890 w2910 w2935 w2954 w2973 w2992 w3011 w3030 w3049 w3068]
            tunnel: w1033 -> [_ _ _ _ _ _ _ _ _ _ _ _ _ _ _ _ _ _ _ _ _ _ _ _ _ _ _ _ _ _ _ _ _ _ _ _ _ _ _ _ _ _ _ _ _ _ _ _ _ _ _ _ _ _ w2719 w2740 w2761 w2782 w2806 _ _ _ _ _ _ _ _ _ _ _ _]
            tunnel: w1031 -> [_ _ _ _ _ _ _ _ _ _ _ _ _ _ _ _ w1715 _ w1758 w1787 w1823 w1849 w1880 _ _ _ _ w1983 w2028 w2066 w2095 _ _ _ _ _ _ _ _ _ _ _ _ _ _ _ _ _ _ _ _ _ _ _ _ _ _ _ _ _ _ _ _ _ _ _ _ _ _ _ _]
            tunnel: w1028 -> [_ _ _ _ _ _ _ _ _ _ _ _ _ _ _ _ _ _ _ _ _ _ _ _ _ _ _ _ _ _ _ _ _ _ _ _ _ _ _ _ _ _ _ _ _ _ _ _ _ _ _ _ _ _ _ _ _ _ _ _ _ w2878 _ _ _ _ _ _ _ _ _]
            tunnel: [w1108 w1127 w1146 w1169 w1229 w1312 w1359 w1411 w1443 w1491 w1557 w1572 w1597 w1621 w1665 w1690 w1721 w1746 w1772 w1797 w1835 w1856 w1887 w1908 w1927 w1946 w1965 w2000 w2046 w2071 w2100 w2121 w2140 w2159 w2178 w2208 w2256 w2273 w2307 w2329 w2371 w2392 w2419 w2443 w2466 w2493 w2518 w2537 w2558 w2605 w2618 w2655 w2676 w2700 w2718 w2739 w2760 w2781 w2803 w2823 w2852 w2872 w2899 w2919 w2944 w2963 w2982 w3001 w3020 w3039 w3058] -> w1022
            tunnel: w1023 -> [w1108 w1127 w1146 w1169 w1229 w1312 w1359 w1411 w1443 w1491 w1557 w1572 _ w1621 w1665 w1690 w1721 w1746 w1772 w1797 w1835 w1856 w1887 w1908 w1927 w1946 w1965 w2000 w2046 w2071 w2100 w2121 w2140 w2159 w2178 w2208 w2256 w2273 w2307 w2329 w2371 w2392 w2419 w2443 w2466 w2493 w2518 w2537 w2558 w2605 w2619 w2655 w2676 w2700 w2718 w2739 w2760 w2781 w2803 w2823 w2852 w2872 w2899 w2919 w2944 w2963 w2982 w3001 w3020 w3039 w3058]
            tunnel: w1021 -> [w1107 w1126 w1145 w1168 w1228 w1311 w1358 w1410 w1442 w1490 w1556 w1571 w1596 w1620 w1657 w1689 w1720 w1745 w1771 w1796 w1834 w1855 w1886 w1907 w1926 w1945 w1964 w1999 w2045 w2070 w2099 w2120 w2139 w2158 w2177 w2207 w2255 w2272 w2306 w2343 w2370 w2391 w2418 w2442 w2465 w2492 w2517 w2536 w2557 w2604 w2630 w2654 w2675 w2703 w2717 w2738 w2759 w2780 w2802 w2822 w2851 w2871 w2898 w2918 w2943 w2962 w2981 w3000 w3019 w3038 w3057]
            tunnel: w1020 -> [w1106 w1125 w1144 w1167 w1227 w1310 w1357 w1409 w1441 w1489 w1555 w1570 w1595 w1619 w1656 w1688 w1719 w1744 w1770 w1795 w1833 w1854 w1885 w1906 w1925 w1944 w1963 w1998 w2044 w2069 w2098 w2119 w2138 w2157 w2176 w2206 w2254 w2271 w2305 w2340 w2369 w2390 w2417 w2441 w2464 w2491 w2516 w2535 w2556 w2603 w2629 w2653 w2674 w2702 w2716 w2737 w2758 w2779 w2801 w2821 w2850 w2870 w2897 w2917 w2942 w2961 w2980 w2999 w3018 w3037 w3056]
            tunnel: [w1107 w1126 w1145 w1168 w1228 w1311 w1358 w1410 w1442 w1490 w1556 w1571 w1596 w1620 w1657 w1689 w1720 w1745 w1771 w1796 w1834 w1855 w1886 w1907 w1926 w1945 w1964 w1999 w2045 w2070 w2099 w2120 w2139 w2158 w2177 w2207 w2255 w2272 w2306 w2342 w2370 w2391 w2418 w2442 w2465 w2492 w2517 w2536 w2557 w2604 w2630 w2654 w2675 w2703 w2717 w2738 w2759 w2780 w2802 w2822 w2851 w2871 w2898 w2918 w2943 w2962 w2981 w3000 w3019 w3038 w3057] -> w1019
            tunnel: [w1106 w1125 w1144 w1167 w1227 w1310 w1357 w1409 w1441 w1489 w1555 w1570 w1595 w1619 w1656 w1688 w1719 w1744 w1770 w1795 w1833 w1854 w1885 w1906 w1925 w1944 w1963 w1998 w2044 w2069 w2098 w2119 w2138 w2157 w2176 w2206 w2254 w2271 w2305 w2341 w2369 w2390 w2417 w2441 w2464 w2491 w2516 w2535 w2556 w2603 w2629 w2653 w2674 w2702 w2716 w2737 w2758 w2779 w2801 w2821 w2850 w2870 w2897 w2917 w2942 w2961 w2980 w2999 w3018 w3037 w3056] -> w1018
            tunnel: w1017 -> [_ _ _ _ _ _ _ _ _ _ w1548 _ _ _ w1668 w1678 _ _ _ _ _ _ _ _ _ _ _ _ w2041 _ _ _ _ _ _ w2204 w2253 _ _ _ _ _ _ _ w2463 _ _ _ _ w2580 _ _ _ _ _ _ _ _ _ _ _ _ _ _ _ _ _ _ _ _ _]
            tunnel: w1016 -> [_ _ _ _ _ _ _ _ _ _ w1549 _ _ _ w1667 w1677 _ _ _ _ _ _ _ _ _ _ _ _ w2040 _ _ _ _ _ _ w2205 w2252 _ _ _ _ _ _ _ w2462 _ _ _ _ w2579 _ _ _ _ _ _ _ _ _ _ _ _ _ _ _ _ _ _ _ _ _]
            tunnel: w1014 -> [_ _ _ _ _ _ _ _ _ _ _ _ _ _ _ _ w1714 _ w1757 w1786 w1822 w1848 w1881 _ _ _ _ w1982 w2027 w2065 w2094 _ _ _ _ _ _ _ _ _ _ _ _ _ _ _ _ _ _ _ _ _ _ _ _ _ _ _ _ _ _ _ _ _ _ _ _ _ _ _ _]
            tunnel: [_ _ _ _ _ _ _ _ _ _ _ _ _ _ _ _ _ _ _ w1790 w1824 w1851 w1884 _ _ _ _ TRUE w2030 w2067 _ _ _ _ _ _ _ _ _ _ _ _ _ _ _ _ _ _ _ _ _ _ _ _ _ _ _ _ _ _ _ _ _ _ _ _ _ _ _ _ _] -> w1013
            tunnel: w1012 -> [_ _ _ _ _ _ _ _ _ _ _ _ _ _ _ _ w1713 _ _ w1789 w1828 w1853 w1882 _ _ _ _ w1990 w2035 w2064 w2097 _ _ _ _ _ _ _ _ _ _ _ _ _ _ _ _ _ _ _ _ _ _ _ _ _ _ _ _ _ _ _ _ _ _ _ _ _ _ _ _]
            tunnel: w1011 -> [_ _ _ _ _ _ _ _ _ _ _ _ _ _ _ _ w1712 _ _ w1788 w1827 w1852 w1883 _ _ _ _ w1989 w2034 w2063 w2096 _ _ _ _ _ _ _ _ _ _ _ _ _ _ _ _ _ _ _ _ _ _ _ _ _ _ _ _ _ _ _ _ _ _ _ _ _ _ _ _]
            tunnel: [_ _ _ _ _ _ _ _ _ _ _ _ _ _ _ _ w1713 _ w1760 w1789 w1828 w1853 w1882 _ _ _ _ w1990 w2035 w2064 w2097 _ _ _ _ _ _ _ _ _ _ _ _ _ _ _ _ _ _ _ _ _ _ _ _ _ _ _ _ _ _ _ _ _ _ _ _ _ _ _ _] -> w1010
            tunnel: [_ _ _ _ _ _ _ _ _ _ _ _ _ _ _ _ w1712 _ w1759 w1788 w1827 w1852 w1883 _ _ _ _ w1989 w2034 w2063 w2096 _ _ _ _ _ _ _ _ _ _ _ _ _ _ _ _ _ _ _ _ _ _ _ _ _ _ _ _ _ _ _ _ _ _ _ _ _ _ _ _] -> w1009
            tunnel: [_ _ _ _ _ _ _ _ _ _ _ _ _ _ _ _ w1715 w1738 w1758 w1787 w1823 w1849 w1880 _ _ _ _ w1983 w2028 w2066 w2095 _ _ _ _ _ _ _ _ _ _ _ _ _ _ _ _ _ _ _ _ _ _ _ _ _ _ _ _ _ _ _ _ _ _ _ _ _ _ _ _] -> w1008
            tunnel: [_ _ _ _ _ _ _ _ _ _ _ _ _ _ _ _ w1714 w1739 w1757 w1786 w1822 w1848 w1881 _ _ _ _ w1982 w2027 w2065 w2094 _ _ _ _ _ _ _ _ _ _ _ _ _ _ _ _ _ _ _ _ _ _ _ _ _ _ _ _ _ _ _ _ _ _ _ _ _ _ _ _] -> w1007
            tunnel: [_ _ _ _ _ _ _ _ _ _ _ _ _ _ _ _ _ _ _ _ w1821 _ _ _ _ _ _ _ w2032 _ _ _ _ _ _ _ _ _ _ _ _ _ _ _ _ _ _ _ _ _ _ _ _ _ _ _ _ _ _ _ _ _ _ _ _ _ _ _ _ _ _] -> w1004
            tunnel: [_ _ _ _ _ _ _ _ _ _ _ _ _ _ _ _ _ _ _ _ w1820 _ _ _ _ _ _ _ w2033 _ _ _ _ _ _ _ _ _ _ _ _ _ _ _ _ _ _ _ _ _ _ _ _ _ _ _ _ _ _ _ _ _ _ _ _ _ _ _ _ _ _] -> w1006
            tunnel: w1001 -> [_ _ _ _ _ _ _ _ _ _ _ _ _ _ _ _ _ _ _ w1785 w1819 w1850 w1879 _ _ _ _ w1985 w2029 w2068 _ _ _ _ _ _ _ _ _ _ _ _ _ _ _ _ _ _ _ _ _ _ _ _ _ _ _ _ _ _ _ _ _ _ _ _ _ _ _ _ _]
            tunnel: [_ _ _ _ _ _ _ _ _ _ _ _ _ _ _ _ _ _ _ w1785 w1819 w1850 w1879 _ _ _ _ w1985 w2031 w2068 _ _ _ _ _ _ _ _ _ _ _ _ _ _ _ _ _ _ _ _ _ _ _ _ _ _ _ _ _ _ _ _ _ _ _ _ _ _ _ _ _] -> w1000
            frame "Start1", Default {
            }
            frame "Start2" {
            }
            frame "Start3" {
            }
            frame "saveSettings1" {
              n555 = call "myRIO_BRig_RT_dataExp_Audio_freq__L.vi"() -> ("output_Audio_freq__L"=w1192:i32)  [unwired: 11 in]
              n556 = call "myRIO_BRig_RT_dataExp_Audio_freq__R.vi"() -> ("output_Audio_freq__R"=w1191:i32)  [unwired: 11 in]
              n557 = call "myRIO_BRig_RT_dataExp_Audio_amp__L.vi"() -> ("output_Audio_amp__L"=w1190:i32)  [unwired: 11 in]
              n558 = call "myRIO_BRig_RT_dataExp_Audio_amp__R.vi"() -> ("output_Audio_amp__R"=w1188:i32)  [unwired: 11 in]
              n559 = call "myRIO_BRig_RT_dataExp_TPB_min__L.vi"() -> ("output_TPB_min__L"=w1200:i32)  [unwired: 11 in]
              n560 = call "myRIO_BRig_RT_dataExp_TPB_min__R.vi"() -> ("output_TPB_min__R"=w1198:i32)  [unwired: 11 in]
              n561 = call "myRIO_BRig_RT_dataExp_TPB_max__L.vi"() -> ("output_TPB_max__L"=w1196:i32)  [unwired: 11 in]
              n562 = call "myRIO_BRig_RT_dataExp_TPB_max__R.vi"() -> ("output_TPB_max__R"=w1194:i32)  [unwired: 11 in]
              n563 = call "myRIO_BRig_RT_dataExp_ItrialUntilReward.vi"() -> ("output_I_trialUntilReward"=w1213:i32)  [unwired: 11 in]
              n564 = call "myRIO_BRig_RT_dataExp_IblockUntilReward.vi"() -> ("output_I_blockUntilReward"=w1209:i32)  [unwired: 11 in]
              n565 = call "myRIO_BRig_RT_dataExp_CueCycles.vi"() -> ("output_CueCycles"=w1208:i32)  [unwired: 11 in]
              n566 = call "myRIO_BRig_RT_dataExp_ENL_min.vi"() -> ("output_ENL_min"=w1206:i32)  [unwired: 11 in]
              n567 = call "myRIO_BRig_RT_dataExp_ENL_max.vi"() -> ("output_ENL_max"=w1204:i32)  [unwired: 11 in]
              n568 = call "myRIO_BRig_RT_dataExp_ENL_penalty.vi"() -> ("output_ENL_penalty"=w1202:i32)  [unwired: 11 in]
              n569 = local read "Audio_Freq__L"() -> (w1166:u8)
              n570 = local read "Audio_Freq__R"() -> (w1164:u8)
              n571 = local read "Audio_Amp__L"() -> (w1189:u16)
              n572 = local read "TpB_Min_L"() -> (w1199:u16)
              n573 = local read "TpB_Min_R"() -> (w1197:u16)
              n574 = local read "TpB_Max_L"() -> (w1195:u16)
              n575 = local read "TpB_Max_R"() -> (w1193:u16)
              n576 = local read "Audio_Amp__R"() -> (w1187:u16)
              n577 = local read "TrialUntilReward"() -> (w1212:bool)
              n578 = local read "CueCycles"() -> (w1207:u16)
              n579 = local read "Tcycle_ENL_min"() -> (w1205:u16)
              n580 = local read "Tcycle_ENL_max"() -> (w1203:u16)
              n581 = local read "Tcycle_ENLPenalty"() -> (w1201:u16)
              n582 = To Unsigned Word Integer(number=w1164) -> (unsigned 16bit integer=w1163:u16)
              n583 = To Unsigned Word Integer(number=w1166) -> (unsigned 16bit integer=w1165:u16)
              n584 = Boolean To (0,1)(Boolean=w1212) -> (0, 1=w1211:i16)
              n585 = To Unsigned Word Integer(number=w1211) -> (unsigned 16bit integer=w1210:u16)
              n586 = local read "BUR_min"() -> (w1181:u16)
              n587 = local read "BUR_max"() -> (w1182:u16)
              n588 = Not Equal To 0?(x=w1181) -> (x != 0?=w1180:bool)
              n589 = Not Equal To 0?(x=w1182) -> (x != 0?=w1179:bool)
              n590 = And(x=w1180, y=w1179) -> (x .and. y?=w1178:bool)
              n591 = Boolean To (0,1)(Boolean=w1178) -> (0, 1=w1183:i16)
              n592 = To Unsigned Word Integer(number=w1183) -> (unsigned 16bit integer=w1177:u16)
              n593 = Replace Array Subset(array=w1215, new element #1=w1210, index #1=w1213, new element #2=w1177, index #2=w1209, new element #3=w1207, index #3=w1208, new element #4=w1205, index #4=w1206, new element #5=w1203, index #5=w1204, new element #6=w1201, index #6=w1202, new element #7=w1199, index #7=w1200, new element #8=w1197, index #8=w1198, new element #9=w1195, index #9=w1196, new element #10=w1193, index #10=w1194, new element #11=w1165, index #11=w1192, new element #12=w1163, index #12=w1191, new element #13=w1189, index #13=w1190, new element #14=w1187, index #14=w1188) -> (w1214:u16[])
            }
            frame "saveSettings2" {
              n594 = call "myRIO_BRig_RT_dataExp_Tcycle_RewardPost.vi"() -> ("output_Tcycle_RewardPost"=w1252:i32)  [unwired: 11 in]
              n595 = call "myRIO_BRig_RT_dataExp_Tcycle_Wrong.vi"() -> ("output_Tcycle_Wrong"=w1250:i32)  [unwired: 11 in]
              n596 = call "myRIO_BRig_RT_dataExp_Tcycle_Timeout.vi"() -> ("output_Tcycle_Timeout"=w1248:i32)  [unwired: 11 in]
              n597 = call "myRIO_BRig_RT_dataExp_Tcycle_Cue_min.vi"() -> ("output_Tcycle_Cue_min"=w1246:i32)  [unwired: 11 in]
              n598 = call "myRIO_BRig_RT_dataExp_Tcycle_Cue_max.vi"() -> ("output_Tcycle_Cue_max"=w1245:i32)  [unwired: 11 in]
              n599 = call "myRIO_BRig_RT_dataExp_Tcycle_CuePenalty.vi"() -> ("output_Tcycle_CuePenalty"=w1244:i32)  [unwired: 11 in]
              n600 = call "myRIO_BRig_RT_dataExp_SolenoidProbability_L.vi"() -> ("output_SolenoidProbability_L"=w1224:i32)  [unwired: 11 in]
              n601 = call "myRIO_BRig_RT_dataExp_SolenoidProbability_R.vi"() -> ("output_SolenoidProbability_R"=w1223:i32)  [unwired: 11 in]
              n602 = call "myRIO_BRig_RT_dataExp_nBlock.vi"() -> ("output_nBlock"=w1261:i32)  [unwired: 11 in]
              n603 = call "myRIO_BRig_RT_dataExp_nTrial.vi"() -> ("output_nTrial"=w1260:i32)  [unwired: 11 in]
              n604 = call "myRIO_BRig_RT_dataExp_runTime_seconds.vi"() -> ("output_RunTime_minutes"=w1259:i32)  [unwired: 11 in]
              n605 = call "myRIO_BRig_RT_dataExp_Tcycle_Selection.vi"() -> ("output_Tcycle_Selection"=w1258:i32)  [unwired: 11 in]
              n606 = call "myRIO_BRig_RT_dataExp_Tcycle_Reward__L.vi"() -> ("output_Tcycle_Reward__L"=w1256:i32)  [unwired: 11 in]
              n607 = call "myRIO_BRig_RT_dataExp_Tcycle_Reward__R.vi"() -> ("output_Tcycle_Reward__R"=w1254:i32)  [unwired: 11 in]
              n608 = local read "Tcycle_RewardPost"() -> (w1251:u16)
              n609 = local read "Tcycle_Wrong"() -> (w1249:u16)
              n610 = local read "Tcycle_Timeout"() -> (w1247:u16)
              n611 = local read "Tcycle_CuePenalty"() -> (w1237:u16)
              n612 = local read "Tcycle_Cue_max"() -> (w1225:u16)
              n613 = local read "Tcycle_Cue_min"() -> (w1226:u16)
              n614 = local read "Tcycle_Selection"() -> (w1257:u16)
              n615 = local read "Tcycle_Reward_L"() -> (w1255:u16)
              n616 = local read "Tcycle_Reward_R"() -> (w1253:u16)
              n617 = local read "SolenoidProbability_R"() -> (w1221:u16)
              n618 = local read "SolenoidProbability_L"() -> (w1222:u16)
              n619 = Replace Array Subset(array=w1263, new element #1=u16 0, index #1=w1261, new element #2=u16 0, index #2=w1260, new element #3=u16 0, index #3=w1259, new element #4=w1257, index #4=w1258, new element #5=w1255, index #5=w1256, new element #6=w1253, index #6=w1254, new element #7=w1251, index #7=w1252, new element #8=w1249, index #8=w1250, new element #9=w1247, index #9=w1248, new element #10=w1226, index #10=w1246, new element #11=w1225, index #11=w1245, new element #12=w1237, index #12=w1244, new element #13=w1222, index #13=w1224, new element #14=w1221, index #14=w1223) -> (w1262:u16[])
            }
            frame "saveSettings3" {
              w1273 = 100.0 ("y")
              n620 = call "myRIO_BRig_RT_dataExp_laser_Freq.vi"() -> ("output_laser_Freq"=w1306:i32)  [unwired: 11 in]
              n621 = call "myRIO_BRig_RT_dataExp_laser_Tpeak.vi"() -> ("output_laser_Tpeak"=w1301:i32)  [unwired: 11 in]
              n622 = call "myRIO_BRig_RT_dataExp_laser_Tshutter.vi"() -> ("output_laser_Tshutter"=w1296:i32)  [unwired: 11 in]
              n623 = call "myRIO_BRig_RT_dataExp_laser_f_millisec2count.vi"() -> ("output_laser_f_millisec2count"=w1291:i32)  [unwired: 11 in]
              n624 = call "myRIO_BRig_RT_dataExp_laser_Power_min.vi"() -> ("output_laser_Power_min"=w1286:i32)  [unwired: 11 in]
              n625 = call "myRIO_BRig_RT_dataExp_laser_Power_max.vi"() -> ("output_laser_Power_max"=w1279:i32)  [unwired: 11 in]
              n626 = call "myRIO_BRig_RT_dataExp_laser_Power_step.vi"() -> ("output_laser_Power_step"=w1278:i32)  [unwired: 11 in]
              n627 = call "myRIO_BRig_RT_dataExp_laser_duration.vi"() -> ("output_laser_duration"=w1281:i32)  [unwired: 11 in]
              n628 = call "myRIO_BRig_RT_dataExp_BUR_min.vi"() -> ("output_BUR_min"=w1328:i32)  [unwired: 11 in]
              n629 = call "myRIO_BRig_RT_dataExp_BUR_max.vi"() -> ("output_BUR_max"=w1326:i32)  [unwired: 11 in]
              n630 = call "myRIO_BRig_RT_dataExp_Audio_sp__L.vi"() -> ("output_Audio_sp__L"=w1323:i32)  [unwired: 11 in]
              n631 = call "myRIO_BRig_RT_dataExp_Audio_sp__R.vi"() -> ("output_Audio_sp__R"=w1322:i32)  [unwired: 11 in]
              n632 = local read "laser_Tshutter"() -> (w1293:dbl)
              n633 = local read "f_millisec2count"() -> (w1288:dbl)
              n634 = local read "laser_Tpeak"() -> (w1298:dbl)
              n635 = local read "laser_power_min"() -> (w1283:dbl)
              n636 = local read "laser_power_max"() -> (w1272:dbl)
              n637 = local read "laser_power_step"() -> (w1271:dbl)
              n638 = local read "laser_Freq"() -> (w1305:dbl)
              n639 = local read "sp_LeftSpout"() -> (w1321:u16)
              n640 = local read "BUR_max"() -> (w1325:u16)
              n641 = local read "sp_RightSpout"() -> (w1320:u16)
              n642 = local read "BUR_min"() -> (w1327:u16)
              n643 = Multiply(x=w1305, y=w1273) -> (x*y=w1304:dbl)
              n644 = Multiply(x=w1298, y=w1273) -> (x*y=w1300:dbl)
              n645 = Multiply(x=w1293, y=w1273) -> (x*y=w1295:dbl)
              n646 = Multiply(x=w1288, y=w1273) -> (x*y=w1290:dbl)
              n647 = Multiply(x=w1283, y=w1273) -> (x*y=w1285:dbl)
              n648 = Multiply(x=w1272, y=w1273) -> (x*y=w1277:dbl)
              n649 = Multiply(x=w1271, y=w1273) -> (x*y=w1275:dbl)
              n650 = Round To Nearest(number=w1304) -> (nearest integer value=w1303:dbl)
              n651 = Round To Nearest(number=w1300) -> (nearest integer value=w1299:dbl)
              n652 = Round To Nearest(number=w1295) -> (nearest integer value=w1294:dbl)
              n653 = Round To Nearest(number=w1290) -> (nearest integer value=w1289:dbl)
              n654 = Round To Nearest(number=w1285) -> (nearest integer value=w1284:dbl)
              n655 = Round To Nearest(number=w1277) -> (nearest integer value=w1276:dbl)
              n656 = Round To Nearest(number=w1275) -> (nearest integer value=w1274:dbl)
              n657 = To Unsigned Word Integer(number=w1303) -> (unsigned 16bit integer=w1302:u16)
              n658 = To Unsigned Word Integer(number=w1299) -> (unsigned 16bit integer=w1297:u16)
              n659 = To Unsigned Word Integer(number=w1294) -> (unsigned 16bit integer=w1292:u16)
              n660 = To Unsigned Word Integer(number=w1289) -> (unsigned 16bit integer=w1287:u16)
              n661 = To Unsigned Word Integer(number=w1284) -> (unsigned 16bit integer=w1282:u16)
              n662 = To Unsigned Word Integer(number=w1276) -> (unsigned 16bit integer=w1270:u16)
              n663 = To Unsigned Word Integer(number=w1274) -> (unsigned 16bit integer=w1269:u16)
              n664 = local read "laser_duration"() -> (w1280:u16)
              n665 = call "myRIO_BRig_RT_dataCurrent_LaserPulse_duration.vi"() -> ("output_LaserPulse_duration"=w1307:i32)  [unwired: 11 in]
              n666 = Replace Array Subset(array=w1329, new element #1=w1327, index #1=w1328, new element #2=w1325, index #2=w1326, new element #3=w1321, index #3=w1323, new element #4=w1320, index #4=w1322, new element #5=w1302, index #5=w1306, new element #6=w1297, index #6=w1301, new element #7=w1292, index #7=w1296, new element #8=w1287, index #8=w1291, new element #9=w1282, index #9=w1286, new element #10=w1270, index #10=w1279, new element #11=w1269, index #11=w1278, new element #12=w1280, index #12=w1281) -> (w1324:u16[])
              n667 = Replace Array Subset(array=w1309, new element=w1280, index=w1307) -> (w1308:u16[])
            }
            frame "saveSettings4_LC_ENL" {
              # "delayOpt"
              # "Count"
              # "Tdelay"
              # "Probability"
              # "OnOff"
              # "Block"
              # "ENL1 All"
              # "delayOpt"
              # "Count"
              # "Tdelay"
              # "Probability"
              # "OnOff"
              # "Block"
              # "ENL1 First"
              n668 = call "myRIO_BRig_RT_dataLC_ENL1_All_Block.vi"() -> ("output_ENL1_All_Block"=w1352:i32)  [unwired: 11 in]
              n669 = call "myRIO_BRig_RT_dataLC_ENL1_All_OnOff.vi"() -> ("output_ENL1_All_OnOff"=w1341:i32)  [unwired: 11 in]
              n670 = call "myRIO_BRig_RT_dataLC_ENL1_All_Probability.vi"() -> ("output_ENL1_All_Probability"=w1340:i32)  [unwired: 11 in]
              n671 = call "myRIO_BRig_RT_dataLC_ENL1_All_Tdelay.vi"() -> ("output_ENL1_All_Tdelay"=w1339:i32)  [unwired: 11 in]
              n672 = call "myRIO_BRig_RT_dataLC_ENL1_All_Count.vi"() -> ("output_ENL1_All_Count"=w1338:i32)  [unwired: 11 in]
              n673 = call "myRIO_BRig_RT_dataLC_ENL1_All_delayOpt.vi"() -> ("output_ENL1_All_delayOpt"=w1337:i32)  [unwired: 11 in]
              n674 = call "myRIO_BRig_RT_dataLC_ENL1_First_Block.vi"() -> ("output_ENL1_First_Block"=w1378:i32)  [unwired: 11 in]
              n675 = call "myRIO_BRig_RT_dataLC_ENL1_First_OnOff.vi"() -> ("output_ENL1_First_OnOff"=w1376:i32)  [unwired: 11 in]
              n676 = call "myRIO_BRig_RT_dataLC_ENL1_First_Probability.vi"() -> ("output_ENL1_First_Probability"=w1372:i32)  [unwired: 11 in]
              n677 = call "myRIO_BRig_RT_dataLC_ENL1_First_Tdelay.vi"() -> ("output_ENL1_First_Tdelay"=w1370:i32)  [unwired: 11 in]
              n678 = call "myRIO_BRig_RT_dataLC_ENL1_First_Count.vi"() -> ("output_ENL1_First_Count"=w1368:i32)  [unwired: 11 in]
              n679 = call "myRIO_BRig_RT_dataLC_ENL1_First_delayOpt.vi"() -> ("output_ENL1_First_delayOpt"=w1354:i32)  [unwired: 11 in]
              n680 = local read "LC_ENL1_First_delayOpt"() -> (w1355:bool)
              n681 = local read "LC_ENL1_First_Count"() -> (w1367:u16)
              n682 = local read "LC_ENL1_First_Probability"() -> (w1371:u16)
              n683 = local read "LC_ENL1_First_Block"() -> (w1377:u16)
              n684 = local read "LC_ENL1_First_Tdelay"() -> (w1369:u16)
              n685 = local read "LC_ENL1_First_OnOff"() -> (w1375:bool)
              n686 = local read "LC_ENL1_All_OnOff"() -> (w1348:bool)
              n687 = local read "LC_ENL1_All_Probability"() -> (w1346:u16)
              n688 = local read "LC_ENL1_All_delayOpt"() -> (w1343:bool)
              n689 = local read "LC_ENL1_All_Tdelay"() -> (w1345:u16)
              n690 = local read "LC_ENL1_All_Block"() -> (w1349:u16)
              n691 = local read "LC_ENL1_All_Count"() -> (w1344:u16)
              n692 = Boolean To (0,1)(Boolean=w1355) -> (0, 1=w1356:i16)
              n693 = Boolean To (0,1)(Boolean=w1375) -> (0, 1=w1374:i16)
              n694 = Boolean To (0,1)(Boolean=w1348) -> (0, 1=w1351:i16)
              n695 = To Unsigned Word Integer(number=w1356) -> (unsigned 16bit integer=w1353:u16)
              n696 = To Unsigned Word Integer(number=w1374) -> (unsigned 16bit integer=w1373:u16)
              n697 = Boolean To (0,1)(Boolean=w1343) -> (0, 1=w1350:i16)
              n698 = To Unsigned Word Integer(number=w1351) -> (unsigned 16bit integer=w1347:u16)
              n699 = To Unsigned Word Integer(number=w1350) -> (unsigned 16bit integer=w1342:u16)
              n700 = Replace Array Subset(array=w1379, new element #1=w1377, index #1=w1378, new element #2=w1373, index #2=w1376, new element #3=w1371, index #3=w1372, new element #4=w1369, index #4=w1370, new element #5=w1367, index #5=w1368, new element #6=w1353, index #6=w1354, new element #7=w1349, index #7=w1352, new element #8=w1347, index #8=w1341, new element #9=w1346, index #9=w1340, new element #10=w1345, index #10=w1339, new element #11=w1344, index #11=w1338, new element #12=w1342, index #12=w1337) -> (w1380:u16[])
            }
            frame "saveSettings5_LC_Cue" {
              # "delayOpt"
              # "Count"
              # "Tdelay"
              # "Probability"
              # "OnOff"
              # "Block"
              # "Cue1 All"
              # "delayOpt"
              # "Count"
              # "Tdelay"
              # "Probability"
              # "OnOff"
              # "Block"
              # "Cue1 First"
              n701 = call "myRIO_BRig_RT_dataLC_Cue1_First_delayOpt.vi"() -> ("output_Cue1_First_delayOpt"=w1407:i32)  [unwired: 11 in]
              n702 = call "myRIO_BRig_RT_dataLC_Cue1_First_Block.vi"() -> ("output_Cue1_First_Block"=w1430:i32)  [unwired: 11 in]
              n703 = call "myRIO_BRig_RT_dataLC_Cue1_First_OnOff.vi"() -> ("output_Cue1_First_OnOff"=w1428:i32)  [unwired: 11 in]
              n704 = call "myRIO_BRig_RT_dataLC_Cue1_First_Probability.vi"() -> ("output_Cue1_First_Probability"=w1424:i32)  [unwired: 11 in]
              n705 = call "myRIO_BRig_RT_dataLC_Cue1_First_Tdelay.vi"() -> ("output_Cue1_First_Tdelay"=w1422:i32)  [unwired: 11 in]
              n706 = call "myRIO_BRig_RT_dataLC_Cue1_First_Count.vi"() -> ("output_Cue1_First_Count"=w1420:i32)  [unwired: 11 in]
              n707 = call "myRIO_BRig_RT_dataLC_Cue1_All_Block.vi"() -> ("output_Cue1_All_Block"=w1404:i32)  [unwired: 11 in]
              n708 = call "myRIO_BRig_RT_dataLC_Cue1_All_OnOff.vi"() -> ("output_Cue1_All_OnOff"=w1403:i32)  [unwired: 11 in]
              n709 = call "myRIO_BRig_RT_dataLC_Cue1_All_Probability.vi"() -> ("output_Cue1_All_Probability"=w1402:i32)  [unwired: 11 in]
              n710 = call "myRIO_BRig_RT_dataLC_Cue1_All_Tdelay.vi"() -> ("output_Cue1_All_Tdelay"=w1401:i32)  [unwired: 11 in]
              n711 = call "myRIO_BRig_RT_dataLC_Cue1_All_Count.vi"() -> ("output_Cue1_All_Count"=w1400:i32)  [unwired: 11 in]
              n712 = call "myRIO_BRig_RT_dataLC_Cue1_All_delayOpt.vi"() -> ("output_Cue1_All_delayOpt"=w1399:i32)  [unwired: 11 in]
              n713 = local read "LC_Cue1_First_delayOpt"() -> (w1406:bool)
              n714 = local read "LC_Cue1_First_Count"() -> (w1419:u16)
              n715 = local read "LC_Cue1_First_Probability"() -> (w1423:u16)
              n716 = local read "LC_Cue1_First_Block"() -> (w1429:u16)
              n717 = local read "LC_Cue1_First_Tdelay"() -> (w1421:u16)
              n718 = local read "LC_Cue1_First_OnOff"() -> (w1427:bool)
              n719 = local read "LC_Cue1_All_OnOff"() -> (w1395:bool)
              n720 = local read "LC_Cue1_All_delayOpt"() -> (w1396:bool)
              n721 = local read "LC_Cue1_All_Probability"() -> (w1392:u16)
              n722 = local read "LC_Cue1_All_Tdelay"() -> (w1391:u16)
              n723 = local read "LC_Cue1_All_Count"() -> (w1390:u16)
              n724 = local read "LC_Cue1_All_Block"() -> (w1394:u16)
              n725 = Boolean To (0,1)(Boolean=w1406) -> (0, 1=w1408:i16)
              n726 = Boolean To (0,1)(Boolean=w1427) -> (0, 1=w1426:i16)
              n727 = Boolean To (0,1)(Boolean=w1395) -> (0, 1=w1398:i16)
              n728 = To Unsigned Word Integer(number=w1408) -> (unsigned 16bit integer=w1405:u16)
              n729 = To Unsigned Word Integer(number=w1426) -> (unsigned 16bit integer=w1425:u16)
              n730 = To Unsigned Word Integer(number=w1398) -> (unsigned 16bit integer=w1393:u16)
              n731 = Boolean To (0,1)(Boolean=w1396) -> (0, 1=w1397:i16)
              n732 = To Unsigned Word Integer(number=w1397) -> (unsigned 16bit integer=w1389:u16)
              n733 = Replace Array Subset(array=w1431, new element #1=w1429, index #1=w1430, new element #2=w1425, index #2=w1428, new element #3=w1423, index #3=w1424, new element #4=w1421, index #4=w1422, new element #5=w1419, index #5=w1420, new element #6=w1405, index #6=w1407, new element #7=w1394, index #7=w1404, new element #8=w1393, index #8=w1403, new element #9=w1392, index #9=w1402, new element #10=w1391, index #10=w1401, new element #11=w1390, index #11=w1400, new element #12=w1389, index #12=w1399) -> (w1432:u16[])
            }
            frame "saveSettings6_LC_Other" {
              # "Trial"
              # "Tdelay"
              # "Probability"
              # "OnOff"
              # "Block"
              # "Wrong"
              # "Trial"
              # "Tdelay"
              # "Probability"
              # "OnOff"
              # "Block"
              # "Reward"
              n734 = call "myRIO_BRig_RT_dataLC_Wrong_Block.vi"() -> ("output_Wrong_Block"=w1462:i32)  [unwired: 11 in]
              n735 = call "myRIO_BRig_RT_dataLC_Wrong_OnOff.vi"() -> ("output_Wrong_OnOff"=w1461:i32)  [unwired: 11 in]
              n736 = call "myRIO_BRig_RT_dataLC_Wrong_Probability.vi"() -> ("output_Wrong_Probability"=w1460:i32)  [unwired: 11 in]
              n737 = call "myRIO_BRig_RT_dataLC_Wrong_Tdelay.vi"() -> ("output_Wrong_Tdelay"=w1459:i32)  [unwired: 11 in]
              n738 = call "myRIO_BRig_RT_dataLC_Wrong_Trial.vi"() -> ("output_Wrong_Trial"=w1458:i32)  [unwired: 11 in]
              n739 = call "myRIO_BRig_RT_dataLC_Reward_Block.vi"() -> ("output_Reward_Block"=w1474:i32)  [unwired: 11 in]
              n740 = call "myRIO_BRig_RT_dataLC_Reward_OnOff.vi"() -> ("output_Reward_OnOff"=w1472:i32)  [unwired: 11 in]
              n741 = call "myRIO_BRig_RT_dataLC_Reward_Probability.vi"() -> ("output_Reward_Probability"=w1468:i32)  [unwired: 11 in]
              n742 = call "myRIO_BRig_RT_dataLC_Reward_Tdelay.vi"() -> ("output_Reward_Tdelay"=w1466:i32)  [unwired: 11 in]
              n743 = call "myRIO_BRig_RT_dataLC_Reward_Trial.vi"() -> ("output_Reward_Trial"=w1464:i32)  [unwired: 11 in]
              n744 = local read "LC_Wrong_OnOff"() -> (w1456:bool)
              n745 = local read "LC_Wrong_Probability"() -> (w1453:u16)
              n746 = local read "LC_Wrong_Block"() -> (w1455:u16)
              n747 = local read "LC_Wrong_Tdelay"() -> (w1452:u16)
              n748 = local read "LC_Wrong_Trial"() -> (w1451:u16)
              n749 = local read "LC_Reward_Probability"() -> (w1467:u16)
              n750 = local read "LC_Reward_Block"() -> (w1473:u16)
              n751 = local read "LC_Reward_Tdelay"() -> (w1465:u16)
              n752 = local read "LC_Reward_OnOff"() -> (w1471:bool)
              n753 = local read "LC_Reward_Trial"() -> (w1463:u16)
              n754 = Boolean To (0,1)(Boolean=w1456) -> (0, 1=w1457:i16)
              n755 = Boolean To (0,1)(Boolean=w1471) -> (0, 1=w1470:i16)
              n756 = To Unsigned Word Integer(number=w1457) -> (unsigned 16bit integer=w1454:u16)
              n757 = To Unsigned Word Integer(number=w1470) -> (unsigned 16bit integer=w1469:u16)
              n758 = Replace Array Subset(array=w1475, new element #1=w1473, index #1=w1474, new element #2=w1469, index #2=w1472, new element #3=w1467, index #3=w1468, new element #4=w1465, index #4=w1466, new element #5=w1463, index #5=w1464, new element #6=w1455, index #6=w1462, new element #7=w1454, index #7=w1461, new element #8=w1453, index #8=w1460, new element #9=w1452, index #9=w1459, new element #10=w1451, index #10=w1458) -> (w1476:u16[])
            }
            frame "setSettings_Audio" {
              # "amp_L"
              # "amp_R"
              # "freq_L"
              # "freq_R"
              n759 = call "myRIO_BRig_RT_dataExp_Audio_amp__L.vi"() -> ("output_Audio_amp__L"=w1501:i32)  [unwired: 11 in]
              n760 = call "myRIO_BRig_RT_dataExp_Audio_amp__R.vi"() -> ("output_Audio_amp__R"=w1500:i32)  [unwired: 11 in]
              n761 = call "myRIO_BRig_RT_dataExp_Audio_freq__L.vi"() -> ("output_Audio_freq__L"=w1499:i32)  [unwired: 11 in]
              n762 = call "myRIO_BRig_RT_dataExp_Audio_freq__R.vi"() -> ("output_Audio_freq__R"=w1498:i32)  [unwired: 11 in]
              n763 = Index Array(array=w1497, index #1=w1501, index #2=w1500, index #3=w1499, index #4=w1498) -> (element #1=w1496:u16, element #2=w1495:u16, element #3=w1488:u16, element #4=w1486:u16)
              n764 = To Unsigned Byte Integer(number=w1488) -> (unsigned 8bit integer=w1487:u8)
              n765 = To Unsigned Byte Integer(number=w1486) -> (unsigned 8bit integer=w1485:u8)
            }
            frame "setSettings_Laser" {
              (unwired) u32 0 ("tDelay_laser_rew")
              # "Wrong tDelay"
              # "Reward tDelay"
              n766 = call "myRIO_BRig_RT_dataLC_Reward_Tdelay.vi"() -> ("output_Reward_Tdelay"=w1528:i32)  [unwired: 11 in]
              n767 = call "myRIO_BRig_RT_dataLC_Wrong_Tdelay.vi"() -> ("output_Wrong_Tdelay"=w1529:i32)  [unwired: 11 in]
              n768 = Index Array(array=w1525, index #1=w1528, index #2=w1529) -> (element #1=w1527:u16, element #2=w1526:u16)
              n769 = call "myRIO_BRig_RT__calc_Tvalley.vi"("input_peakWidth"="laser_Tpeak", "input_freq"="laser_Freq") -> ("output_Tvalley"=w1535:dbl)  [unwired: 9 in]
              n770 = To Double Precision Float(number=w1527) -> (double precision float=w1522:dbl)
              n771 = To Double Precision Float(number=w1526) -> (double precision float=w1519:dbl)
              n772 = Multiply(x="f_millisec2count", y="laser_Tpeak") -> (x*y=w1544:dbl)
              n773 = Multiply(x="f_millisec2count", y=w1535) -> (x*y=w1541:dbl)
              n774 = Multiply(x="f_millisec2count", y="laser_Tshutter") -> (x*y=w1539:dbl)
              n775 = Round Toward +Infinity(x="laser_Tshutter") -> (ceil(x): smallest int >= x=w1530:dbl)
              n776 = Multiply(x="f_millisec2count", y=w1522) -> (x*y=w1523:dbl)
              n777 = Multiply(x="f_millisec2count", y=w1519) -> (x*y=w1520:dbl)
              n778 = To Unsigned Word Integer(number="f_millisec2count") -> (unsigned 16bit integer=w1510:u16)
              n779 = Round Toward +Infinity(x=w1544) -> (ceil(x): smallest int >= x=w1545:dbl)
              n780 = Round Toward +Infinity(x=w1541) -> (ceil(x): smallest int >= x=w1542:dbl)
              n781 = Round Toward +Infinity(x=w1539) -> (ceil(x): smallest int >= x=w1534:dbl)
              n782 = Round Toward +Infinity(x=w1523) -> (ceil(x): smallest int >= x=w1524:dbl)
              n783 = Round Toward +Infinity(x=w1520) -> (ceil(x): smallest int >= x=w1521:dbl)
              n784 = To Unsigned Long Integer(number=w1545) -> (unsigned 32bit integer=w1543:u32)
              n785 = To Unsigned Long Integer(number=w1542) -> (unsigned 32bit integer=w1540:u32)
              n786 = To Unsigned Long Integer(number=w1534) -> (unsigned 32bit integer=w1538:u32)
              n787 = To Unsigned Word Integer(number=w1530) -> (unsigned 16bit integer=w1533:u16)
              n788 = To Unsigned Long Integer(number=w1524) -> (unsigned 32bit integer=w1518:u32)
              n789 = To Unsigned Long Integer(number=w1521) -> (unsigned 32bit integer=w1517:u32)
              n790 = Add(x="laser_duration", y=w1533) -> (x+y=w1514:u16)
              n791 = To Double Precision Float(number=w1514) -> (double precision float=w1513:dbl)
              n792 = Multiply(x=w1513, y="f_millisec2count") -> (x*y=w1515:dbl)
              n793 = call "myRIO_BRig_RT_dataCurrent_LaserPulse_duration.vi"() -> ("output_LaserPulse_duration"=w1546:i32)  [unwired: 11 in]
              n794 = Round Toward +Infinity(x=w1515) -> (ceil(x): smallest int >= x=w1516:dbl)
              n795 = To Unsigned Long Integer(number=w1516) -> (unsigned 32bit integer=w1512:u32)
              n796 = xnode "Read/Write Control"("FPGA VI Reference In"=w1548, "error in"=w1549, "laser_Npeak"=w1543, "laser_Nvalley"=w1540, "laser_Nshutter"=w1538, "laser_selRew_Ndelay"=w1518, "laser_selWro_NDelay"=w1517, "laser_selRew_Ntotal"=w1512, "laser_selWro_Ntotal"=w1512, "k1__counter_per_ms"=w1510) -> ("error out"=→"error out":errorcluster)  [unwired: 1 out]
              n797 = Replace Array Subset(array=w1525, new element=w1514, index=w1546) -> (w1547:u16[])
            }
            frame "initBlock" {
              n798 = call "myRIO_Brig_RT__Case_Exp_State_initBlock.vi"("input_spout"=w1592, "input_dataExp"=w1590, "input_dataCurrent"=w1591) -> ("output_spout"=w1569:enum16{"Left", "Right"}, "output_state"=w1593:T2, "output_dataExp"=w1589:u16[], "output_dataCurrent"=w1575:u16[], "output_TpB_target"=→"TpB_target":u16)  [unwired: 4 in]
              "cSpout" <- w1569
              n799 = call "myRIO_BRig_RT_dataCurrent_iBlock.vi"() -> ("output_iBlock"=w1574:i32)  [unwired: 11 in]
              n800 = Index Array(array=w1575, index=w1574) -> (element=→"iBlock":u16)
            }
            frame "initBlock2" {
              n801 = local write "nRewards_cur"(u16 0 ("nRewards_cur")) -> ()
              n802 = call "myRIO_BRig_RT__Case_Exp_State_initBlock2.vi"("input_spout"=w1601, "input_dataBlock"=w1602, "input_dataCurrent"=w1600) -> ("idxDataBlock"=w1597:i32, "output_dataBlock"=w1599:u16[][])  [unwired: 7 in]
            }
            frame "initTrial" {
              n803 = call "myRIO_Brig_RT__Case_Exp_State_initTrial.vi"("input_spout"=w1618, "input_dataExp"=w1635, "input_dataCurrent"=w1636) -> ("output_state"=w1637:T2, "output_dataExp"=w1634:u16[], "output_dataCurrent"=w1624:u16[])  [unwired: 6 in]
              n804 = call "myRIO_BRig_RT_dataCurrent_iTrial.vi"() -> ("output_iTrial"=w1623:i32)  [unwired: 11 in]
              n805 = call "myRIO_BRig_RT_dataCurrent_SolenoidReward.vi"() -> ("output_SolenoidReward"=w1617:i32)  [unwired: 11 in]
              n806 = Index Array(array=w1624, index #1=w1623, index #2=w1617) -> (element #1=→"iTrial":u16, element #2=w1616:u16)
              n807 = Not Equal To 0?(x=w1616) -> (x != 0?=→"SolenoidReward":bool)
            }
            frame "initTrial2" {
              # "trialUntilReward"
              n808 = call "myRIO_BRig_RT__Case_Exp_subState_LC__initTrial.vi"("input_dataTrial"=w1644, "input_spout"=w1653, "input_dataCurrent"=w1642, "input_dataLC"=w1641) -> ("output_LC_Wrong"=w1654:bool, "output_LC_led_Wrong"=w1646:bool, "output_LC_Reward"=w1655:bool, "output_LC_led_Reward"=w1645:bool, "output_dataTrial"=w1643:u16[][])  [unwired: 2 in]
              n809 = Equal?(x=w1653, y=enum16{"Left", "Right"}."Right") -> (x = y?=w1651:bool)
              n810 = call "myRIO_BRig_RT_dataExp_ItrialUntilReward.vi"() -> ("output_I_trialUntilReward"=w1649:i32)  [unwired: 11 in]
              n811 = Index Array(array=w1650, index=w1649) -> (element=w1648:u16)
              n812 = Not Equal To 0?(x=w1648) -> (x != 0?=w1647:bool)
              n813 = xnode "Read/Write Control"("FPGA VI Reference In"=w1668, "error in"=w1667, "SelectionState"=FALSE, "laserResponse_reward"=w1655, "laserResponse_wrong"=w1654, "laserResponse_reward_LED"=w1645, "laserResponse_wrong_LED"=w1646, "Left(F)_or_Right(T)"=w1651, "ignoreWrong"=w1647) -> ("error out"=→"error_initTrial":errorcluster)  [unwired: 1 out]
            }
            frame "initTrial3" {
              n814 = call "myRIO_BRig_RT__Case_Exp_State_initTrial_dataTrial.vi"("input_spout"=w1683, "input_dataCurrent"=w1684, "input_dataExp"=w1682, "input_dataTrial"=w1686) -> ("output_dataTrial"=w1685:u16[][], "output_laserPower"=w1679:u16)  [unwired: 6 in]
              n815 = To Double Precision Float(number=w1679) -> (double precision float=w1681:dbl)
              n816 = Divide(x=w1681, y=100.0 ("x")) -> (x/y=w1674:dbl)
              "output_PortA" <- w1674
              n817 = call "myRIO_Brig_RT__covert_Voltage_to_FPGAvalue.vi"("input_voltage"=w1674) -> ("output_PortA"=w1675:u16)  [unwired: 9 in, 1 out]
              n818 = xnode "Read/Write Control"("FPGA VI Reference In"=w1678, "error in"=w1677, "AnaOut_0"=w1675) -> ("error out"=→"error out 4":errorcluster)  [unwired: 1 out]
            }
            frame "initTrial4" {
              n819 = call "myRIO_BRig_RT_dataCurrent_idxDataTrial.vi"() -> ("output_idxDataTrial"=w1709:i32)  [unwired: 11 in]
              n820 = call "myRIO_BRig_RT_dataTrial_activeRecording.vi"() -> ("output_activeRecording"=w1706:i32)  [unwired: 11 in]
              n821 = Index Array(array=w1711, index=w1709) -> (element=w1708:u16)
              n822 = Boolean To (0,1)(Boolean="Recording") -> (0, 1=w1705:i16)
              n823 = To Long Integer(number=w1708) -> (32bit integer=w1707:i32)
              n824 = To Unsigned Word Integer(number=w1705) -> (unsigned 16bit integer=w1704:u16)
              n825 = Replace Array Subset(array=w1710, new element=w1704, index (row)=w1707, index (col)=w1706) -> (w1703:u16[][])
              n826 = local write "Recording_p2"("Recording") -> ()
            }
            frame "initTrial_LC_ENL1" {
              n827 = call "myRIO_BRig_RT__Case_Exp_State_initTrial_LC_ENL1__v2.vi"("input_dataTrial"=w1735, "input_spout"=w1740, "input_dataBlock"=w1733, "input_dataLC"=w1741, "input_dataCurrent"=w1737) -> ("output_LC__ENL1"=w1739:bool, "output_LC_led__ENL1"=w1738:bool, "output_dataTrial"=w1734:u16[][], "output_dataCurrent"=w1736:u16[])  [unwired: 3 in]
            }
            frame "initTrial_LC_Cue1" {
              n828 = local write "Recording_p2"(FALSE ("Recording_p2")) -> ()
              n829 = call "myRIO_BRig_RT__Case_Exp_State_initTrial_LC_Cue1__v2.vi"("input_dataTrial"=w1763, "input_spout"=w1766, "input_dataBlock"=w1761, "input_dataLC"=w1767, "input_dataCurrent"=w1765) -> ("output_LC__Cue1"=w1759:bool, "output_LC_led__Cue1"=w1760:bool, "output_dataTrial"=w1762:u16[][], "output_dataCurrent"=w1764:u16[])  [unwired: 3 in]
            }
            frame "ENL1_pre" {
              # "ENL1_n"
              # "Tcycle"
              # "counter"
              n830 = call "myRIO_BRig_RT_dataCurrent_Tcycle_generic.vi"() -> ("output_Tcycle_generic"=w1813:i32)  [unwired: 11 in]
              n831 = call "myRIO_BRig_RT_dataCurrent_count_generic.vi"() -> ("output_count_generic"=w1815:i32)  [unwired: 11 in]
              n832 = call "myRIO_BRig_RT_dataCurrent_ENL.vi"() -> ("output_ENL"=w1812:i32)  [unwired: 11 in]
              n833 = call "myRIO_BRig_RT_dataCurrent_ENL1_n.vi"() -> ("output_ENL1_n"=w1784:i32)  [unwired: 11 in]
              n834 = Index Array(array=w1806, index #1=w1812, index #2=w1784) -> (element #1=w1811:u16, element #2=w1783:u16)
              n835 = Increment(x=w1783) -> (x+1=w1782:u16)
              n836 = Replace Array Subset(array=w1806, new element #1=u16 0 ("new element/subarray"), index #1=w1815, new element #2=w1811, index #2=w1813, new element #3=w1782, index #3=w1784) -> (w1810:u16[])
              n837 = Select(t=myRIO_BRig_RT__Case_Exp_stateList."ENL1Penalty_pre" ("Enum"), s=w1794, f=myRIO_BRig_RT__Case_Exp_stateList."ENL1" ("Enum")) -> (s? t:f=w1791:T2)
            }
            frame "ENL1" {
              n838 = call "myRIO_BRig_RT__Case_Exp_State_ENL1__v2.vi"("input_LC"=w1822, "I_lick"=w1826, "input_LC_led"=w1823, "input_laserOccurred"=w1818, "input_state"=w1832, "input_dataCurrent"=w1831) -> ("output_trigger_laser_led"=w1821:bool, "output_state"=w1829:T2, "output_dataCurrent"=w1830:u16[], "output_trigger_laser"=w1820:bool)  [unwired: 2 in]
              n839 = Or(x=w1821, y=w1818) -> (x .or. y?=w1824:bool)
            }
            frame "ENL1Penalty_pre" {
              # "Tcycle"
              # "counter"
              n840 = call "myRIO_BRig_RT_dataCurrent_Tcycle_generic.vi"() -> ("output_Tcycle_generic"=w1872:i32)  [unwired: 11 in]
              n841 = call "myRIO_BRig_RT_dataCurrent_count_generic.vi"() -> ("output_count_generic"=w1874:i32)  [unwired: 11 in]
              n842 = call "myRIO_BRig_RT_dataExp_ENL_penalty.vi"() -> ("output_ENL_penalty"=w1867:i32)  [unwired: 11 in]
              n843 = Index Array(array=w1868, index=w1867) -> (element=w1871:u16)
              n844 = Replace Array Subset(array=w1869, new element #1=u16 0 ("new element/subarray"), index #1=w1874, new element #2=w1871, index #2=w1872) -> (w1870:u16[])
            }
            frame "ENL1Penalty" {
              n845 = call "myRIO_BRig_RT__Case_Exp_State_ENL1Penalty.vi"("input_state"=w1897, "input_dataCurrent"=w1901) -> ("output_state"=w1898:T2, "output_dataCurrent"=w1900:u16[])  [unwired: 8 in]
            }
            frame "ENL2_pre" {
            }
            frame "ENL2" {
            }
            frame "ENL2Penalty_pre" {
            }
            frame "ENL2Penalty" {
            }
            frame "Cue1_pre" {
              # "Cue1_n"
              # "Tcycle_Cue1"
              # "0 = L, 1 = R, 2 = both"
              # "sp_R"
              # "sp_L"
              # "Tcycle"
              # "counter"
              n846 = Equal?(x=w2012, y=enum16{"Left", "Right"}."Left") -> (x = y?=w2011:bool)
              n847 = call "myRIO_BRig_RT_dataExp_Audio_sp__L.vi"() -> ("output_Audio_sp__L"=w2010:i32)  [unwired: 11 in]
              n848 = call "myRIO_BRig_RT_dataExp_Audio_sp__R.vi"() -> ("output_Audio_sp__R"=w2009:i32)  [unwired: 11 in]
              n849 = call "myRIO_BRig_RT_dataCurrent_Tcycle_generic.vi"() -> ("output_Tcycle_generic"=w2022:i32)  [unwired: 11 in]
              n850 = call "myRIO_BRig_RT_dataCurrent_count_generic.vi"() -> ("output_count_generic"=w2024:i32)  [unwired: 11 in]
              n851 = Select(t=w2010, s=w2011, f=w2009) -> (s? t:f=w2008:i32)
              n852 = call "myRIO_BRig_RT_dataCurrent_Cue1_n.vi"() -> ("output_Cue1_n"=w1986:i32)  [unwired: 11 in]
              n853 = call "myRIO_BRig_RT_dataCurrent_Tcycle_cue.vi"() -> ("output_Tcycle_cue"=w1995:i32)  [unwired: 11 in]
              n854 = Index Array(array=w2014, index=w2008) -> (element=w2006:u16)
              n855 = Index Array(array=w1996, index #1=w1995, index #2=w1986) -> (element #1=w1997:u16, element #2=w1988:u16)
              n856 = Increment(x=w1988) -> (x+1=w1987:u16)
              n857 = Not Equal To 0?(x=w2006) -> (x != 0?=w2004:bool)
              n858 = Not Equal?(x=w2006, y=u16 1) -> (x != y?=w2005:bool)
              n859 = Replace Array Subset(array=w1996, new element #1=u16 0 ("new element/subarray"), index #1=w2024, new element #2=w1997, index #2=w2022, new element #3=w1987, index #3=w1986) -> (w2021:u16[])
              n860 = Select(t=myRIO_BRig_RT__Case_Exp_stateList."Cue1Penalty_pre" ("Enum"), s=w1992, f=myRIO_BRig_RT__Case_Exp_stateList."Cue1" ("Enum")) -> (s? t:f=w1993:T2)
            }
            frame "Cue1" {
              n861 = call "myRIO_BRig_RT__Case_Exp_State_Cue1__v2.vi"("input_LC"=w2034, "I_lick"=w2037, "input_LC_led"=w2035, "input_laserOccurred"=w2029, "input_state"=w2039, "input_dataCurrent"=w2057) -> ("output_trigger_laser_led"=w2032:bool, "output_state"=w2038:T2, "output_dataCurrent"=w2056:u16[], "output_trigger_laser"=w2033:bool)  [unwired: 2 in]
              n862 = Or(x=w2032, y=w2029) -> (x .or. y?=w2031:bool)
              n863 = Equal?(x=myRIO_BRig_RT__Case_Exp_stateList."Selection_pre", y=w2038) -> (x = y?=w2042:bool)
              n864 = xnode "Read/Write Control"("FPGA VI Reference In"=w2041, "error in"=w2040, "SelectionState"=w2042) -> ()  [unwired: 2 out]
            }
            frame "Cue1Penalty_pre" {
              # "Tcycle"
              # "counter"
              n865 = call "myRIO_BRig_RT_dataCurrent_Tcycle_generic.vi"() -> ("output_Tcycle_generic"=w2088:i32)  [unwired: 11 in]
              n866 = call "myRIO_BRig_RT_dataCurrent_count_generic.vi"() -> ("output_count_generic"=w2090:i32)  [unwired: 11 in]
              n867 = call "myRIO_BRig_RT_dataExp_Tcycle_CuePenalty.vi"() -> ("output_Tcycle_CuePenalty"=w2087:i32)  [unwired: 11 in]
              n868 = Index Array(array=w2082, index=w2087) -> (element=w2086:u16)
              n869 = Replace Array Subset(array=w2084, new element #1=u16 0 ("new element/subarray"), index #1=w2090, new element #2=w2086, index #2=w2088) -> (w2083:u16[])
            }
            frame "Cue1Penalty" {
              # "reset laserOccurred"
              n870 = call "myRIO_BRig_RT__Case_Exp_State_Cue1Penalty.vi"("input_state"=w2114, "input_dataCurrent"=w2115) -> ("output_state"=w2112:T2, "output_dataCurrent"=w2113:u16[])  [unwired: 8 in]
            }
            frame "Cue2_pre" {
              n871 = call "myRIO_BRig_RT__Case_Exp_subState_LC__Cue2.vi"("input_spout"=w2132, "input_dataCurrent"=w2133, "input_dataLC"=w2131) -> ()  [unwired: 6 in, 2 out]
            }
            frame "Cue2" {
            }
            frame "Cue2Penalty_pre" {
            }
            frame "Cue2Penalty" {
            }
            frame "Selection_pre" {
              # "Tcycle"
              # "counter"
              n872 = xnode "Read/Write Control"("FPGA VI Reference In"=w2204, "error in"=w2205) -> ("error out"=→"error_Selection_pre":errorcluster, "SelectReward"=w2197:bool, "SelectWrong"=w2199:bool)  [unwired: 1 out]
              n873 = call "myRIO_BRig_RT_dataCurrent_Tcycle_generic.vi"() -> ("output_Tcycle_generic"=w2226:i32)  [unwired: 11 in]
              n874 = call "myRIO_BRig_RT_dataCurrent_count_generic.vi"() -> ("output_count_generic"=w2228:i32)  [unwired: 11 in]
              n875 = call "myRIO_BRig_RT_dataExp_Tcycle_Selection.vi"() -> ("output_Tcycle_Selection"=w2225:i32)  [unwired: 11 in]
              n876 = Index Array(array=w2222, index=w2225) -> (element=w2224:u16)
              n877 = Replace Array Subset(array=w2220, new element #1=u16 0 ("new element/subarray"), index #1=w2228, new element #2=w2224, index #2=w2226) -> (w2223:u16[])
              n878 = Or(x=w2197, y=w2199) -> (x .or. y?=w2198:bool)
              n879 = Select(t=myRIO_BRig_RT__Case_Exp_stateList."SelectReward_pre" ("Enum"), s=w2197, f=myRIO_BRig_RT__Case_Exp_stateList."SelectWrong_pre" ("Enum")) -> (s? t:f=w2203:T2)
              n880 = Select(t=w2203, s=w2198, f=myRIO_BRig_RT__Case_Exp_stateList."Selection" ("Enum")) -> (s? t:f=w2200:T2)
            }
            frame "Selection" {
              # "counter\nSelection"
              # "increment"
              # "get Tcycle"
              # "get count"
              n881 = xnode "Read/Write Control"("FPGA VI Reference In"=w2253, "error in"=w2252) -> ("error out"=→"error_Selection":errorcluster, "SelectReward"=w2249:bool, "SelectWrong"=w2250:bool)  [unwired: 1 out]
              n882 = call "myRIO_BRig_RT_dataCurrent_Tcycle_generic.vi"() -> ("output_Tcycle_generic"=w2246:i32)  [unwired: 11 in]
              n883 = call "myRIO_BRig_RT_dataCurrent_count_generic.vi"() -> ("output_count_generic"=w2239:i32)  [unwired: 11 in]
              n884 = Index Array(array=w2247, index #1=w2246, index #2=w2239) -> (element #1=w2238:u16, element #2=w2245:u16)
              n885 = call "myRIO_BRig_RT__increment_u16.vi"() -> ("output_increment__u16"=w2244:u16)  [unwired: 11 in]
              n886 = Add(x=w2245, y=w2244) -> (x+y=w2240:u16)
              n887 = Greater?(x=w2238, y=w2240) -> (0:w2232:bool)
              n888 = Select(t=w2243, s=w2232, f=myRIO_BRig_RT__Case_Exp_stateList."SelectTimeout_pre" ("Enum")) -> (s? t:f=w2233:T2)
              n889 = Select(t=w2240, s=w2232, f=w2238) -> (s? t:f=w2236:u16)
              n890 = call "myRIO_BRig_RT_dataCurrent_count_selection.vi"() -> ("output_count_generic"=w2237:i32)  [unwired: 11 in]
              n891 = Select(t=myRIO_BRig_RT__Case_Exp_stateList."SelectReward_pre" ("Enum"), s=w2249, f=myRIO_BRig_RT__Case_Exp_stateList."SelectWrong_pre" ("Enum")) -> (s? t:f=w2248:T2)
              n892 = Replace Array Subset(array=w2247, new element #1=w2236, index #1=w2239, new element #2=w2236, index #2=w2237) -> (w2242:u16[])
              n893 = Or(x=w2249, y=w2250) -> (x .or. y?=w2231:bool)
              n894 = Select(t=w2248, s=w2231, f=w2233) -> (s? t:f=w2251:T2)
            }
            frame "SelectReward_pre" {
              # "iState"
              # "Tcycle\nReward"
              # "nRewTrials"
              # "Tcycle\nGeneric"
              # "counter"
              n895 = call "myRIO_BRig_RT_dataCurrent_nRewTrials.vi"() -> ("output_nRewTrials"=w2285:i32)  [unwired: 11 in]
              n896 = Equal?(x=w2294, y=enum16{"Left", "Right"}."Left") -> (x = y?=w2295:bool)
              n897 = Index Array(array=w2286, index=w2285) -> (element=w2284:u16)
              n898 = call "myRIO_BRig_RT_dataExp_Tcycle_Reward__L.vi"() -> ("output_Tcycle_Reward__L"=w2298:i32)  [unwired: 11 in]
              n899 = call "myRIO_BRig_RT_dataExp_Tcycle_Reward__R.vi"() -> ("output_Tcycle_Reward__R"=w2299:i32)  [unwired: 11 in]
              n900 = Increment(x=w2284) -> (x+1=w2283:u16)
              n901 = Select(t=w2298, s=w2295, f=w2299) -> (s? t:f=w2297:i32)
              n902 = call "myRIO_BRig_RT__Case_Exp_subState_LC__Reward.vi"("input_spout"=w2294, "input_dataCurrent"=w2286, "input_dataLC"=w2293) -> ()  [unwired: 6 in, 2 out]
              n903 = call "myRIO_BRig_RT_dataCurrent_count_generic.vi"() -> ("output_count_generic"=w2288:i32)  [unwired: 11 in]
              n904 = call "myRIO_BRig_RT_dataCurrent_Tcycle_generic.vi"() -> ("output_Tcycle_generic"=w2289:i32)  [unwired: 11 in]
              n905 = Index Array(array=w2300, index=w2297) -> (element=w2290:u16)
              n906 = call "myRIO_BRig_RT_dataCurrent_iState.vi"() -> ("output_iState"=w2278:i32)  [unwired: 11 in]
              n907 = Replace Array Subset(array=w2286, new element #1=w2283, index #1=w2285, new element #2=u16 0 ("new element/subarray"), index #2=w2288, new element #3=w2290, index #3=w2289, new element #4=u16 1 ("new element/subarray"), index #4=w2278) -> (w2301:u16[])
            }
            frame "SelectReward" {
              n908 = call "myRIO_BRig_RT__Case_Exp_State_Reward.vi"("input_dataCurrent"=w2322, "input_state"=w2319, "input_spout"=w2317) -> ("output_dataCurrent"=w2321:u16[], "output_state"=w2320:T2, "output__L"=w2315:bool, "output__R"=w2316:bool)  [unwired: 9 in]
            }
            frame "SelectRewardPost_pre" {
              # "nRewards"
              # "nRewTrials"
              # "Tcycle"
              # "counter"
              n909 = call "myRIO_BRig_RT_dataBlock_nRewards__L.vi"() -> ("output_nRewards__L"=w2338:i32)  [unwired: 11 in]
              n910 = call "myRIO_BRig_RT_dataBlock_nRewards__R.vi"() -> ("output_nRewards__R"=w2337:i32)  [unwired: 11 in]
              n911 = call "myRIO_BRig_RT_dataCurrent_Tcycle_generic.vi"() -> ("output_Tcycle_generic"=w2357:i32)  [unwired: 11 in]
              n912 = call "myRIO_BRig_RT_dataCurrent_count_generic.vi"() -> ("output_count_generic"=w2359:i32)  [unwired: 11 in]
              n913 = case shown="\"Left\", Default" w2331 {
                tunnel: w2343 -> [w2364 w2368]
                tunnel: [w2363 w2368] -> w2342
                tunnel: [w2365 w2366] -> w2341
                tunnel: w2340 -> [w2365 w2367]
                frame "Left", Default {
                  n914 = Increment(x=w2364) -> (x+1=w2363:u16)
                }
                frame "Right" {
                  n915 = Increment(x=w2367) -> (x+1=w2366:u16)
                }
              }
              "nRewards_Left" <- w2342
              "nRewards_Right" <- w2341
              n916 = Equal?(x=w2331, y=enum16{"Left", "Right"}."Left") -> (x = y?=w2330:bool)
              n917 = Select(t=w2338, s=w2330, f=w2337) -> (s? t:f=w2336:i32)
              n918 = call "myRIO_BRig_RT_dataExp_Tcycle_RewardPost.vi"() -> ("output_Tcycle_RewardPost"=w2353:i32)  [unwired: 11 in]
              n919 = call "myRIO_BRig_RT_dataCurrent_nRewTrials.vi"() -> ("output_nRewTrials"=w2339:i32)  [unwired: 11 in]
              n920 = Index Array(array=w2354, index=w2353) -> (element=w2356:u16)
              n921 = Index Array(array=w2333, index=w2339) -> (element=w2328:u16)
              n922 = Replace Array Subset(array=w2333, new element #1=u16 0 ("new element/subarray"), index #1=w2359, new element #2=w2356, index #2=w2357) -> (w2355:u16[])
              n923 = Replace Array Subset(array=w2335, new element=w2328, index (row)=w2329, index (col)=w2336) -> (w2334:u16[][])
              n924 = local write "nRewards_cur"(w2328) -> ()
            }
            frame "SelectRewardPost" {
              n925 = call "myRIO_BRig_RT__Case_Exp_State_RewardPost.vi"("input_state"=w2383, "input_dataCurrent"=w2386) -> ("output_state"=w2384:T2, "output_dataCurrent"=w2385:u16[])  [unwired: 8 in]
            }
            frame "SelectWrong_pre" {
              # "iState"
              # "Tcycle"
              # "counter"
              n926 = call "myRIO_BRig_RT_dataCurrent_Tcycle_generic.vi"() -> ("output_Tcycle_generic"=w2411:i32)  [unwired: 11 in]
              n927 = call "myRIO_BRig_RT_dataCurrent_count_generic.vi"() -> ("output_count_generic"=w2413:i32)  [unwired: 11 in]
              n928 = call "myRIO_BRig_RT_dataExp_Tcycle_Wrong.vi"() -> ("output_Tcycle_Wrong"=w2409:i32)  [unwired: 11 in]
              n929 = call "myRIO_BRig_RT__Case_Exp_subState_LC__Wrong.vi"("input_spout"=w2405, "input_dataCurrent"=w2406, "input_dataLC"=w2403) -> ()  [unwired: 6 in, 2 out]
              n930 = Index Array(array=w2407, index=w2409) -> (element=w2410:u16)
              n931 = call "myRIO_BRig_RT_dataCurrent_iState.vi"() -> ("output_iState"=w2397:i32)  [unwired: 11 in]
              n932 = Replace Array Subset(array=w2406, new element #1=u16 0 ("new element/subarray"), index #1=w2413, new element #2=w2410, index #2=w2411, new element #3=u16 2 ("new element/subarray"), index #3=w2397) -> (w2408:u16[])
            }
            frame "SelectWrong" {
              n933 = call "myRIO_BRig_RT__Case_Exp_State_Wrong.vi"("input_state"=w2427, "input_dataCurrent"=w2436) -> ("output_state"=w2424:T2, "output_dataCurrent"=w2435:u16[])  [unwired: 8 in]
              n934 = Not Equal?(x=w2427, y=w2424) -> (x != y?=w2426:bool)
              n935 = Select(t=myRIO_BRig_RT__Case_Exp_stateList."SelectWrong_post" ("Enum"), s=w2426, f=w2424) -> (s? t:f=w2423:T2)
            }
            frame "SelectWrong_post" {
            }
            frame "SelectTimeout_pre" {
              # "iState"
              # "Tcycle"
              # "counter"
              n936 = xnode "Read/Write Control"("FPGA VI Reference In"=w2463, "error in"=w2462, "SelectionState"=FALSE) -> ("error out"=→"error out 3":errorcluster)  [unwired: 1 out]
              n937 = call "myRIO_BRig_RT_dataCurrent_Tcycle_generic.vi"() -> ("output_Tcycle_generic"=w2485:i32)  [unwired: 11 in]
              n938 = call "myRIO_BRig_RT_dataCurrent_count_generic.vi"() -> ("output_count_generic"=w2483:i32)  [unwired: 11 in]
              n939 = call "myRIO_BRig_RT_dataExp_Tcycle_Timeout.vi"() -> ("output_Tcycle_Timeout"=w2487:i32)  [unwired: 11 in]
              n940 = call "myRIO_BRig_RT__Case_Exp_subState_LC__Timeout.vi"("input_spout"=w2478, "input_dataCurrent"=w2479, "input_dataLC"=w2477) -> ()  [unwired: 6 in, 2 out]
              n941 = Index Array(array=w2481, index=w2487) -> (element=w2486:u16)
              n942 = call "myRIO_BRig_RT_dataCurrent_iState.vi"() -> ("output_iState"=w2471:i32)  [unwired: 11 in]
              n943 = Replace Array Subset(array=w2479, new element #1=u16 0 ("new element/subarray"), index #1=w2483, new element #2=w2486, index #2=w2485, new element #3=u16 3 ("new element/subarray"), index #3=w2471) -> (w2482:u16[])
            }
            frame "SelectTimeout" {
              n944 = call "myRIO_BRig_RT__Case_Exp_State_Timeout.vi"("input_dataLC"=w2506, "input_LC"=w2507, "input_state"=w2497, "input_dataCurrent"=w2512) -> ("output_state"=w2498:T2, "output_dataCurrent"=w2511:u16[])  [unwired: 5 in, 1 out]
              n945 = Not Equal?(x=w2497, y=w2498) -> (x != y?=w2501:bool)
              n946 = Select(t=myRIO_BRig_RT__Case_Exp_stateList."SelectTimeout_post" ("Enum"), s=w2501, f=w2498) -> (s? t:f=w2499:T2)
            }
            frame "SelectTimeout_post" {
            }
            frame "endTrial1" {
              # "Update dataBlock"
              n947 = call "myRIO_BRig_RT__Case_Exp_State_endTrial1.vi"("input_spout"=w2545, "input_dataBlock"=w2544, "input_dataCurrent"=w2542) -> ("output_dataBlock"=w2543:u16[][], "output_dataCurrent"=w2541:u16[])  [unwired: 7 in]
            }
            frame "endTrial2" {
              # "update dataTrial"
              n948 = call "myRIO_BRig_RT__Case_Exp_State_endTrial2.vi"("input_spout"=w2564, "input_dataTrial"=w2568, "input_dataCurrent"=w2566) -> ("output_dataTrial"=w2567:u16[][], "output_dataCurrent"=w2565:u16[])  [unwired: 7 in]
            }
            frame "endTrial3" {
              w2594 = myRIO_BRig_RT__Case_Exp_stateList."endBlock" ("Enum")
              # "nRewTrials"
              # "iTrial"
              # "I_blockUntilReward"
              # "TPB"
              # "end block?"
              n949 = local read "STOP_endTrial"() -> (w2592:bool)
              n950 = local read "STOP_abort"() -> (w2591:bool)
              n951 = xnode "Read/Write Control"("FPGA VI Reference In"=w2580, "error in"=w2579, "SelectionState"=FALSE) -> ("error out"=→"error out 2":errorcluster)  [unwired: 1 out]
              n952 = local read "START"() -> (w2589:bool)
              n953 = call "myRIO_BRig_RT_dataExp_IblockUntilReward.vi"() -> ("output_I_blockUntilReward"=w2601:i32)  [unwired: 11 in]
              n954 = Index Array(array=w2585, index=w2601) -> (element=w2581:u16)
              n955 = Not(x=w2589) -> (.not. x?=w2590:bool)
              n956 = Not Equal To 0?(x=w2581) -> (x != 0?=w2599:bool)
              n957 = Compound Arithmetic op=OR(w2592, w2590, w2591) -> (w2593:bool)
              n958 = call "myRIO_BRig_RT_dataCurrent_nRewTrials.vi"() -> ("output_nRewTrials"=w2597:i32)  [unwired: 11 in]
              n959 = call "myRIO_BRig_RT_dataCurrent_iTrial.vi"() -> ("output_iTrial"=w2598:i32)  [unwired: 11 in]
              n960 = Select(t=w2597, s=w2599, f=w2598) -> (s? t:f=w2596:i32)
              n961 = call "myRIO_BRig_RT_dataCurrent_TpB.vi"() -> ("output_TpB"=w2600:i32)  [unwired: 11 in]
              n962 = Index Array(array=w2586, index #1=w2600, index #2=w2596) -> (element #1=w2587:u16, element #2=w2588:u16)
              n963 = Less Or Equal?(x=w2587, y=w2588) -> (x <= y?=w2584:bool)
              n964 = Select(t=w2594, s=w2584, f=myRIO_BRig_RT__Case_Exp_stateList."empty_endTrial1" ("Enum")) -> (s? t:f=w2595:T2)
              n965 = Select(t=w2594, s=w2593, f=w2595) -> (s? t:f=w2582:T2)
            }
            frame "endBlock" {
              # "R"
              # "L"
              # "idxDataBlock"
              n966 = Equal?(x=w2625, y=enum16{"Left", "Right"}."Left") -> (x = y?=w2624:bool)
              n967 = call "myRIO_BRig_RT_dataCurrent_idxDataBlockL.vi"() -> ("output_idxDataBlock__L"=w2628:i32)  [unwired: 11 in]
              n968 = call "myRIO_BRig_RT_dataCurrent_idxDataBlockR.vi"() -> ("output_idxDataBlock__R"=w2627:i32)  [unwired: 11 in]
              n969 = Increment(x=w2619) -> (x+1=w2618:i32)
              n970 = Select(t=w2628, s=w2624, f=w2627) -> (s? t:f=w2622:i32)
              n971 = To Unsigned Word Integer(number=w2618) -> (unsigned 16bit integer=w2620:u16)
              n972 = local read "START"() -> (w2648:bool)
              n973 = local read "STOP_endBlock"() -> (w2643:bool)
              n974 = local read "STOP_endTrial"() -> (w2646:bool)
              n975 = local read "STOP_abort"() -> (w2645:bool)
              n976 = Replace Array Subset(array=w2623, new element=w2620, index=w2622) -> (w2621:u16[])
              n977 = Not(x=w2648) -> (.not. x?=w2647:bool)
              n978 = Compound Arithmetic op=OR(w2647, w2643, w2646, w2645) -> (w2644:bool)
              n979 = Select(t=myRIO_BRig_RT__Case_Exp_stateList."endExp" ("Enum"), s=w2644, f=myRIO_BRig_RT__Case_Exp_stateList."empty_endBlock1" ("Enum")) -> (s? t:f=w2652:T2)
            }
            frame "endExp" {
            }
            frame "commConnect" {
              n980 = call "myRIO_BRig_RT_comm_webdav_connect.vi"("input_password"="Host Password", "input_username"="Host UserName") -> ("output_Iconnected"=w2673:bool, "output_hSession"=w2691:T6)  [unwired: 7 in, 1 out]
              "Connected To Host?" <- w2673
              n981 = case shown="False" w2673 {
                frame False {
                  n982 = One Button Dialog(message="Connection Failed!\nData not being saved!") -> ()  [unwired: 1 in, 1 out]
                }
                frame True {
                }
              }
            }
            frame "commUpload_pre" {
              n983 = Select(t=myRIO_BRig_RT__Case_Exp_stateList."commUpload_dataBlock" ("Enum"), s=w2698, f=myRIO_BRig_RT__Case_Exp_stateList."endTrial3") -> (s? t:f=w2696:T2)
            }
            frame "commUpload_dataBlock" {
              n984 = call "myRIO_BRig_RT_comm_webdav_uploadFile__data.vi"("input_fileName_prefix"=w2719, "input_fileName"="dataBlock" ("input_filename"), "input_hSession"=w2721) -> ()  [unwired: 8 in, 1 out]
            }
            frame "commUpload_dataCurrent" {
              n985 = call "myRIO_BRig_RT_comm_webdav_uploadFile__data.vi"("input_fileName_prefix"=w2740, "input_fileName"="dataCurrent" ("input_filename"), "input_hSession"=w2742) -> ()  [unwired: 8 in, 1 out]
            }
            frame "commUpload_dataExp" {
              n986 = call "myRIO_BRig_RT_comm_webdav_uploadFile__data.vi"("input_fileName_prefix"=w2761, "input_fileName"="dataExp" ("input_filename"), "input_hSession"=w2763) -> ()  [unwired: 8 in, 1 out]
            }
            frame "commUpload_dataLC" {
              n987 = call "myRIO_BRig_RT_comm_webdav_uploadFile__data.vi"("input_fileName_prefix"=w2782, "input_fileName"="dataLC" ("input_filename"), "input_hSession"=w2784) -> ()  [unwired: 8 in, 1 out]
            }
            frame "commUpload_dataTrial" {
              n988 = call "myRIO_BRig_RT_comm_webdav_uploadFile__data.vi"("input_fileName_prefix"=w2806, "input_fileName"="dataTrial" ("input_filename"), "input_hSession"=w2808) -> ()  [unwired: 8 in, 1 out]
            }
            frame "saveData_dataBlock" {
              # "idxDataBlockR"
              # "idxDataBlockL"
              n989 = call "myRIO_BRig_RT_dataCurrent_idxDataBlockL.vi"() -> ("output_idxDataBlock__L"=w2832:i32)  [unwired: 11 in]
              n990 = call "myRIO_BRig_RT_dataCurrent_idxDataBlockR.vi"() -> ("output_idxDataBlock__R"=w2833:i32)  [unwired: 11 in]
              n991 = Index Array(array=w2834, index #1=w2832, index #2=w2833) -> (element #1=w2831:u16, element #2=w2830:u16)
              n992 = Greater?(x=w2831, y=w2830) -> (0:w2829:bool)
              n993 = Select(t=w2831, s=w2829, f=w2830) -> (s? t:f=w2827:u16)
              n994 = Increment(x=w2827) -> (x+1=w2826:u16)
              n995 = To Long Integer(number=w2826) -> (32bit integer=w2825:i32)
              n996 = Array Subset(array=w2828, length (row)=w2825) -> (w2824:u16[][])  [unwired: 3 in]
              n997 = call "myRIO_BRig_RT_comm_webdav_saveArrayToFile__2D_u16.vi"("Array"=w2824, "input_filename"="dataBlock") -> ()  [unwired: 10 in]
            }
            frame "saveData_dataCurrent" {
              n998 = call "myRIO_BRig_RT_comm_webdav_saveArrayToFile__1D_u16.vi"("Array"=w2853, "input_filename"="dataCurrent") -> ()  [unwired: 10 in]
            }
            frame "saveData_dataExp" {
              # "runTime"
              n999 = Get Date/Time In Seconds() -> (seconds since 1Jan1904=w2881:timestamp)
              n1000 = To Double Precision Float(number=w2881) -> (double precision float=w2880:dbl)
              n1001 = call "myRIO_BRig_RT_dataExp_runTime_seconds.vi"() -> ("output_RunTime_minutes"=w2879:i32)  [unwired: 11 in]
              n1002 = Subtract(x=w2880, y=w2878) -> (x-y=w2875:dbl)
              n1003 = To Unsigned Word Integer(number=w2875) -> (unsigned 16bit integer=w2874:u16)
              n1004 = Replace Array Subset(array=w2873, new element=w2874, index=w2879) -> (w2876:u16[])
              n1005 = call "myRIO_BRig_RT_comm_webdav_saveArrayToFile__1D_u16.vi"("Array"=w2876, "input_filename"="dataExp") -> ()  [unwired: 10 in]
            }
            frame "saveData_dataLC" {
              n1006 = call "myRIO_BRig_RT_comm_webdav_saveArrayToFile__1D_u16.vi"("Array"=w2900, "input_filename"="dataLC") -> ()  [unwired: 10 in]
            }
            frame "saveData_dataTrial" {
              # "idxTrial"
              n1007 = call "myRIO_BRig_RT_dataCurrent_idxDataTrial.vi"() -> ("output_idxDataTrial"=w2925:i32)  [unwired: 11 in]
              n1008 = Index Array(array=w2926, index=w2925) -> (element=w2922:u16)
              n1009 = Increment(x=w2922) -> (x+1=w2921:u16)
              n1010 = To Long Integer(number=w2921) -> (32bit integer=w2920:i32)
              n1011 = Array Subset(array=w2923, length (row)=w2920) -> (w2924:u16[][])  [unwired: 3 in]
              n1012 = call "myRIO_BRig_RT_comm_webdav_saveArrayToFile__2D_u16.vi"("Array"=w2924, "input_filename"="dataTrial") -> ()  [unwired: 10 in]
            }
            frame "empty_endBlock1" {
            }
            frame "empty_endBlock2" {
            }
            frame "empty_endTrial1" {
            }
            frame "empty_endTrial2" {
            }
            frame "empty_endTrial3" {
            }
            frame "empty_endTrial4" {
            }
            frame "empty_endTrial5" {
            }
          }
          n1013 = case shown="True" w1074 {
            tunnel: w1070 -> [w1097 w1105]
            tunnel: w1073 -> [_ w1101]
            tunnel: w1072 -> [_ w1100]
            tunnel: w1071 -> [_ w1099]
            tunnel: w1040 -> [_ w1098]
            tunnel: [w1097 w1104] -> w1069
            tunnel: w1068 -> [w1096 w1103]
            tunnel: [w1096 w1102] -> w1067
            frame False {
            }
            frame True {
              n1014 = call "myRIO_BRig_RT__Case_Exp__recordLick.vi"("intput_state__trialEnd"=w1098, "intput_state__trialStart"=w1099, "input_lick__R"=w1100, "input_lick__L"=w1101, "input_dataCurrent"=w1103, "input_dataLick"=w1105) -> ("output_dataCurrent"=w1102:u16[], "output_dataLick"=w1104:u16[][])  [unwired: 4 in]
            }
          }
          n1015 = Or(x=w1042, y=w1043) -> (x .or. y?=w1029:bool)
          n1016 = Or(x=w1046, y=w1026) -> (x .or. y?=w1015:bool)
          n1017 = Or(x=w1025, y=w1047) -> (x .or. y?=w1041:bool)
          n1018 = Or(x=w1045, y=w1044) -> (x .or. y?=w1030:bool)
          n1019 = Or(x=w1075, y="STOP_abort") -> (x .or. y?=w1077:bool)
          n1020 = Or(x=w1004, y=w1005) -> (x .or. y?=w1002:bool)
          n1021 = Or(x=w1006, y=w1005) -> (x .or. y?=w1003:bool)
          n1022 = xnode "Read/Write Control"("FPGA VI Reference In"=w1017, "error in"=w1016, "A1_SR"=w1030, "A3_SL"=w1029, "A6_Act"="Recording_p2", "audioTrigger_L"=w1015, "audioAmp_L"=w1056, "audioFreq_L_kHz"=w1024, "audioTrigger_R"=w1041, "audioAmp_R"=w1057, "audioFreq_R_kHz"=w1058, "laserledMTrig"=w1002, "laserMTrig"=w1003) -> ("FPGA VI Reference Out"=w1066:refnum<k20>, "error out"=w1065:errorcluster)
          n1023 = node-c288() -> ()  [unwired: 1 in, 1 out]
          "cState" <- w1071
        }
        n1024 = node-c288(w960) -> ()  [unwired: 1 out]
        n1025 = flat-sequence {
          tunnel: w956 -> [w994]
          tunnel: w955 -> [w993]
          tunnel: [w992] -> w948
          tunnel: [w991] -> w947
          tunnel: [w997] -> w949
          tunnel: [w998] -> w954
          tunnel: w948 -> [w998]
          tunnel: w947 -> [w997]
          frame #0 {
            w988 = u8 0
            w989 = u16 0 ("AudioLeft_phase_inc")
            w990 = FALSE
            n1026 = xnode "Read/Write Control"("FPGA VI Reference In"=w994, "error in"=w993, "Counts_Reset"=TRUE, "audioTrigger_L"=w990, "audioFreq_L_kHz"=w988, "audioAmp_L"=w989, "audioTrigger_R"=w990, "audioFreq_R_kHz"=w988, "audioAmp_R"=w989, "A3_SL"=w990, "A1_SR"=w990, "A6_Act"=w990) -> ("FPGA VI Reference Out"=w992:refnum<k20>, "error out"=w991:errorcluster)
          }
          frame #1 {
            w996 = FALSE ("START")
            n1027 = local write "START"(w996) -> ()
            n1028 = local write "STOP_endTrial"(w996) -> ()
            n1029 = local write "STOP_endBlock"(w996) -> ()
          }
        }
        n1030 = stacked-sequence {
          tunnel: w932 -> [w968 _]
          tunnel: w930 -> [w969 _]
          tunnel: w929 -> [_ w974]
          tunnel: w928 -> [_ w973]
          tunnel: w927 -> [_ w972]
          tunnel: w926 -> [w962 _]
          frame #0 {
            n1031 = call "myRIO_BRig_RT_dataCurrent_idxDataLick.vi"() -> ("output_idxDataLick"=w963:i32)  [unwired: 11 in]
            n1032 = Index Array(array=w962, index=w963) -> (element=w965:u16)
            n1033 = Increment(x=w965) -> (x+1=w966:u16)
            n1034 = call "myRIO_BRig_RT_comm_webdav_saveArrayToFile__1D_u16.vi"("Array"=w969, "input_filename"="dataMTrig") -> ()  [unwired: 10 in]
            n1035 = To Long Integer(number=w966) -> (32bit integer=w964:i32)
            n1036 = Array Subset(array=w968, length (row)=w964) -> (w967:u16[][])  [unwired: 3 in]
            n1037 = call "myRIO_BRig_RT_comm_webdav_saveArrayToFile__2D_u16.vi"("Array"=w967, "input_filename"="dataLick") -> ()  [unwired: 10 in]
          }
          frame #1 {
            n1038 = case shown="True" w974 {
              tunnel: w973 -> [_ w976]
              tunnel: w972 -> [_ w975]
              frame False {
              }
              frame True {
                n1039 = stacked-sequence {
                  tunnel: w976 -> [w978 w985 w987]
                  tunnel: w975 -> [w979 w984 _]
                  frame #0 {
                    n1040 = call "myRIO_BRig_RT_comm_webdav_uploadFile__announce.vi"("input_addText"=TRUE, "input_fileName_prefix"=w979, "intput_fileName"="curExp_end", "intput_hSession"=w978) -> ("output_Isuccess"=w977:bool)  [unwired: 6 in, 1 out]
                    n1041 = case shown="True" w977 {
                      frame False {
                        n1042 = One Button Dialog(message="!!! Warning !!! Your data is located at C:\\BehaviorRig\\commTransfer") -> ()  [unwired: 1 in, 1 out]
                      }
                      frame True {
                        n1043 = Wait (ms)(milliseconds to wait=u32 20) -> ()  [unwired: 1 out]
                      }
                    }
                  }
                  frame #1 {
                    n1044 = call "myRIO_BRig_RT__endExp_sendData.vi"("input_fileName_prefix"=w984, "input_hSession"=w985) -> ()  [unwired: 8 in, 2 out]
                  }
                  frame #2 {
                    n1045 = local write "Connected To Host?"(FALSE ("Connected To Host?")) -> ()
                    n1046 = call <vilib>:"Close Session.vi"("session handle"=w987) -> ()  [unwired: 14 in, 1 out]
                  }
                }
              }
            }
          }
        }
      }
    }
    n1047 = local read "STOP_abort"() -> (w30:bool)
  }
  n1048 = xnode "Read/Write Control"("FPGA VI Reference In"=w8, "error in"=w7, "FPGA_Stop"=TRUE) -> ("FPGA VI Reference Out"=w13:refnum<k20>, "error out"=w14:errorcluster)
  n1049 = xnode "Close FPGA VI Reference"("FPGA VI Reference In"=w13, "error in"=w14) -> ("error out"=w12:errorcluster)
  n1050 = call <vilib>:"Reset myRIO.vi"("error in (no error)"=w12) -> ()  [unwired: 10 in, 1 out]
